vi "btp_work.vi"() -> ()   [LabVIEW 2022 SP3]
uses:
  D:/LabVIEWCodes/USRPPacketTxRx/sub_Chop_Packet.vi
  D:/LabVIEWCodes/USRPPacketTxRx/sub_Ave_Power_And_Thresholding.vi
  D:/LabVIEWCodes/USRPPacketTxRx/sub_Extract_Packet_Boundaries - G.vi
  D:/LabVIEWCodes/USRPPacketTxRx/sub_Extract_Packets.vi
  <vilib>/addons/Modulation/Digital/General/MT Generate PSK System Parameters(M).vi
  <instrlib>/niUSRP/niUSRP Write Tx Data (CDB Cluster).vi
  <instrlib>/niUSRP/niUSRP Fetch Rx Data (CDB Cluster).vi
  D:/LabVIEWCodes/USRPPacketTxRx/subDCOffset.vi
  D:/LabVIEWCodes/USRPPacketTxRx/sub_est_noise_power - G1.vi
  <vilib>/addons/Modulation/niDMT.lvlib
panel:
  out "text 2":string
  out "text":string
  out "standard output 3":string
  out "standard output":string
  out "standard output 2":string
  in  "file (use dialog) 4":path
  in  "file (use dialog) 3":path
  out "standard error 3":string
  in  "file (use dialog) 2":path
  in  "file (use dialog)":path
  out "standard error 2":string
  out "standard error":string
  out "x .or. y?":bool
  in  "synchronization parameters":T1={"expected sync location (symbols)"=-1, "sync sequence"=[], "sync location uncertainty (symbols)"=0, "sync indent (symbols)"=0} {"sync sequence" format="%.2f"}
  in  "Tab Control":T2(tab)=enum."Rx Display"
  in  "Acquisition Duration [sec]":dbl=0.04 format="%#.6p"
  in  "Rx Parameters":T3={"Rx IQ Sampling\nRate [s/sec]"=500000.0, "Rx\nFrequency [Hz]"=915000000.0, "Rx Gain [dB]"=20.0, "Rx Antenna"="RX1"} {"Rx Gain [dB]" format="%#.6p"; "Rx\nFrequency [Hz]" format="%#.6p"; "Rx IQ Sampling\nRate [s/sec]" format="%#.6p"}
  out "Actual Rx Parameters":T3={"Rx IQ Sampling\nRate [s/sec]"=500000.0, "Rx\nFrequency [Hz]"=915000000.0, "Rx Gain [dB]"=20.0, "Rx Antenna"="RX1"} {"Rx Gain [dB]" format="%#.6p"; "Rx\nFrequency [Hz]" format="%#.6p"; "Rx IQ Sampling\nRate [s/sec]" format="%#.6p"}
  out "Symbol Rate\n[symbols/sec]":dbl=62500.0 format="%#.6p"
  in  "Choose a PSK Format":T4(tab)=enum."QPSK" caption="PSK"
  in  "BPSK System Parameters":T5={"Samples per Symbol"=8, "symbol map"=[], "Differential PSK"=enum."disable", "PSK type"=0} {"PSK type" items=["normal", "shifted", "offset"]; "symbol map" format="%.3f"}
  in  "QPSK System Parameters":T5={"Samples per Symbol"=8, "symbol map"=[], "Differential PSK"=enum."disable", "PSK type"=0} {"PSK type" items=["normal", "shifted", "offset"]; "symbol map" format="%.3f"}
  in  "pi/4 DQPSK System Parameters":T5={"Samples per Symbol"=8, "symbol map"=[], "Differential PSK"=enum."enable", "PSK type"=1} {"PSK type" items=["normal", "shifted", "offset"]; "symbol map" format="%.3f"}
  in  "OQPSK System Parameters":T5={"Samples per Symbol"=8, "symbol map"=[], "Differential PSK"=enum."disable", "PSK type"=2} {"PSK type" items=["normal", "shifted", "offset"]; "symbol map" format="%.3f"}
  in  "8-PSK System Parameters":T5={"Samples per Symbol"=8, "symbol map"=[], "Differential PSK"=enum."disable", "PSK type"=0} {"PSK type" items=["normal", "shifted", "offset"]; "symbol map" format="%.3f"}
  in  "16-PSK System Parameters":T5={"Samples per Symbol"=8, "symbol map"=[], "Differential PSK"=enum."disable", "PSK type"=0} {"PSK type" items=["normal", "shifted", "offset"]; "symbol map" format="%.3f"}
  in  "M":i32=4 min=2 step=2
  in  "Custom System Parameters":T5={"Samples per Symbol"=8, "symbol map"=[], "Differential PSK"=enum."disable", "PSK type"=0} {"PSK type" items=["normal", "shifted", "offset"]; "symbol map" format="%.3f"}
  in  "filter parameters":T6={"Alpha"=0.5, "Filter Length"=6, "TX Filter"=enum."Root Raised Cos"} caption="Matching Filter Parameters" {"Alpha" format="%.2f"}
  in  "PN Sequence Order\nfor Sync":i32=31
  in  "Packet Parameters":T7={"Guard Bits "=30, "Sync Bits"=20, "Message Bits"=128, "Number of Packets \nto Expect"=46}
  out "Recovered Message":string="Two roads diverged in a yellow wood,\nAnd sorry I could not travel both\nAnd be one traveler, long I stood\nAnd looked down one as far as I could\nTo where it bent in the undergrowth.\n\nThen took the other, as just as fair,\nAnd having perhaps the better claim,\nBecause it was grassy and wanted wear;\nThough as for that the passing there\nHad worn them really about the same.\n\nAnd both that morning equally lay\nIn leaves no step had trodden black.\nOh, I kept the first for another day!\nYet knowing how way leads on to way,\nI doubted if I should ever come back.\n\nI shall be telling this with a sigh\nSomewhere..."
  out "Received Signal (Raw)":dbl[](graph)
  out "Constellation Graph":T8(graph)=[{"Decimated Array"=[-0.6804993103727607, -0.6771092058245918, -0.6428257187708691, 0.7259219405542873, 0.7311366832454209, -0.6450362325295403, -0.658892442379921, -0.6855840493085356, -0.646998431742077, -0.6568678904388265, 0.7432214399633668, -0.6618522924674632, -0.6753922285302938, 0.6950905811428861, 0.7248141384495557, 0.7218255862492685, 0.704818637196686, 0.7027336696732543, 0.7016253671990413, 0.7082534735709545, 0.7084209330001522, 0.7036372125301554, 0.7010930640613204, 0.7075984577478206, 0.7100058187983528, 0.7171431626733421, 0.7279231861183771, 0.6959557947635676, -0.7024336186443912, -0.7110189818905128, 0.6934234462727887, 0.7327126116070742, 0.7051667045224878, 0.690798979580973, -0.6877839781333666, 0.6889445287579181, 0.716354235720989, -0.706071092371314, 0.72195318833854, -0.7119212984185137, 0.7223509528651848, -0.7244956435522718, -0.6716656585292338, -0.7182056308592257, 0.724421589775866, -0.6763390206227603, 0.7587597202334532, -0.6966306246608392, -0.6999692828092537, -0.7056805503027465, 0.7430994824068496, 0.7108305621069824, 0.7197425435843314, -0.7051937005816177, -0.6734048186040171, -0.6909214820858487, 0.7004218263991402, -0.6889802592692622, 0.7244882842042791, 0.7027757047403482, -0.7012448562483489, -0.6963431828766949, 0.7166197717755273, 0.7431431506248717, 0.7233235134334371, 0.6983161172439467, 0.7059749857271942, -0.6872358926309042, 0.6918268533027474, -0.7138701729016586, -0.6801285945135653, 0.7195044185357663, 0.6810587309328351, -0.6856313040037053, -0.7011043347997452, 0.6920652628903768, -0.7080955978852922, -0.6860253207439192, -0.7101309321759165, 0.7212965033681705, 0.6967245108747491, 0.7128097205123256, 0.6657328144726218, 0.6985573048815797, 0.6967609587320983, 0.720489591403177, -0.6992149062771553, 0.6810319795543738, -0.7124274384065621, -0.6689704942642202, 0.7017697482270308, 0.7036983705130238, -0.69378287602043, -0.6926507402482928, 0.6832891050414109, 0.7219614630178657, 0.7044242088089868, 0.6722056874933439, -0.6818156450864503, 0.6786113633855301, 0.7039257931121476, -0.6836867328922335, 0.6967676536286352, -0.7018627722542645, 0.7033449800412358, -0.7121625353086042], "Decimated Array"=[0.7327573786203745, 0.7417811878517194, -0.6799031648608087, -0.7111421642681004, -0.727382953469249, -0.6704579022356528, -0.6770604606987946, 0.7538529097411865, -0.6722715103438465, -0.6756211416707443, -0.6914774106844375, -0.673529581873597, 0.7393627898718214, 0.7522557788351737, 0.7435736461024193, 0.7257726558576425, 0.7275033865931528, 0.7311828384458046, 0.7293390182016347, 0.7220976758138733, 0.7195981106474233, 0.7211811690986409, 0.7188051788075457, 0.7320183145085448, 0.6962181897094762, 0.7305998791526044, -0.6967382767827438, 0.7159339540668409, -0.7008762468325049, 0.7525668303202456, 0.7058888207208955, 0.7252589385855543, -0.7159704258460882, 0.7370284868429373, 0.7140037167311404, 0.7389767670280546, -0.6960013467696725, 0.7235856630223708, -0.6972846806923089, -0.657884155216942, -0.6949224336608516, 0.7453870445521058, -0.6844918028247094, -0.6835224068604273, -0.7079388773369498, 0.7505384293302241, 0.6958348088594112, 0.7516973279064126, -0.6781015202421304, 0.7276930986154884, 0.7072095654921254, -0.6818066642899347, -0.702124108056222, 0.7365289833752492, 0.7313371097907961, 0.7586596196292686, -0.7079902911617727, 0.713630396728027, -0.7007240447824197, 0.7246614220304907, -0.7064584618733396, 0.7515472341269214, 0.6939391865838809, 0.7190183727683939, -0.6934598211856411, 0.7287398470888085, 0.7237013633767214, 0.7256529739097736, -0.6909901985488635, 0.7147604584382636, 0.6881560723752628, 0.7236976539802175, -0.6922424302133595, 0.7045483839307563, 0.6890103411064745, -0.6887965775506286, -0.7136342940914308, 0.7205719868506776, 0.7023916754066073, 0.7473081616445082, -0.6863264429683489, 0.7186091906642366, -0.7100679145508004, -0.6810878313976068, 0.7293932651728482, 0.722408788035578, 0.7004331018480651, -0.6822150791593455, 0.685337537979504, 0.7132682495621445, -0.6721281174161831, 0.7245443113283739, -0.7431160183824671, 0.7359349670621476, 0.7174344380700259, 0.7431105593701001, -0.6993804544754962, 0.7453566040596344, 0.6929469282521439, 0.7449696798222867, -0.693664788209523, 0.7157173189250563, -0.7183409139718169, -0.6991338441055578, -0.7093747657586275, 0.724868684652829]}, {"Decimated Array"=[-0.6804993103727607, -0.6762349965387238, -0.6685108157798112, -0.6587623289821404, -0.6494739544100483, -0.6438465750011458, -0.645155862498135, -0.6559333949667008, -0.6771092058245918, -0.707329395010057, -0.7427108893571827, -0.7768816274525345, -0.8016064503455926, -0.8078913118575249, -0.7873020181422804, -0.7333876332701184, -0.6428257187708691, -0.5161117575568228, -0.35777203758853365, -0.17570329650700167, 0.01987541369217473, 0.21778298257008183, 0.4072432109758152, 0.5789865397268567, 0.7259219405542873, 0.8433225109633283, 0.9285347773827741, 0.9803625623365572, 0.9983411710644498, 0.9823024312079763, 0.9321501534368272, 0.8480801425231922, 0.7311366832454209, 0.5839247754585907, 0.41126876723240074, 0.2204206478178329, 0.020932943403138903, -0.1761332529377578, -0.3593512576776315, -0.5183227318987554, -0.6450362325295403, -0.7348944300155227, -0.7873580245691122, -0.8057437870339258, -0.7965717988687436, -0.7684407927742708, -0.7306238606226202, -0.6917860656058442, -0.658892442379921, -0.6364690666334113, -0.6263656338128196, -0.6279033391241801, -0.6383295002999582, -0.6535857140497858, -0.6691389263327601, -0.6808303682804338, -0.6855840493085356, -0.6819546232796994, -0.6704727894453094, -0.6535744314745204, -0.6353365462635079, -0.6208696353048802, -0.6154307523642993, -0.6233724286798671, -0.646998431742077, -0.6855864576394015, -0.7347128803667217, -0.7860882541221362, -0.8282453730286534, -0.8479309126781169, -0.8321007406466316, -0.7702787309009056, -0.6568678904388265, -0.4928870454737699, -0.286812316855307, -0.054181947000257816, 0.18398541460571163, 0.403912791430555, 0.5822957160369652, 0.6996654194867074, 0.7432214399633668, 0.7085518372290116, 0.6001271112229511, 0.43028071322686884, 0.21712133759522834, -0.01828477060583316, -0.25486167705907176, -0.474106655260725, -0.6618522924674632, -0.8090041994597156, -0.9113555181844136, -0.9685514235160106, -0.9827395175415803, -0.9572113882143858, -0.8953875269303032, -0.8004356628744611, -0.6753922285302938, -0.5237515103490776, -0.3502005293644506, -0.1611351791820148, 0.03517140208780353, 0.22893110044459927, 0.40972263321669966, 0.5677345648283395, 0.6950905811428861, 0.7869683371034619, 0.8423038906676682, 0.8638849324516561, 0.8577538092414735, 0.8321468933549871, 0.7961070317612736, 0.7580880124868856, 0.7248141384495557, 0.7005277134039959, 0.686923334338586, 0.6833877232132058, 0.6876280888811944, 0.6964899036822818, 0.706747954834772, 0.7157647696850384, 0.7218255862492685, 0.724268969267967, 0.7234261321898535, 0.7202619630220548, 0.7159731242866095, 0.7116890979547664, 0.7082240869885714, 0.70594341514383, 0.704818637196686, 0.7045271958113069, 0.7047088927454438, 0.7050023859293303, 0.7051255773761397, 0.7049541452505861, 0.7044514570052206, 0.7036747950662702, 0.7027336696732543, 0.7017628701423971, 0.7009138948889888, 0.7003118882562483, 0.7000261021126073, 0.7000875017890581, 0.7004449481097869, 0.7009932809698078, 0.7016253671990413, 0.702221540251104, 0.7027618684813808, 0.7032916906181711, 0.7038854962099375, 0.7046487256800136, 0.7056308879137863, 0.7068515417419651, 0.7082534735709545, 0.7096888191782372, 0.7109913402244956, 0.7119894724643936, 0.7124890080936077, 0.7123827414517839, 0.7116323891766451, 0.7102633952930952, 0.7084209330001522, 0.7063057748688335, 0.7042562032788021, 0.7025954190884202, 0.7015546954049546, 0.7012557549487087, 0.7016448259380934, 0.7025398218482226, 0.7036372125301554, 0.7046321819639692, 0.7053295412842902, 0.7055972799037947, 0.705357986716468, 0.7046523984817116, 0.7036068751653552, 0.7023536981462808, 0.7010930640613204, 0.7000326295845363, 0.6993965049981011, 0.6993226127993213, 0.6998881120919372, 0.701113074412268, 0.7029138523453567, 0.7051416575412044, 0.7075984577478206, 0.710078980444559, 0.7123321038850414, 0.7140736603763724, 0.7150314533562983, 0.7150214932752349, 0.7140093308210059, 0.7121877418723002, 0.7100058187983528, 0.70805206355385, 0.7070027727419878, 0.7073212689161522, 0.7091056294101988, 0.7119833987327618, 0.7150644848824459, 0.7171668570713718, 0.7171431626733421, 0.71423133689185, 0.7085192919358748, 0.7011650150275229, 0.6943243914091253, 0.6909299894216554, 0.694045612210552, 0.706066960259486, 0.7279231861183771, 0.7583890909767882, 0.7938021658029275, 0.8279962238841705, 0.8528896550258644, 0.8595701988778817, 0.8395633321459017, 0.7862278633870129, 0.6959557947635676, 0.5689496495122442, 0.4094105630569515, 0.22502717825358973, 0.025894312218078558, -0.17672464042078925, -0.37176542586543576, -0.5495413422869474, -0.7024336186443912, -0.8251771287794907, -0.9146738107129905, -0.9693864660264264, -0.9886486884020281, -0.9721997012143947, -0.920010882437784, -0.8324905468768208, -0.7110189818905128, -0.5586215402038113, -0.38057133580870495, -0.18461757845785642, 0.019294891934465676, 0.2197963582992338, 0.4053691867674974, 0.5657713716359056, 0.6934234462727887, 0.7843501298361789, 0.8386729718179944, 0.8602628823550353, 0.855774513907276, 0.8333154686311419, 0.8010170366525857, 0.7658225991667146, 0.7327126116070742, 0.7045406905991981, 0.6824916000019303, 0.6667964864918056, 0.6575588911889615, 0.6553991485314229, 0.6616300661715835, 0.677865934701111, 0.7051667045224878, 0.7429233296416752, 0.7878677137961015, 0.8333853282559609, 0.8696348770191419, 0.8846190114381185, 0.8659756375138661, 0.8033400824826783, 0.690798979580973, 0.5288571353054295, 0.32551133007737276, 0.09595098720473762, -0.13906888290440567, -0.35588344294942403, -0.5312979803398246, -0.646084108275294, -0.6877839781333666, -0.6524636145322816, -0.5450893812430798, -0.37828756856953233, -0.17009276356333847, 0.0590247558982818, 0.28912715162217667, 0.5032762839933951, 0.6889445287579181, 0.8383428746399739, 0.9477025130341128, 1.015790170453614, 1.0423483901645878, 1.0268512388275022, 0.9680879161655901, 0.8646551393981081, 0.716354235720989, 0.5260764152807655, 0.30160439840294034, 0.05668512406955431, -0.18910351581760784, -0.4118751751084471, -0.5863423085037114, -0.6897554505434935, -0.706071092371314, -0.6295185621493208, -0.4668637151478481, -0.23765972556227086, 0.027714817455610417, 0.29202447870753795, 0.5167154122972588, 0.6679084709283569, 0.72195318833854, 0.6695114009171929, 0.5175155629675429, 0.2883041299697019, 0.01623720013151288, -0.25755900242514196, -0.4917082138253101, -0.6510176327160702, -0.7119212984185137, -0.6659995880876536, -0.5209852917537516, -0.2992839322286186, -0.03416997277404838, 0.2355466281568285, 0.4714352113659737, 0.6410442893752866, 0.7223509528651848, 0.7062991907811851, 0.5973003486423586, 0.4116890808688979, 0.17445466790696096, -0.08489625696410336, -0.3368901331962952, -0.5561324114364461, -0.7244956435522718, -0.832904063982776, -0.8817003370505312, -0.8795283892255058, -0.841156501109088, -0.7846263716950196, -0.7281214416972949, -0.6870445779683771, -0.6716656585292338, -0.6855631019709484, -0.7251869491105687, -0.7803544807713914, -0.8357414937022205, -0.8732615963603204, -0.8749681769421048, -0.8261602248386887, -0.7182056308592257, -0.5506938062457699, -0.3325933377055765, -0.08189760414583691, 0.17618237159000388, 0.4123697444728759, 0.5974694739328056, 0.7068084628379865, 0.724421589775866, 0.6461724854013321, 0.4812775786848407, 0.25159361606242997, -0.011058078343011023, -0.2692923486046545, -0.48569025029571594, -0.6284581525739953, -0.6763390206227603, -0.6219818356022658, -0.47306441806801147, -0.2510857990405568, 0.01202477775150253, 0.27875734553572085, 0.5116930035471384, 0.6789865139576629, 0.7587597202334532, 0.7418192787585248, 0.6323458533022597, 0.446406792743502, 0.20878035238051276, -0.05119783320575381, -0.3042611875270661, -0.5253152667965498, -0.6966306246608392, -0.8095606744479041, -0.8647740627418172, -0.870930075780708, -0.8423384959975685, -0.7960318277718325, -0.7486596019303445, -0.7137982795070836, -0.6999692828092537, -0.7095971091381883, -0.7390816485119921, -0.7796138336185289, -0.818762813999536, -0.8425904879324037, -0.8378822227707572, -0.7942341058424417, -0.7056805503027465, -0.571726769560303, -0.39765177441111643, -0.19391837432237818, 0.025178720377377686, 0.24333379676657457, 0.44433965307888695, 0.6142375047967751, 0.7430994824068496, 0.8263038750024307, 0.8650100488333368, 0.8657148042767202, 0.8390794723757462, 0.7981161813167071, 0.7560954579232749, 0.7244176046468488, 0.7108305621069824, 0.718204650734365, 0.7441150394580835, 0.7812106743682087, 0.8183931962770272, 0.8425254654823089, 0.8406177118076219, 0.8019301699596733, 0.7197425435843314, 0.5926686710089698, 0.4251140503775492, 0.22683136067452989, 0.011660330280988253, -0.20423795622266205, -0.4045792942890271, -0.57504838691632, -0.7051937005816177, -0.7897661684393493, -0.8293068652572223, -0.8299006515155186, -0.8021229049955473, -0.7594233513128958, -0.715953221878639, -0.684307426439313, -0.6734048186040171, -0.6868570522140265, -0.7221874426788824, -0.7708237442647581, -0.8191585903691571, -0.8505818015508355, -0.8481661462885941, -0.7977634650762118, -0.6909214820858487, -0.5271825682100394, -0.31525436879598623, -0.07267661804829456, 0.17610311762416703, 0.4028796348907104, 0.5798206568779839, 0.6838352068807156, 0.7004218263991402, 0.6263585027788804, 0.4707037347107586, 0.2537801245269521, 0.004363575376446024, -0.244425088845282, -0.45988451941533137, -0.6143614233710846, -0.6889802592692622, -0.675810131006379, -0.5782280367437729, -0.40962067096108434, -0.19054676255841746, 0.05481291967260732, 0.3023001215109928, 0.5308329677888366, 0.7244882842042791, 0.8734246012838044, 0.9735701497284382, 1.0253939516322779, 1.0322709072595566, 0.9989018615889086, 0.9300855209250758, 0.8301278260930205, 0.7027757047403482, 0.5516545283139476, 0.38091449347590134, 0.19570631362414656, 0.002354352790910658, -0.19179798997086855, -0.3788570549590451, -0.5510272450358933, -0.7012448562483489, -0.8236915392774603, -0.914039706142418, -0.9694184170252935, -0.9881756409826234, -0.9696303075716558, -0.913918517626886, -0.8220829857364051, -0.6963431828766949, -0.5405016807251724, -0.36031892603430715, -0.16359224329210514, 0.04013418091790215, 0.24018456190270834, 0.425760423266114, 0.5870829268985424, 0.7166197717755273, 0.8099833426954562, 0.8664917523906949, 0.8890606065456064, 0.8835329376488369, 0.8577948250420299, 0.8205354221662687, 0.7800304020582047, 0.7431431506248717, 0.7146443568705966, 0.6969512334183051, 0.6901074157262647, 0.6922880175560046, 0.7003398356906728, 0.7105226229352982, 0.7191652725013788, 0.7233235134334371, 0.7213381284523223, 0.7131072858574705, 0.7002046822080928, 0.6857438943908143, 0.6739876200747604, 0.6696394639541572, 0.6768836675096863, 0.6983161172439467, 0.7338690127516884, 0.7800774899548244, 0.829602819630056, 0.8715371312486556, 0.892620000492053, 0.8790856399483223, 0.8192212166031462, 0.7059749857271942, 0.5391749210900726, 0.3269503040314498, 0.08573815461541592, -0.1612255824786287, -0.386730293143399, -0.5635326559438285, -0.6686383256247854, -0.6872358926309042, -0.6156114857935734, -0.4623211423735695, -0.24733010394610414, 0.0007198102460047476, 0.24863863484628498, 0.4635514254715547, 0.6176104623364325, 0.6918268533027474, 0.6782756201030052, 0.5805134425392992, 0.41210610757403726, 0.19372452237290802, -0.050391409713054024, -0.29611210645789393, -0.5225111093000552, -0.7138701729016586, -0.8605441211993027, -0.9585448112667802, -1.008414026021156, -1.0135648241052666, -0.978745896542667, -0.9087849082692102, -0.8079881948321259, -0.6801285945135653, -0.5287862221062773, -0.35805233939202374, -0.1729861888667504, 0.020116186161511587, 0.21387335563181437, 0.40025748153323093, 0.5712472743319003, 0.7195044185357663, 0.8388895884119506, 0.9249072134737321, 0.9746853929178996, 0.9868923875604191, 0.9616684243967665, 0.9003848901697228, 0.8056175444681817, 0.6810587309328351, 0.5314881726723011, 0.3626554692436761, 0.18103860407685468, -0.006510589607727805, -0.1931114704827839, -0.3722848897831801, -0.5381718770034626, -0.6856313040037053, -0.8101801487665511, -0.9076732803716326, -0.9739618526107378, -1.004716020345832, -0.9956414793795033, -0.9430154749490675, -0.8446500281072215, -0.7011043347997452, -0.516842399364099, -0.3010204717594881, -0.06763754580789842, 0.16514820448340978, 0.37668157665933155, 0.5461920463765456, 0.655552915260347, 0.6920652628903768, 0.6505655304034257, 0.5346883243834851, 0.35661897243093144, 0.13559774776324776, -0.1046718797566402, -0.3394032573081613, -0.5461789593962133, -0.7080955978852922, -0.8157954529602021, -0.8683801331865292, -0.8727983131028657, -0.8421078226859732, -0.7927582081222804, -0.741572331068595, -0.7028423018527019, -0.6860253207439192, -0.6943551977069015, -0.7245345157854167, -0.7675646042411391, -0.8104296201087327, -0.8383601072014226, -0.8373952185694984, -0.7966528302359737, -0.7101309321759165, -0.5776984378988999, -0.40521323182553737, -0.2036592543667804, 0.012419924984258368, 0.22695341747885692, 0.42449093142276867, 0.592188438033417, 0.7212965033681705, 0.8079364234726191, 0.8532668165288172, 0.8627953034872611, 0.8451288060001957, 0.8104079963441455, 0.7687359339278867, 0.7287670505538517, 0.6967245108747491, 0.6759780606536095, 0.667107406232625, 0.6684364317450245, 0.676784919616326, 0.6884291860003884, 0.699890853611944, 0.7085144901744879, 0.7128097205123256, 0.7124229876828518, 0.7080187790236897, 0.7008050101089057, 0.6921805709227881, 0.6834646736814466, 0.6757033963031507, 0.669648508318143, 0.6657328144726218, 0.6642652636337992, 0.6653767657521718, 0.6690028595853793, 0.674775333959487, 0.6819477949985021, 0.6893278789128267, 0.6953927726157616, 0.6985573048815797, 0.697578095425808, 0.6920506573747554, 0.6828307951888688, 0.6722732265164824, 0.6640958466160822, 0.6627912256868634, 0.6726965874495441, 0.6967609587320983, 0.735252994349721, 0.7847852487718341, 0.837860611588047, 0.8832021671865116, 0.9070282265831913, 0.8950883370622812, 0.8352994933427401, 0.720489591403177, 0.5506306635171825, 0.3342725070105252, 0.08840692523651153, -0.16315427404215097, -0.3926718560799536, -0.572539734272038, -0.6796338477180948, -0.6992149062771553, -0.6277630208203462, -0.4741131473050659, -0.2585293695095081, -0.009930257048617025, 0.23830892263310452, 0.45325402085890604, 0.607121618765611, 0.6810319795543738, 0.6672310461853316, 0.5694827757707117, 0.4015147931896041, 0.1841817171712272, -0.05817646638242799, -0.3014136753019013, -0.524665532969832, -0.7124274384065621, -0.855285246094759, -0.9495933688767533, -0.996236130847489, -0.9989838487955423, -0.9628841324499167, -0.8930056180780918, -0.7937877561121499, -0.6689704942642202, -0.5220072798874036, -0.3566099133872175, -0.17731129436958973, 0.010268861422383327, 0.19945198638565087, 0.3827826926443024, 0.5526251582270405, 0.7017697482270308, 0.8239876507426606, 0.9144785689512498, 0.9699591512942685, 0.9886252045487814, 0.9700306803372667, 0.9149020439452162, 0.825116863065968, 0.7036983705130238, 0.554839481392563, 0.3840291620621759, 0.19787647745423148, 0.003860727052948984, -0.18999525295737457, -0.3757044734833313, -0.5458056810042837, -0.69378287602043, -0.814366828718361, -0.9036469275456485, -0.9588849469775574, -0.9783006504455267, -0.960973889608092, -0.9067746467203663, -0.8165903751017708, -0.6926507402482928, -0.5388812935652539, -0.361228905014989, -0.16771060388912773, 0.031903370124330505, 0.22678679843602859, 0.4061707941853134, 0.5606402717569381, 0.6832891050414109, 0.7705901219032752, 0.8228006526178891, 0.8436430103344122, 0.8394755303225311, 0.8180394512925253, 0.7871333265278456, 0.7534665911565442, 0.7219614630178657, 0.695510686451852, 0.6753252498343544, 0.6615878037807406, 0.6542998195364643, 0.6538606147644473, 0.6612723675386262, 0.6778625191525914, 0.7044242088089868, 0.7402649399766673, 0.7822594926239343, 0.8241634231439008, 0.8566831085547093, 0.8684082810681567, 0.8475040183712003, 0.784012885063017, 0.6722056874933439, 0.5125005393952523, 0.31260026449095785, 0.08722135068631567, -0.14339658857823498, -0.35611765704885123, -0.5282733760242059, -0.6409441045045646, -0.6818156450864503, -0.6469272017629891, -0.5410574986904879, -0.37652152921039295, -0.17097947697100876, 0.05541171165914345, 0.2829619347828144, 0.49484727767121917, 0.6786113633855301, 0.8264573551553331, 0.9345361200971587, 1.0015661687984379, 1.0272888190262575, 1.0112965146842847, 0.952583288738177, 0.8500890658990591, 0.7039257931121476, 0.5171900515296706, 0.29764273007471115, 0.05870661463653025, -0.1806017914741214, -0.39721826601913907, -0.5668036345777544, -0.6674573482841338, -0.6836867328922335, -0.6099467963750959, -0.4528161959244535, -0.23123780147788525, 0.0254037230819288, 0.2810884215045038, 0.4984727203603391, 0.6447055580185417, 0.6967676536286352, 0.6455398584402634, 0.4976568874522828, 0.2746594289249686, 0.009825427460916032, -0.25698435822392646, -0.4855514161032739, -0.6415528231225354, -0.7018627722542645, -0.6580125604775775, -0.517265265222927, -0.30121265695938104, -0.04212438479079229, 0.22217065809727116, 0.45405673442103006, 0.6217149465148919, 0.7033449800412358, 0.6897787566619501, 0.5850104229528822, 0.4047415306155254, 0.17323834921239678, -0.08075812096424864, -0.3284327261412435, -0.5448733152596168, -0.7121625353086042, -0.8211818337976253, -0.8719691969355644, -0.8727186157199347, -0.8376486334880819, -0.7842590106698991, -0.7303274268398209, -0.6909814362358659], "Decimated Array"=[0.7327573786203745, 0.8571160437398065, 0.9481227692632541, 1.003980881033979, 1.0238155370523472, 1.0072368286759465, 0.9541994905916551, 0.8651912730450063, 0.7417811878517194, 0.5871636451740783, 0.40676677760888635, 0.20846130324205578, 0.0022318875001048045, -0.2005410967663612, -0.38829860023304064, -0.5506845398656813, -0.6799031648608087, -0.7716987861234258, -0.8258475294329478, -0.8459996756657396, -0.8388616433189412, -0.8130753155007096, -0.7778435482452709, -0.7416372990136377, -0.7111421642681004, -0.6905831950739342, -0.6815454430666558, -0.6831516021872707, -0.6925669267273694, -0.7057731727702966, -0.7184007879882285, -0.7265282476091678, -0.727382953469249, -0.7198001905615271, -0.7045629848520147, -0.6843705475932246, -0.6634185556136458, -0.646887119577886, -0.6400361359583534, -0.6471594714631548, -0.6704579022356528, -0.7090564063186768, -0.7584053880552923, -0.8101244036157627, -0.8526189235085075, -0.872417498261418, -0.8561767863823757, -0.7930533916017833, -0.6770604606987946, -0.5089375701527854, -0.2971550620890392, -0.05761269204799846, 0.18789151496970918, 0.4143336303799478, 0.596919125262307, 0.7147087986695557, 0.7538529097411865, 0.7097353627437273, 0.5877778836770051, 0.40257278286196346, 0.1755748921605498, -0.06817834720063913, -0.30381917292160493, -0.5101473732591594, -0.6722715103438465, -0.782942771822579, -0.8426075541528982, -0.8581499860345086, -0.8406550377330191, -0.8028915815603971, -0.7569445207502417, -0.7124441110679234, -0.6756211416707443, -0.6492985792878058, -0.6336104831921037, -0.6270868628284776, -0.6278993868440812, -0.6347460148648578, -0.6473189374357599, -0.6660652122000107, -0.6914774106844375, -0.7231297220029862, -0.7587664029448702, -0.7936544758660282, -0.8205522923344901, -0.8305429506490288, -0.8142884856193261, -0.7636823212203829, -0.673529581873597, -0.5429181777841331, -0.3758793938755062, -0.18113858110834186, 0.028812354472331908, 0.23939310934756888, 0.4359274511900307, 0.6056519046787863, 0.7393627898718214, 0.8324327306148087, 0.8851319247653551, 0.9020886016493107, 0.8911142062914292, 0.8617307665544903, 0.8235701121823792, 0.7850172209229723, 0.7522557788351737, 0.7288635601528786, 0.7158958847588804, 0.7123277223581522, 0.715761845721655, 0.7231900323302534, 0.7316880970831603, 0.7389528359720056, 0.7435736461024193, 0.7451046063677472, 0.743901281226759, 0.740788821822152, 0.7367782401995692, 0.7328033193551644, 0.7294981194191762, 0.7271513904156902, 0.7257726558576425, 0.725159941446078, 0.725060989178965, 0.7252632377419967, 0.7256163395829798, 0.7260606904500417, 0.7265379023034586, 0.7270291732601397, 0.7275033865931528, 0.7279199682707127, 0.7282769079854728, 0.7285974590770533, 0.7289407767207793, 0.7293428506461535, 0.7298479408102396, 0.7304778513692572, 0.7311828384458046, 0.7318265401385785, 0.7323028750384627, 0.7325567749966301, 0.7325033028493253, 0.7321158823152807, 0.7314068004824351, 0.7304533892028899, 0.7293390182016347, 0.7281572743585262, 0.7270606197087242, 0.7261241067000211, 0.7253508195631971, 0.7246697616263047, 0.723969429286671, 0.723139564739256, 0.7220976758138733, 0.7208555865072881, 0.719568292828321, 0.7184478733558384, 0.7176993275862744, 0.7174622207349447, 0.7177521937986072, 0.718516228428159, 0.7195981106474233, 0.7207879819353863, 0.7218924194293399, 0.7227111613943498, 0.7231168859595661, 0.7230786498664554, 0.7226411424851807, 0.7219463720454906, 0.7211811690986409, 0.7204810710907097, 0.7199538718599565, 0.7196320372423504, 0.7194607411817737, 0.7193099127963588, 0.7190971249818399, 0.7188635612803779, 0.7188051788075457, 0.7192369464355841, 0.7205351477714964, 0.7229401499987833, 0.7263486481418566, 0.7301617369824043, 0.7333271712095472, 0.7344308070476105, 0.7320183145085448, 0.7250816880667706, 0.7135657369657201, 0.6987104127947069, 0.6831567860992641, 0.6708043964638186, 0.6662258399732381, 0.6737496016563864, 0.6962181897094762, 0.7338123953236427, 0.7831464621140352, 0.8367458472751513, 0.8833813981307604, 0.9091987678800104, 0.8998091259693833, 0.8428401153753142, 0.7305998791526044, 0.562507495226734, 0.34659814194077, 0.0995702257773744, -0.15462281131582128, -0.3875977492359962, -0.5706271624637833, -0.6790839949047796, -0.6967382767827438, -0.6189803271815245, -0.4544562375583789, -0.22459908414379984, 0.03903553601854455, 0.29916696405087967, 0.5182679460830586, 0.6643639077354586, 0.7159339540668409, 0.6652943920234429, 0.5198749673865217, 0.300993470244488, 0.04051717061424443, -0.22409581460784916, -0.45544556602126973, -0.6216785191074483, -0.7008762468325049, -0.6837610820977862, -0.5742886326760264, -0.3883111156265534, -0.1505286326662823, 0.10967239939698414, 0.3627475020866999, 0.5831487815378037, 0.7525668303202456, 0.8617987081334637, 0.9111768991603971, 0.9094611758407977, 0.8715862070139058, 0.8157455416667302, 0.760202018310825, 0.7202658930923688, 0.7058888207208955, 0.7201847936946834, 0.759052366114439, 0.811812333812609, 0.8630070563777121, 0.8948697888398245, 0.8903643946442023, 0.8361831300618912, 0.7252589385855543, 0.5584821670091451, 0.345315670477598, 0.10299763765352206, -0.14547539122840722, -0.37428698339337824, -0.5583637418127292, -0.6768312337753024, -0.7159704258460882, -0.6711625159308375, -0.5476542552431498, -0.3597709705436185, -0.1287724532856077, 0.12018518168690656, 0.36151984386717273, 0.572699142103299, 0.7370284868429373, 0.8455964386542135, 0.8979126579643226, 0.9012807607635166, 0.8690744380604796, 0.8181990426007191, 0.7661088030574076, 0.7279245613823432, 0.7140037167311404, 0.7282038712248695, 0.7671972819282604, 0.8208631561250372, 0.8738564756136162, 0.9080475656744531, 0.9055112204914009, 0.8518434216042863, 0.7389767670280546, 0.5673122043840576, 0.346672036977057, 0.09563946895916749, -0.1604955961723308, -0.3929887785452873, -0.573731438794397, -0.6795623772004052, -0.6960013467696725, -0.619916032405668, -0.46047605211853976, -0.238293779549608, 0.017302276506560462, 0.2723050965454336, 0.4928472153853533, 0.6499682346772773, 0.7235856630223708, 0.7050531042870595, 0.5980296925245243, 0.4173625434472803, 0.18635581949974522, -0.06697296685650257, -0.3141616680583659, -0.5303108718258116, -0.6972846806923089, -0.805693295562243, -0.8554610680619644, -0.8548810350527455, -0.8184903429533198, -0.7641725094683359, -0.7100008771843999, -0.671228658984871, -0.657884155216942, -0.6731679025330721, -0.7131015741595147, -0.7671687462263975, -0.8200654189127506, -0.8542004537564716, -0.8526249939936517, -0.8019646550151107, -0.6949224336608516, -0.5320250473508275, -0.32225185034324333, -0.08237582607009868, 0.1650026835738332, 0.39428466394542017, 0.5803342409591474, 0.7020686940954762, 0.7453870445521058, 0.7052505477960299, 0.5864589514160631, 0.40293010537214813, 0.17562748086081167, -0.0704552502607787, -0.309822690701368, -0.5200321703524325, -0.6844918028247094, -0.7944039739927944, -0.849369247148433, -0.856656043797114, -0.8292787623167311, -0.7833804658452638, -0.7353387812407823, -0.6989933350482087, -0.6835224068604273, -0.6921158238785066, -0.7217188264252835, -0.7637517506720419, -0.8057159017858148, -0.8333093620537693, -0.8327870038627241, -0.7931510688939891, -0.7079388773369498, -0.5762895149017982, -0.4032287101039275, -0.19912345762738048, 0.021626092972811716, 0.24243838454530214, 0.4466281803126936, 0.6195670275196116, 0.7505384293302241, 0.8341667424696944, 0.8710515511074273, 0.867618588313726, 0.8350546605288388, 0.7875968290108912, 0.7403153596554869, 0.7065887377614032, 0.6958348088594112, 0.7117510991794384, 0.7514265747295997, 0.8055501080993405, 0.8597172027233948, 0.896672112950365, 0.8992716440220376, 0.8535956532880161, 0.7516973279064126, 0.5935739768219647, 0.3879409425761628, 0.1514795080598367, -0.09323685375808283, -0.32079142716179476, -0.5065138588773618, -0.6300491223171335, -0.6781015202421304, -0.64619431762589, -0.5389832779795898, -0.36913308344851997, -0.15510153259215717, 0.08166236993095077, 0.3196509591252603, 0.5398927777919778, 0.7276930986154884, 0.8734985979773947, 0.9728047077610658, 1.0252642302363124, 1.0333899494712895, 1.0012329554745556, 0.9333027118497857, 0.8339401572384909, 0.7072095654921254, 0.5571462896311223, 0.3881483450425459, 0.20534155782487487, 0.01482887737245796, -0.1764521290488, -0.3611157500299354, -0.5318043493520626, -0.6818066642899347, -0.8054524101831724, -0.8983255342414102, -0.9572814410830893, -0.9802961943453828, -0.9661962276209902, -0.9145882909024544, -0.8259958203690237, -0.702124108056222, -0.5463111553516156, -0.3640099142702318, -0.1630068815984123, 0.04665386649189137, 0.25324056756651203, 0.4443960991039263, 0.6085609531447825, 0.7365289833752492, 0.8228996922007434, 0.8670933837874918, 0.8736111453366721, 0.8515289789816484, 0.8132403002190881, 0.772465080941647, 0.7419679771548864, 0.7313371097907961, 0.7450271466496866, 0.7811915546642222, 0.8315498322037654, 0.8823689588265033, 0.9165305921773814, 0.9163401501954511, 0.866798433796903, 0.7586596196292686, 0.5908492722170399, 0.37178062020046765, 0.11907890680745346, -0.14211821683680798, -0.38238233257874527, -0.5721392733995939, -0.6862057323913836, -0.7079902911617727, -0.6327143381258475, -0.4689575875843263, -0.23816585088733142, 0.02788728184520496, 0.2913733998865506, 0.5138745348418566, 0.6622161891528019, 0.713630396728027, 0.6595409016687056, 0.5072353110800646, 0.2790535214186103, 0.009173689804918802, -0.26151320666451255, -0.49168518087347146, -0.646028784822539, -0.7007240447824197, -0.6471884427151815, -0.493530539618674, -0.2632018631271933, 0.008643095196815533, 0.28067049342689865, 0.5117662020698565, 0.667360375596674, 0.7246614220304907, 0.6758948089830248, 0.5292499968474088, 0.30723953882700833, 0.04292589220225078, -0.22522884697938184, -0.4592044373314265, -0.6269083921942394, -0.7064584618733396, -0.6888404338934664, -0.578411648288706, -0.39139022626549447, -0.15271914914807735, 0.10811456934185323, 0.36154443524920665, 0.5821113615057549, 0.7515472341269214, 0.8606474547165524, 0.9096953707888916, 0.9073268916916939, 0.8684122594374747, 0.8110629523849187, 0.7535131577918508, 0.7111116174600383, 0.6939391865838809, 0.7053500144234236, 0.7415364458091326, 0.7922663020024436, 0.8425535702269459, 0.8751141872059586, 0.8732034679792344, 0.8235993150699542, 0.7190183727683939, 0.5598342988350936, 0.3547305255173707, 0.12000835651727722, -0.12227364288086777, -0.34712620885755746, -0.5299758484536152, -0.6500817333967435, -0.6934598211856411, -0.6548680069310724, -0.538631179832801, -0.35797405653961106, -0.13314154269390344, 0.11150249461783546, 0.3507932103438662, 0.5622006640712187, 0.7287398470888085, 0.8409123226340982, 0.8975410491756267, 0.9052474392037568, 0.8767801125750505, 0.8285828512227308, 0.7778392815717208, 0.7394654445105879, 0.7237013633767214, 0.7343864257619723, 0.7683602106205176, 0.8160146443370595, 0.862832671453382, 0.8918135732392275, 0.8863825849799384, 0.8334021521345413, 0.7256529739097736, 0.5635985512953553, 0.35608386653185525, 0.1195604135723027, -0.12374840459859741, -0.3487502236997944, -0.5308687349642771, -0.6495113130900928, -0.6909901985488635, -0.6504937240912037, -0.5328353201969774, -0.3517349807169625, -0.12783984379196844, 0.11423012543166067, 0.3492730631198282, 0.5549865684462535, 0.7147604584382636, 0.8196924285734603, 0.8692925730239803, 0.8708584840188425, 0.8377913064207088, 0.7870129074549828, 0.7359765930553231, 0.6996793525556969, 0.6881560723752628, 0.7048218776482567, 0.7458257319106636, 0.8006775631265496, 0.853917719961837, 0.8877440401214893, 0.8850693181898429, 0.8326613733709883, 0.7236976539802175, 0.5594490106415803, 0.3497538967519691, 0.11201578047048573, -0.13100695912350224, -0.3542636347146736, -0.5338912711941378, -0.6506028489493497, -0.6922424302133595, -0.6552909494544218, -0.545064832644278, -0.37448254797377645, -0.16191455440330382, 0.07162348789175096, 0.305307696187205, 0.5209397804835978, 0.7045483839307563, 0.8471495500869136, 0.9446334649114675, 0.9967359029755237, 1.0058177131022314, 0.9755714551521117, 0.910087443335543, 0.8133163625595331, 0.6890103411064745, 0.5410140712172831, 0.37367966894661164, 0.19222351735516607, 0.002885008671315868, -0.18723164421141011, -0.3706358231842831, -0.540017664941237, -0.6887965775506286, -0.811456181705438, -0.9037768968384509, -0.9627749707154154, -0.986428591882344, -0.9734798839005043, -0.9233425758887451, -0.8362626385273748, -0.7136342940914308, -0.5585921807071323, -0.37653877807456615, -0.17539608244694269, 0.03449829302119377, 0.24108409799518699, 0.4317114568156308, 0.5946337468390553, 0.7205719868506776, 0.8042233087437884, 0.8452649724027359, 0.8485537347599877, 0.8236121116636361, 0.7832470748996688, 0.7415340851598169, 0.7114139852567443, 0.7023916754066073, 0.7186444625002776, 0.7579146977658392, 0.8114788518364714, 0.865212362785649, 0.9017186145139675, 0.9031789704236397, 0.8546836474975438, 0.7473081616445082, 0.5805118731598218, 0.3633604703375262, 0.11403099657073672, -0.1421571689009856, -0.376100265224383, -0.5591208341865042, -0.66748156416295, -0.6863264429683489, -0.61238919788703, -0.45495950013783854, -0.2348765682622349, 0.018329318180048494, 0.27072256893627067, 0.4888669989484364, 0.6445441082266234, 0.7186091906642366, 0.7032516717681991, 0.602286440359839, 0.4297305321288512, 0.20693427048046936, -0.04118448970582595, -0.2899486028515708, -0.51813884111226, -0.7100679145508004, -0.8564812364022516, -0.954078154354838, -1.004051301932304, -1.0102212014763818, -0.9772535580383042, -0.9093646718646989, -0.8097976595431309, -0.6810878313976068, -0.5258335391357575, -0.34780340225624445, -0.15283789222057037, 0.05073422541995442, 0.25233190333965977, 0.44007238959276546, 0.6022906295601135, 0.7293932651728482, 0.8155001380288734, 0.8596440510683021, 0.8661244160018878, 0.8440053760191001, 0.8057116144877121, 0.7648934322393982, 0.7341019522530025, 0.722408788035578, 0.7335846743805764, 0.76523665163658, 0.8088069415554398, 0.8508057382972929, 0.8750784439185956, 0.8656525197192184, 0.8097364952043214, 0.7004331018480651, 0.5385134797346247, 0.333020638982082, 0.10055243220663874, -0.13684916712333142, -0.3547046170347631, -0.5296187059445376, -0.6427036804094352, -0.6822150791593455, -0.6450059416608724, -0.5366580259087476, -0.37013892662339776, -0.16344566761793425, 0.06325834047144631, 0.29051687792880865, 0.5019090102948002, 0.685337537979504, 0.8332571783100664, 0.9419059935710599, 1.0099338897337269, 1.0368536824281052, 1.0219112826998396, 0.9637216757298569, 0.8608644035958495, 0.7132682495621445, 0.5240958995354725, 0.30150783203128084, 0.05962244367312289, -0.18169903701790627, -0.3985650165893692, -0.5660874768283738, -0.6622779885806316, -0.6721281174161831, -0.5910217986061128, -0.4267122427659796, -0.19931344093386746, 0.06087906417721856, 0.31748163584889194, 0.5333437531858058, 0.6763479522156483, 0.7245443113283739, 0.6697558890344962, 0.5190710655465737, 0.2937181748767438, 0.02576020244976748, -0.24681249668741956, -0.4858948596428177, -0.6588635605451997, -0.7431160183824671, -0.7289134552508003, -0.6200694296515479, -0.4325067812603366, -0.19121024572221312, 0.07400166309693594, 0.3330849816678037, 0.5599873834891823, 0.7359349670621476, 0.8513661111199331, 0.9063246869034065, 0.9094064046484032, 0.8755054075051303, 0.8228032542069148, 0.7695512733800192, 0.7310864566365781, 0.7174344380700259, 0.7318771929311987, 0.770521492507058, 0.8229990169861556, 0.8741669857800006, 0.9065945000702298, 0.9034290410951017, 0.8513488075060012, 0.7431105593701001, 0.5792771762670239, 0.3688585907869233, 0.12855873457058717, -0.11905374155741394, -0.348465451110149, -0.5346000660767498, -0.6563026294503328, -0.6993804544754962, -0.6586232637177873, -0.5386587210945445, -0.35325412329016936, -0.12340944757935825, 0.12562838916868907, 0.3678984527083349, 0.5802535686096911, 0.7453566040596344, 0.8536797217461267, 0.904341743696613, 0.9045288934223483, 0.8678005605218305, 0.8115232656672823, 0.7538338251356304, 0.7106289265654393, 0.6929469282521439, 0.7051665302164144, 0.7441987520198292, 0.7999632255413621, 0.8568697593576841, 0.8963183241181077, 0.8998019936252488, 0.8522424023181564, 0.7449696798222867, 0.5778551163588856, 0.3603125530553699, 0.11070054945898282, -0.14570230635299203, -0.3799809948767624, -0.5637043781173343, -0.6732548027150764, -0.693664788209523, -0.6213306289901542, -0.46505052769065697, -0.24516543111583403, 0.0090596915946915, 0.2635428251223252, 0.48417637041829653, 0.641689526437302, 0.7157173189250563, 0.6973828411174359, 0.5901314098610099, 0.4086428546496129, 0.17619718572689294, -0.07917988137166046, -0.328937783780878, -0.5480728892646238, -0.7183409139718169, -0.830216292312652, -0.8834929518448947, -0.8862829283786646, -0.8529835994516479, -0.8013536812216641, -0.7493136237212195, -0.711957955660661, -0.6991338441055578, -0.7139427031909754, -0.7523268372875261, -0.8037761996631599, -0.8530893578229929, -0.8828792296977179, -0.8764987725251604, -0.8209490836280732, -0.7093747657586275, -0.5427215391631399, -0.33033331822457584, -0.08916763854378294, 0.15803966171501063, 0.3856904000524847, 0.5687642313471672, 0.6864040238926279, 0.724868684652829, 0.6795420414253549, 0.5557211678730963, 0.3677696222282419, 0.13706564016321376, -0.11113892216576668, -0.3513165038596046, -0.5611655218564168]}]
  out "Sync Found":bool=TRUE
  out "Correct Packets Rx":i16=46
  out "Singal & Noise Power":cluster{"signal_power":dbl, "noise_power":dbl}={"signal_power"=0.000719802679436105, "noise_power"=8.71918670194843e-09}
  out "error out":errorcluster
  out "Cumulative Packets Recovered":i16(graph)=46
  out "Signal and Noise Power Tracking":cluster{"total_power":dbl, "noise_power":dbl}(graph)={"total_power"=0.000719802679436105, "noise_power"=8.71918670194843e-09}
  in  "stop":bool
  out "Symbol Rate\n[symbols/sec] 2":dbl=25000.0 format="%#.6p"
  out "Constellation Graph 2":T8(graph) caption="Constellation Graph"
  in  "autoscale":bool
  in  "Tab Control 2":T9(tab)
  in  "Packet Parameters 2":T10={"Guard Bits "=30, "Sync Bits"=20, "Message Bits"=128}
  in  "Packet Pad \n[samples]":i32=200
  in  "Blank Frame \n[samples]":i32=500
  out "Number of Packets in Message":i32=46
  in  "PN sequence order\nfor Sync Bits":i32=31 caption="PN sequence order (9)"
  in  "Packet Repeat":i32=2
  in  "Select PSK Modulation Format":T4(tab)=enum."QPSK" caption="PSK"
  in  "BPSK System Parameters 2":T5={"Samples per Symbol"=8, "symbol map"=[], "Differential PSK"=enum."disable", "PSK type"=0} caption="BPSK System Parameters" {"PSK type" items=["normal", "shifted", "offset"]; "symbol map" format="%.3f"}
  in  "QPSK System Parameters 2":T5={"Samples per Symbol"=8, "symbol map"=[], "Differential PSK"=enum."disable", "PSK type"=0} caption="QPSK System Parameters" {"PSK type" items=["normal", "shifted", "offset"]; "symbol map" format="%.3f"}
  in  "pi/4 DQPSK System Parameters 2":T5={"Samples per Symbol"=8, "symbol map"=[], "Differential PSK"=enum."enable", "PSK type"=1} caption="pi/4 DQPSK System Parameters" {"PSK type" items=["normal", "shifted", "offset"]; "symbol map" format="%.3f"}
  in  "OQPSK System Parameters 2":T5={"Samples per Symbol"=8, "symbol map"=[], "Differential PSK"=enum."disable", "PSK type"=2} caption="OQPSK System Parameters" {"PSK type" items=["normal", "shifted", "offset"]; "symbol map" format="%.3f"}
  in  "8-PSK System Parameters 2":T5={"Samples per Symbol"=8, "symbol map"=[], "Differential PSK"=enum."disable", "PSK type"=0} caption="8-PSK System Parameters" {"PSK type" items=["normal", "shifted", "offset"]; "symbol map" format="%.3f"}
  in  "16-PSK System Parameters 2":T5={"Samples per Symbol"=8, "symbol map"=[], "Differential PSK"=enum."disable", "PSK type"=0} caption="16-PSK System Parameters" {"PSK type" items=["normal", "shifted", "offset"]; "symbol map" format="%.3f"}
  in  "M 2":i32=4 caption="M" min=2 step=2
  in  "Custom System Parameters 2":T5={"Samples per Symbol"=8, "symbol map"=[], "Differential PSK"=enum."disable", "PSK type"=0} caption="Custom System Parameters" {"PSK type" items=["normal", "shifted", "offset"]; "symbol map" format="%.3f"}
  in  "Pulse Shaping Filter Parameters":T6={"Alpha"=0.5, "Filter Length"=6, "TX Filter"=enum."Root Raised Cos"} caption="Pulse Shaping Filter" {"Alpha" format="%.2f"}
  in  "Tx Parameters":T11={"Tx IQ Sampling\nRate [s/sec]"=500000.0, "Tx Frequency [Hz]"=2500000000.0, "Tx Gain [dB]"=0.0, "Tx Antenna"="TX1"} {"Tx Gain [dB]" format="%#.6p"; "Tx Frequency [Hz]" format="%#.6p"; "Tx IQ Sampling\nRate [s/sec]" format="%#.6p"}
  out "Actual Tx Parameters":T11={"Tx IQ Sampling\nRate [s/sec]"=200000.0, "Tx Frequency [Hz]"=2500000000.0, "Tx Gain [dB]"=0.0, "Tx Antenna"="TX1"} {"Tx Gain [dB]" format="%#.6p"; "Tx Frequency [Hz]" format="%#.6p"; "Tx IQ Sampling\nRate [s/sec]" format="%#.6p"}
  out "error out 2":errorcluster
  in  "Queue Length":i32=10
  in  "stop 3":bool caption="stop"
  out "Symbol Rate\n[symbols/sec] 5":dbl=25000.0 format="%#.6p"
  out "Constellation Graph 5":T8(graph) caption="Constellation Graph"
  in  "autoscale 3":bool caption="autoscale"
  in  "Tab Control 5":T9(tab)
  in  "Packet Parameters 5":T10={"Guard Bits "=30, "Sync Bits"=20, "Message Bits"=128}
  in  "Packet Pad \n[samples] 3":i32=200
  in  "Blank Frame \n[samples] 3":i32=500
  out "Number of Packets in Message 3":i32=46
  in  "PN sequence order\nfor Sync Bits 3":i32=31 caption="PN sequence order (9)"
  in  "Packet Repeat 3":i32=2
  in  "Select PSK Modulation Format 3":T4(tab)=enum."QPSK" caption="PSK"
  in  "BPSK System Parameters 5":T5={"Samples per Symbol"=8, "symbol map"=[], "Differential PSK"=enum."disable", "PSK type"=0} caption="BPSK System Parameters" {"PSK type" items=["normal", "shifted", "offset"]; "symbol map" format="%.3f"}
  in  "QPSK System Parameters 5":T5={"Samples per Symbol"=8, "symbol map"=[], "Differential PSK"=enum."disable", "PSK type"=0} caption="QPSK System Parameters" {"PSK type" items=["normal", "shifted", "offset"]; "symbol map" format="%.3f"}
  in  "pi/4 DQPSK System Parameters 5":T5={"Samples per Symbol"=8, "symbol map"=[], "Differential PSK"=enum."enable", "PSK type"=1} caption="pi/4 DQPSK System Parameters" {"PSK type" items=["normal", "shifted", "offset"]; "symbol map" format="%.3f"}
  in  "OQPSK System Parameters 5":T5={"Samples per Symbol"=8, "symbol map"=[], "Differential PSK"=enum."disable", "PSK type"=2} caption="OQPSK System Parameters" {"PSK type" items=["normal", "shifted", "offset"]; "symbol map" format="%.3f"}
  in  "8-PSK System Parameters 5":T5={"Samples per Symbol"=8, "symbol map"=[], "Differential PSK"=enum."disable", "PSK type"=0} caption="8-PSK System Parameters" {"PSK type" items=["normal", "shifted", "offset"]; "symbol map" format="%.3f"}
  in  "16-PSK System Parameters 5":T5={"Samples per Symbol"=8, "symbol map"=[], "Differential PSK"=enum."disable", "PSK type"=0} caption="16-PSK System Parameters" {"PSK type" items=["normal", "shifted", "offset"]; "symbol map" format="%.3f"}
  in  "M 5":i32=4 caption="M" min=2 step=2
  in  "Custom System Parameters 5":T5={"Samples per Symbol"=8, "symbol map"=[], "Differential PSK"=enum."disable", "PSK type"=0} caption="Custom System Parameters" {"PSK type" items=["normal", "shifted", "offset"]; "symbol map" format="%.3f"}
  in  "Pulse Shaping Filter Parameters 3":T6={"Alpha"=0.5, "Filter Length"=6, "TX Filter"=enum."Root Raised Cos"} caption="Pulse Shaping Filter" {"Alpha" format="%.2f"}
  in  "Tx Parameters 3":T11={"Tx IQ Sampling\nRate [s/sec]"=500000.0, "Tx Frequency [Hz]"=2500000000.0, "Tx Gain [dB]"=0.0, "Tx Antenna"="TX1"} {"Tx Gain [dB]" format="%#.6p"; "Tx Frequency [Hz]" format="%#.6p"; "Tx IQ Sampling\nRate [s/sec]" format="%#.6p"}
  out "Actual Tx Parameters 3":T11={"Tx IQ Sampling\nRate [s/sec]"=200000.0, "Tx Frequency [Hz]"=2500000000.0, "Tx Gain [dB]"=0.0, "Tx Antenna"="TX1"} {"Tx Gain [dB]" format="%#.6p"; "Tx Frequency [Hz]" format="%#.6p"; "Tx IQ Sampling\nRate [s/sec]" format="%#.6p"}
  out "error out 5":errorcluster
  in  "Queue Length 3":i32=10
  out "x .or. y? 6":bool
  in  "synchronization parameters 4":T1={"expected sync location (symbols)"=-1, "sync sequence"=[], "sync location uncertainty (symbols)"=0, "sync indent (symbols)"=0} caption="synchronization parameters" {"sync sequence" format="%.2f"}
  in  "Tab Control 7":T2(tab)=enum."Rx Display"
  in  "Acquisition Duration [sec] 4":dbl=0.04 format="%#.6p"
  in  "Rx Parameters 4":T3={"Rx IQ Sampling\nRate [s/sec]"=500000.0, "Rx\nFrequency [Hz]"=915000000.0, "Rx Gain [dB]"=20.0, "Rx Antenna"="RX1"} {"Rx Gain [dB]" format="%#.6p"; "Rx\nFrequency [Hz]" format="%#.6p"; "Rx IQ Sampling\nRate [s/sec]" format="%#.6p"}
  out "Actual Rx Parameters  4":T3={"Rx IQ Sampling\nRate [s/sec]"=500000.0, "Rx\nFrequency [Hz]"=915000000.0, "Rx Gain [dB]"=20.0, "Rx Antenna"="RX1"} {"Rx Gain [dB]" format="%#.6p"; "Rx\nFrequency [Hz]" format="%#.6p"; "Rx IQ Sampling\nRate [s/sec]" format="%#.6p"}
  out "Symbol Rate\n[symbols/sec] 7":dbl=62500.0 format="%#.6p"
  in  "Choose a PSK Format 4":T4(tab)=enum."QPSK" caption="PSK"
  in  "BPSK System Parameters 7":T5={"Samples per Symbol"=8, "symbol map"=[], "Differential PSK"=enum."disable", "PSK type"=0} caption="BPSK System Parameters" {"PSK type" items=["normal", "shifted", "offset"]; "symbol map" format="%.3f"}
  in  "QPSK System Parameters 7":T5={"Samples per Symbol"=8, "symbol map"=[], "Differential PSK"=enum."disable", "PSK type"=0} caption="QPSK System Parameters" {"PSK type" items=["normal", "shifted", "offset"]; "symbol map" format="%.3f"}
  in  "pi/4 DQPSK System Parameters 7":T5={"Samples per Symbol"=8, "symbol map"=[], "Differential PSK"=enum."enable", "PSK type"=1} caption="pi/4 DQPSK System Parameters" {"PSK type" items=["normal", "shifted", "offset"]; "symbol map" format="%.3f"}
  in  "OQPSK System Parameters 7":T5={"Samples per Symbol"=8, "symbol map"=[], "Differential PSK"=enum."disable", "PSK type"=2} caption="OQPSK System Parameters" {"PSK type" items=["normal", "shifted", "offset"]; "symbol map" format="%.3f"}
  in  "8-PSK System Parameters 7":T5={"Samples per Symbol"=8, "symbol map"=[], "Differential PSK"=enum."disable", "PSK type"=0} caption="8-PSK System Parameters" {"PSK type" items=["normal", "shifted", "offset"]; "symbol map" format="%.3f"}
  in  "16-PSK System Parameters 7":T5={"Samples per Symbol"=8, "symbol map"=[], "Differential PSK"=enum."disable", "PSK type"=0} caption="16-PSK System Parameters" {"PSK type" items=["normal", "shifted", "offset"]; "symbol map" format="%.3f"}
  in  "M 7":i32=4 caption="M" min=2 step=2
  in  "Custom System Parameters 7":T5={"Samples per Symbol"=8, "symbol map"=[], "Differential PSK"=enum."disable", "PSK type"=0} caption="Custom System Parameters" {"PSK type" items=["normal", "shifted", "offset"]; "symbol map" format="%.3f"}
  in  "filter parameters 4":T6={"Alpha"=0.5, "Filter Length"=6, "TX Filter"=enum."Root Raised Cos"} caption="Matching Filter Parameters" {"Alpha" format="%.2f"}
  in  "PN Sequence Order\nfor Sync 4":i32=31
  in  "Packet Parameters 7":T7={"Guard Bits "=30, "Sync Bits"=20, "Message Bits"=128, "Number of Packets \nto Expect"=46}
  out "Recovered Message 4":string="Two roads diverged in a yellow wood,\nAnd sorry I could not travel both\nAnd be one traveler, long I stood\nAnd looked down one as far as I could\nTo where it bent in the undergrowth.\n\nThen took the other, as just as fair,\nAnd having perhaps the better claim,\nBecause it was grassy and wanted wear;\nThough as for that the passing there\nHad worn them really about the same.\n\nAnd both that morning equally lay\nIn leaves no step had trodden black.\nOh, I kept the first for another day!\nYet knowing how way leads on to way,\nI doubted if I should ever come back.\n\nI shall be telling this with a sigh\nSomewhere..."
  out "Received Signal (Raw) 4":dbl[](graph)
  out "Constellation Graph 7":T8(graph)=[{"Decimated Array"=[-0.6804993103727607, -0.6771092058245918, -0.6428257187708691, 0.7259219405542873, 0.7311366832454209, -0.6450362325295403, -0.658892442379921, -0.6855840493085356, -0.646998431742077, -0.6568678904388265, 0.7432214399633668, -0.6618522924674632, -0.6753922285302938, 0.6950905811428861, 0.7248141384495557, 0.7218255862492685, 0.704818637196686, 0.7027336696732543, 0.7016253671990413, 0.7082534735709545, 0.7084209330001522, 0.7036372125301554, 0.7010930640613204, 0.7075984577478206, 0.7100058187983528, 0.7171431626733421, 0.7279231861183771, 0.6959557947635676, -0.7024336186443912, -0.7110189818905128, 0.6934234462727887, 0.7327126116070742, 0.7051667045224878, 0.690798979580973, -0.6877839781333666, 0.6889445287579181, 0.716354235720989, -0.706071092371314, 0.72195318833854, -0.7119212984185137, 0.7223509528651848, -0.7244956435522718, -0.6716656585292338, -0.7182056308592257, 0.724421589775866, -0.6763390206227603, 0.7587597202334532, -0.6966306246608392, -0.6999692828092537, -0.7056805503027465, 0.7430994824068496, 0.7108305621069824, 0.7197425435843314, -0.7051937005816177, -0.6734048186040171, -0.6909214820858487, 0.7004218263991402, -0.6889802592692622, 0.7244882842042791, 0.7027757047403482, -0.7012448562483489, -0.6963431828766949, 0.7166197717755273, 0.7431431506248717, 0.7233235134334371, 0.6983161172439467, 0.7059749857271942, -0.6872358926309042, 0.6918268533027474, -0.7138701729016586, -0.6801285945135653, 0.7195044185357663, 0.6810587309328351, -0.6856313040037053, -0.7011043347997452, 0.6920652628903768, -0.7080955978852922, -0.6860253207439192, -0.7101309321759165, 0.7212965033681705, 0.6967245108747491, 0.7128097205123256, 0.6657328144726218, 0.6985573048815797, 0.6967609587320983, 0.720489591403177, -0.6992149062771553, 0.6810319795543738, -0.7124274384065621, -0.6689704942642202, 0.7017697482270308, 0.7036983705130238, -0.69378287602043, -0.6926507402482928, 0.6832891050414109, 0.7219614630178657, 0.7044242088089868, 0.6722056874933439, -0.6818156450864503, 0.6786113633855301, 0.7039257931121476, -0.6836867328922335, 0.6967676536286352, -0.7018627722542645, 0.7033449800412358, -0.7121625353086042], "Decimated Array"=[0.7327573786203745, 0.7417811878517194, -0.6799031648608087, -0.7111421642681004, -0.727382953469249, -0.6704579022356528, -0.6770604606987946, 0.7538529097411865, -0.6722715103438465, -0.6756211416707443, -0.6914774106844375, -0.673529581873597, 0.7393627898718214, 0.7522557788351737, 0.7435736461024193, 0.7257726558576425, 0.7275033865931528, 0.7311828384458046, 0.7293390182016347, 0.7220976758138733, 0.7195981106474233, 0.7211811690986409, 0.7188051788075457, 0.7320183145085448, 0.6962181897094762, 0.7305998791526044, -0.6967382767827438, 0.7159339540668409, -0.7008762468325049, 0.7525668303202456, 0.7058888207208955, 0.7252589385855543, -0.7159704258460882, 0.7370284868429373, 0.7140037167311404, 0.7389767670280546, -0.6960013467696725, 0.7235856630223708, -0.6972846806923089, -0.657884155216942, -0.6949224336608516, 0.7453870445521058, -0.6844918028247094, -0.6835224068604273, -0.7079388773369498, 0.7505384293302241, 0.6958348088594112, 0.7516973279064126, -0.6781015202421304, 0.7276930986154884, 0.7072095654921254, -0.6818066642899347, -0.702124108056222, 0.7365289833752492, 0.7313371097907961, 0.7586596196292686, -0.7079902911617727, 0.713630396728027, -0.7007240447824197, 0.7246614220304907, -0.7064584618733396, 0.7515472341269214, 0.6939391865838809, 0.7190183727683939, -0.6934598211856411, 0.7287398470888085, 0.7237013633767214, 0.7256529739097736, -0.6909901985488635, 0.7147604584382636, 0.6881560723752628, 0.7236976539802175, -0.6922424302133595, 0.7045483839307563, 0.6890103411064745, -0.6887965775506286, -0.7136342940914308, 0.7205719868506776, 0.7023916754066073, 0.7473081616445082, -0.6863264429683489, 0.7186091906642366, -0.7100679145508004, -0.6810878313976068, 0.7293932651728482, 0.722408788035578, 0.7004331018480651, -0.6822150791593455, 0.685337537979504, 0.7132682495621445, -0.6721281174161831, 0.7245443113283739, -0.7431160183824671, 0.7359349670621476, 0.7174344380700259, 0.7431105593701001, -0.6993804544754962, 0.7453566040596344, 0.6929469282521439, 0.7449696798222867, -0.693664788209523, 0.7157173189250563, -0.7183409139718169, -0.6991338441055578, -0.7093747657586275, 0.724868684652829]}, {"Decimated Array"=[-0.6804993103727607, -0.6762349965387238, -0.6685108157798112, -0.6587623289821404, -0.6494739544100483, -0.6438465750011458, -0.645155862498135, -0.6559333949667008, -0.6771092058245918, -0.707329395010057, -0.7427108893571827, -0.7768816274525345, -0.8016064503455926, -0.8078913118575249, -0.7873020181422804, -0.7333876332701184, -0.6428257187708691, -0.5161117575568228, -0.35777203758853365, -0.17570329650700167, 0.01987541369217473, 0.21778298257008183, 0.4072432109758152, 0.5789865397268567, 0.7259219405542873, 0.8433225109633283, 0.9285347773827741, 0.9803625623365572, 0.9983411710644498, 0.9823024312079763, 0.9321501534368272, 0.8480801425231922, 0.7311366832454209, 0.5839247754585907, 0.41126876723240074, 0.2204206478178329, 0.020932943403138903, -0.1761332529377578, -0.3593512576776315, -0.5183227318987554, -0.6450362325295403, -0.7348944300155227, -0.7873580245691122, -0.8057437870339258, -0.7965717988687436, -0.7684407927742708, -0.7306238606226202, -0.6917860656058442, -0.658892442379921, -0.6364690666334113, -0.6263656338128196, -0.6279033391241801, -0.6383295002999582, -0.6535857140497858, -0.6691389263327601, -0.6808303682804338, -0.6855840493085356, -0.6819546232796994, -0.6704727894453094, -0.6535744314745204, -0.6353365462635079, -0.6208696353048802, -0.6154307523642993, -0.6233724286798671, -0.646998431742077, -0.6855864576394015, -0.7347128803667217, -0.7860882541221362, -0.8282453730286534, -0.8479309126781169, -0.8321007406466316, -0.7702787309009056, -0.6568678904388265, -0.4928870454737699, -0.286812316855307, -0.054181947000257816, 0.18398541460571163, 0.403912791430555, 0.5822957160369652, 0.6996654194867074, 0.7432214399633668, 0.7085518372290116, 0.6001271112229511, 0.43028071322686884, 0.21712133759522834, -0.01828477060583316, -0.25486167705907176, -0.474106655260725, -0.6618522924674632, -0.8090041994597156, -0.9113555181844136, -0.9685514235160106, -0.9827395175415803, -0.9572113882143858, -0.8953875269303032, -0.8004356628744611, -0.6753922285302938, -0.5237515103490776, -0.3502005293644506, -0.1611351791820148, 0.03517140208780353, 0.22893110044459927, 0.40972263321669966, 0.5677345648283395, 0.6950905811428861, 0.7869683371034619, 0.8423038906676682, 0.8638849324516561, 0.8577538092414735, 0.8321468933549871, 0.7961070317612736, 0.7580880124868856, 0.7248141384495557, 0.7005277134039959, 0.686923334338586, 0.6833877232132058, 0.6876280888811944, 0.6964899036822818, 0.706747954834772, 0.7157647696850384, 0.7218255862492685, 0.724268969267967, 0.7234261321898535, 0.7202619630220548, 0.7159731242866095, 0.7116890979547664, 0.7082240869885714, 0.70594341514383, 0.704818637196686, 0.7045271958113069, 0.7047088927454438, 0.7050023859293303, 0.7051255773761397, 0.7049541452505861, 0.7044514570052206, 0.7036747950662702, 0.7027336696732543, 0.7017628701423971, 0.7009138948889888, 0.7003118882562483, 0.7000261021126073, 0.7000875017890581, 0.7004449481097869, 0.7009932809698078, 0.7016253671990413, 0.702221540251104, 0.7027618684813808, 0.7032916906181711, 0.7038854962099375, 0.7046487256800136, 0.7056308879137863, 0.7068515417419651, 0.7082534735709545, 0.7096888191782372, 0.7109913402244956, 0.7119894724643936, 0.7124890080936077, 0.7123827414517839, 0.7116323891766451, 0.7102633952930952, 0.7084209330001522, 0.7063057748688335, 0.7042562032788021, 0.7025954190884202, 0.7015546954049546, 0.7012557549487087, 0.7016448259380934, 0.7025398218482226, 0.7036372125301554, 0.7046321819639692, 0.7053295412842902, 0.7055972799037947, 0.705357986716468, 0.7046523984817116, 0.7036068751653552, 0.7023536981462808, 0.7010930640613204, 0.7000326295845363, 0.6993965049981011, 0.6993226127993213, 0.6998881120919372, 0.701113074412268, 0.7029138523453567, 0.7051416575412044, 0.7075984577478206, 0.710078980444559, 0.7123321038850414, 0.7140736603763724, 0.7150314533562983, 0.7150214932752349, 0.7140093308210059, 0.7121877418723002, 0.7100058187983528, 0.70805206355385, 0.7070027727419878, 0.7073212689161522, 0.7091056294101988, 0.7119833987327618, 0.7150644848824459, 0.7171668570713718, 0.7171431626733421, 0.71423133689185, 0.7085192919358748, 0.7011650150275229, 0.6943243914091253, 0.6909299894216554, 0.694045612210552, 0.706066960259486, 0.7279231861183771, 0.7583890909767882, 0.7938021658029275, 0.8279962238841705, 0.8528896550258644, 0.8595701988778817, 0.8395633321459017, 0.7862278633870129, 0.6959557947635676, 0.5689496495122442, 0.4094105630569515, 0.22502717825358973, 0.025894312218078558, -0.17672464042078925, -0.37176542586543576, -0.5495413422869474, -0.7024336186443912, -0.8251771287794907, -0.9146738107129905, -0.9693864660264264, -0.9886486884020281, -0.9721997012143947, -0.920010882437784, -0.8324905468768208, -0.7110189818905128, -0.5586215402038113, -0.38057133580870495, -0.18461757845785642, 0.019294891934465676, 0.2197963582992338, 0.4053691867674974, 0.5657713716359056, 0.6934234462727887, 0.7843501298361789, 0.8386729718179944, 0.8602628823550353, 0.855774513907276, 0.8333154686311419, 0.8010170366525857, 0.7658225991667146, 0.7327126116070742, 0.7045406905991981, 0.6824916000019303, 0.6667964864918056, 0.6575588911889615, 0.6553991485314229, 0.6616300661715835, 0.677865934701111, 0.7051667045224878, 0.7429233296416752, 0.7878677137961015, 0.8333853282559609, 0.8696348770191419, 0.8846190114381185, 0.8659756375138661, 0.8033400824826783, 0.690798979580973, 0.5288571353054295, 0.32551133007737276, 0.09595098720473762, -0.13906888290440567, -0.35588344294942403, -0.5312979803398246, -0.646084108275294, -0.6877839781333666, -0.6524636145322816, -0.5450893812430798, -0.37828756856953233, -0.17009276356333847, 0.0590247558982818, 0.28912715162217667, 0.5032762839933951, 0.6889445287579181, 0.8383428746399739, 0.9477025130341128, 1.015790170453614, 1.0423483901645878, 1.0268512388275022, 0.9680879161655901, 0.8646551393981081, 0.716354235720989, 0.5260764152807655, 0.30160439840294034, 0.05668512406955431, -0.18910351581760784, -0.4118751751084471, -0.5863423085037114, -0.6897554505434935, -0.706071092371314, -0.6295185621493208, -0.4668637151478481, -0.23765972556227086, 0.027714817455610417, 0.29202447870753795, 0.5167154122972588, 0.6679084709283569, 0.72195318833854, 0.6695114009171929, 0.5175155629675429, 0.2883041299697019, 0.01623720013151288, -0.25755900242514196, -0.4917082138253101, -0.6510176327160702, -0.7119212984185137, -0.6659995880876536, -0.5209852917537516, -0.2992839322286186, -0.03416997277404838, 0.2355466281568285, 0.4714352113659737, 0.6410442893752866, 0.7223509528651848, 0.7062991907811851, 0.5973003486423586, 0.4116890808688979, 0.17445466790696096, -0.08489625696410336, -0.3368901331962952, -0.5561324114364461, -0.7244956435522718, -0.832904063982776, -0.8817003370505312, -0.8795283892255058, -0.841156501109088, -0.7846263716950196, -0.7281214416972949, -0.6870445779683771, -0.6716656585292338, -0.6855631019709484, -0.7251869491105687, -0.7803544807713914, -0.8357414937022205, -0.8732615963603204, -0.8749681769421048, -0.8261602248386887, -0.7182056308592257, -0.5506938062457699, -0.3325933377055765, -0.08189760414583691, 0.17618237159000388, 0.4123697444728759, 0.5974694739328056, 0.7068084628379865, 0.724421589775866, 0.6461724854013321, 0.4812775786848407, 0.25159361606242997, -0.011058078343011023, -0.2692923486046545, -0.48569025029571594, -0.6284581525739953, -0.6763390206227603, -0.6219818356022658, -0.47306441806801147, -0.2510857990405568, 0.01202477775150253, 0.27875734553572085, 0.5116930035471384, 0.6789865139576629, 0.7587597202334532, 0.7418192787585248, 0.6323458533022597, 0.446406792743502, 0.20878035238051276, -0.05119783320575381, -0.3042611875270661, -0.5253152667965498, -0.6966306246608392, -0.8095606744479041, -0.8647740627418172, -0.870930075780708, -0.8423384959975685, -0.7960318277718325, -0.7486596019303445, -0.7137982795070836, -0.6999692828092537, -0.7095971091381883, -0.7390816485119921, -0.7796138336185289, -0.818762813999536, -0.8425904879324037, -0.8378822227707572, -0.7942341058424417, -0.7056805503027465, -0.571726769560303, -0.39765177441111643, -0.19391837432237818, 0.025178720377377686, 0.24333379676657457, 0.44433965307888695, 0.6142375047967751, 0.7430994824068496, 0.8263038750024307, 0.8650100488333368, 0.8657148042767202, 0.8390794723757462, 0.7981161813167071, 0.7560954579232749, 0.7244176046468488, 0.7108305621069824, 0.718204650734365, 0.7441150394580835, 0.7812106743682087, 0.8183931962770272, 0.8425254654823089, 0.8406177118076219, 0.8019301699596733, 0.7197425435843314, 0.5926686710089698, 0.4251140503775492, 0.22683136067452989, 0.011660330280988253, -0.20423795622266205, -0.4045792942890271, -0.57504838691632, -0.7051937005816177, -0.7897661684393493, -0.8293068652572223, -0.8299006515155186, -0.8021229049955473, -0.7594233513128958, -0.715953221878639, -0.684307426439313, -0.6734048186040171, -0.6868570522140265, -0.7221874426788824, -0.7708237442647581, -0.8191585903691571, -0.8505818015508355, -0.8481661462885941, -0.7977634650762118, -0.6909214820858487, -0.5271825682100394, -0.31525436879598623, -0.07267661804829456, 0.17610311762416703, 0.4028796348907104, 0.5798206568779839, 0.6838352068807156, 0.7004218263991402, 0.6263585027788804, 0.4707037347107586, 0.2537801245269521, 0.004363575376446024, -0.244425088845282, -0.45988451941533137, -0.6143614233710846, -0.6889802592692622, -0.675810131006379, -0.5782280367437729, -0.40962067096108434, -0.19054676255841746, 0.05481291967260732, 0.3023001215109928, 0.5308329677888366, 0.7244882842042791, 0.8734246012838044, 0.9735701497284382, 1.0253939516322779, 1.0322709072595566, 0.9989018615889086, 0.9300855209250758, 0.8301278260930205, 0.7027757047403482, 0.5516545283139476, 0.38091449347590134, 0.19570631362414656, 0.002354352790910658, -0.19179798997086855, -0.3788570549590451, -0.5510272450358933, -0.7012448562483489, -0.8236915392774603, -0.914039706142418, -0.9694184170252935, -0.9881756409826234, -0.9696303075716558, -0.913918517626886, -0.8220829857364051, -0.6963431828766949, -0.5405016807251724, -0.36031892603430715, -0.16359224329210514, 0.04013418091790215, 0.24018456190270834, 0.425760423266114, 0.5870829268985424, 0.7166197717755273, 0.8099833426954562, 0.8664917523906949, 0.8890606065456064, 0.8835329376488369, 0.8577948250420299, 0.8205354221662687, 0.7800304020582047, 0.7431431506248717, 0.7146443568705966, 0.6969512334183051, 0.6901074157262647, 0.6922880175560046, 0.7003398356906728, 0.7105226229352982, 0.7191652725013788, 0.7233235134334371, 0.7213381284523223, 0.7131072858574705, 0.7002046822080928, 0.6857438943908143, 0.6739876200747604, 0.6696394639541572, 0.6768836675096863, 0.6983161172439467, 0.7338690127516884, 0.7800774899548244, 0.829602819630056, 0.8715371312486556, 0.892620000492053, 0.8790856399483223, 0.8192212166031462, 0.7059749857271942, 0.5391749210900726, 0.3269503040314498, 0.08573815461541592, -0.1612255824786287, -0.386730293143399, -0.5635326559438285, -0.6686383256247854, -0.6872358926309042, -0.6156114857935734, -0.4623211423735695, -0.24733010394610414, 0.0007198102460047476, 0.24863863484628498, 0.4635514254715547, 0.6176104623364325, 0.6918268533027474, 0.6782756201030052, 0.5805134425392992, 0.41210610757403726, 0.19372452237290802, -0.050391409713054024, -0.29611210645789393, -0.5225111093000552, -0.7138701729016586, -0.8605441211993027, -0.9585448112667802, -1.008414026021156, -1.0135648241052666, -0.978745896542667, -0.9087849082692102, -0.8079881948321259, -0.6801285945135653, -0.5287862221062773, -0.35805233939202374, -0.1729861888667504, 0.020116186161511587, 0.21387335563181437, 0.40025748153323093, 0.5712472743319003, 0.7195044185357663, 0.8388895884119506, 0.9249072134737321, 0.9746853929178996, 0.9868923875604191, 0.9616684243967665, 0.9003848901697228, 0.8056175444681817, 0.6810587309328351, 0.5314881726723011, 0.3626554692436761, 0.18103860407685468, -0.006510589607727805, -0.1931114704827839, -0.3722848897831801, -0.5381718770034626, -0.6856313040037053, -0.8101801487665511, -0.9076732803716326, -0.9739618526107378, -1.004716020345832, -0.9956414793795033, -0.9430154749490675, -0.8446500281072215, -0.7011043347997452, -0.516842399364099, -0.3010204717594881, -0.06763754580789842, 0.16514820448340978, 0.37668157665933155, 0.5461920463765456, 0.655552915260347, 0.6920652628903768, 0.6505655304034257, 0.5346883243834851, 0.35661897243093144, 0.13559774776324776, -0.1046718797566402, -0.3394032573081613, -0.5461789593962133, -0.7080955978852922, -0.8157954529602021, -0.8683801331865292, -0.8727983131028657, -0.8421078226859732, -0.7927582081222804, -0.741572331068595, -0.7028423018527019, -0.6860253207439192, -0.6943551977069015, -0.7245345157854167, -0.7675646042411391, -0.8104296201087327, -0.8383601072014226, -0.8373952185694984, -0.7966528302359737, -0.7101309321759165, -0.5776984378988999, -0.40521323182553737, -0.2036592543667804, 0.012419924984258368, 0.22695341747885692, 0.42449093142276867, 0.592188438033417, 0.7212965033681705, 0.8079364234726191, 0.8532668165288172, 0.8627953034872611, 0.8451288060001957, 0.8104079963441455, 0.7687359339278867, 0.7287670505538517, 0.6967245108747491, 0.6759780606536095, 0.667107406232625, 0.6684364317450245, 0.676784919616326, 0.6884291860003884, 0.699890853611944, 0.7085144901744879, 0.7128097205123256, 0.7124229876828518, 0.7080187790236897, 0.7008050101089057, 0.6921805709227881, 0.6834646736814466, 0.6757033963031507, 0.669648508318143, 0.6657328144726218, 0.6642652636337992, 0.6653767657521718, 0.6690028595853793, 0.674775333959487, 0.6819477949985021, 0.6893278789128267, 0.6953927726157616, 0.6985573048815797, 0.697578095425808, 0.6920506573747554, 0.6828307951888688, 0.6722732265164824, 0.6640958466160822, 0.6627912256868634, 0.6726965874495441, 0.6967609587320983, 0.735252994349721, 0.7847852487718341, 0.837860611588047, 0.8832021671865116, 0.9070282265831913, 0.8950883370622812, 0.8352994933427401, 0.720489591403177, 0.5506306635171825, 0.3342725070105252, 0.08840692523651153, -0.16315427404215097, -0.3926718560799536, -0.572539734272038, -0.6796338477180948, -0.6992149062771553, -0.6277630208203462, -0.4741131473050659, -0.2585293695095081, -0.009930257048617025, 0.23830892263310452, 0.45325402085890604, 0.607121618765611, 0.6810319795543738, 0.6672310461853316, 0.5694827757707117, 0.4015147931896041, 0.1841817171712272, -0.05817646638242799, -0.3014136753019013, -0.524665532969832, -0.7124274384065621, -0.855285246094759, -0.9495933688767533, -0.996236130847489, -0.9989838487955423, -0.9628841324499167, -0.8930056180780918, -0.7937877561121499, -0.6689704942642202, -0.5220072798874036, -0.3566099133872175, -0.17731129436958973, 0.010268861422383327, 0.19945198638565087, 0.3827826926443024, 0.5526251582270405, 0.7017697482270308, 0.8239876507426606, 0.9144785689512498, 0.9699591512942685, 0.9886252045487814, 0.9700306803372667, 0.9149020439452162, 0.825116863065968, 0.7036983705130238, 0.554839481392563, 0.3840291620621759, 0.19787647745423148, 0.003860727052948984, -0.18999525295737457, -0.3757044734833313, -0.5458056810042837, -0.69378287602043, -0.814366828718361, -0.9036469275456485, -0.9588849469775574, -0.9783006504455267, -0.960973889608092, -0.9067746467203663, -0.8165903751017708, -0.6926507402482928, -0.5388812935652539, -0.361228905014989, -0.16771060388912773, 0.031903370124330505, 0.22678679843602859, 0.4061707941853134, 0.5606402717569381, 0.6832891050414109, 0.7705901219032752, 0.8228006526178891, 0.8436430103344122, 0.8394755303225311, 0.8180394512925253, 0.7871333265278456, 0.7534665911565442, 0.7219614630178657, 0.695510686451852, 0.6753252498343544, 0.6615878037807406, 0.6542998195364643, 0.6538606147644473, 0.6612723675386262, 0.6778625191525914, 0.7044242088089868, 0.7402649399766673, 0.7822594926239343, 0.8241634231439008, 0.8566831085547093, 0.8684082810681567, 0.8475040183712003, 0.784012885063017, 0.6722056874933439, 0.5125005393952523, 0.31260026449095785, 0.08722135068631567, -0.14339658857823498, -0.35611765704885123, -0.5282733760242059, -0.6409441045045646, -0.6818156450864503, -0.6469272017629891, -0.5410574986904879, -0.37652152921039295, -0.17097947697100876, 0.05541171165914345, 0.2829619347828144, 0.49484727767121917, 0.6786113633855301, 0.8264573551553331, 0.9345361200971587, 1.0015661687984379, 1.0272888190262575, 1.0112965146842847, 0.952583288738177, 0.8500890658990591, 0.7039257931121476, 0.5171900515296706, 0.29764273007471115, 0.05870661463653025, -0.1806017914741214, -0.39721826601913907, -0.5668036345777544, -0.6674573482841338, -0.6836867328922335, -0.6099467963750959, -0.4528161959244535, -0.23123780147788525, 0.0254037230819288, 0.2810884215045038, 0.4984727203603391, 0.6447055580185417, 0.6967676536286352, 0.6455398584402634, 0.4976568874522828, 0.2746594289249686, 0.009825427460916032, -0.25698435822392646, -0.4855514161032739, -0.6415528231225354, -0.7018627722542645, -0.6580125604775775, -0.517265265222927, -0.30121265695938104, -0.04212438479079229, 0.22217065809727116, 0.45405673442103006, 0.6217149465148919, 0.7033449800412358, 0.6897787566619501, 0.5850104229528822, 0.4047415306155254, 0.17323834921239678, -0.08075812096424864, -0.3284327261412435, -0.5448733152596168, -0.7121625353086042, -0.8211818337976253, -0.8719691969355644, -0.8727186157199347, -0.8376486334880819, -0.7842590106698991, -0.7303274268398209, -0.6909814362358659], "Decimated Array"=[0.7327573786203745, 0.8571160437398065, 0.9481227692632541, 1.003980881033979, 1.0238155370523472, 1.0072368286759465, 0.9541994905916551, 0.8651912730450063, 0.7417811878517194, 0.5871636451740783, 0.40676677760888635, 0.20846130324205578, 0.0022318875001048045, -0.2005410967663612, -0.38829860023304064, -0.5506845398656813, -0.6799031648608087, -0.7716987861234258, -0.8258475294329478, -0.8459996756657396, -0.8388616433189412, -0.8130753155007096, -0.7778435482452709, -0.7416372990136377, -0.7111421642681004, -0.6905831950739342, -0.6815454430666558, -0.6831516021872707, -0.6925669267273694, -0.7057731727702966, -0.7184007879882285, -0.7265282476091678, -0.727382953469249, -0.7198001905615271, -0.7045629848520147, -0.6843705475932246, -0.6634185556136458, -0.646887119577886, -0.6400361359583534, -0.6471594714631548, -0.6704579022356528, -0.7090564063186768, -0.7584053880552923, -0.8101244036157627, -0.8526189235085075, -0.872417498261418, -0.8561767863823757, -0.7930533916017833, -0.6770604606987946, -0.5089375701527854, -0.2971550620890392, -0.05761269204799846, 0.18789151496970918, 0.4143336303799478, 0.596919125262307, 0.7147087986695557, 0.7538529097411865, 0.7097353627437273, 0.5877778836770051, 0.40257278286196346, 0.1755748921605498, -0.06817834720063913, -0.30381917292160493, -0.5101473732591594, -0.6722715103438465, -0.782942771822579, -0.8426075541528982, -0.8581499860345086, -0.8406550377330191, -0.8028915815603971, -0.7569445207502417, -0.7124441110679234, -0.6756211416707443, -0.6492985792878058, -0.6336104831921037, -0.6270868628284776, -0.6278993868440812, -0.6347460148648578, -0.6473189374357599, -0.6660652122000107, -0.6914774106844375, -0.7231297220029862, -0.7587664029448702, -0.7936544758660282, -0.8205522923344901, -0.8305429506490288, -0.8142884856193261, -0.7636823212203829, -0.673529581873597, -0.5429181777841331, -0.3758793938755062, -0.18113858110834186, 0.028812354472331908, 0.23939310934756888, 0.4359274511900307, 0.6056519046787863, 0.7393627898718214, 0.8324327306148087, 0.8851319247653551, 0.9020886016493107, 0.8911142062914292, 0.8617307665544903, 0.8235701121823792, 0.7850172209229723, 0.7522557788351737, 0.7288635601528786, 0.7158958847588804, 0.7123277223581522, 0.715761845721655, 0.7231900323302534, 0.7316880970831603, 0.7389528359720056, 0.7435736461024193, 0.7451046063677472, 0.743901281226759, 0.740788821822152, 0.7367782401995692, 0.7328033193551644, 0.7294981194191762, 0.7271513904156902, 0.7257726558576425, 0.725159941446078, 0.725060989178965, 0.7252632377419967, 0.7256163395829798, 0.7260606904500417, 0.7265379023034586, 0.7270291732601397, 0.7275033865931528, 0.7279199682707127, 0.7282769079854728, 0.7285974590770533, 0.7289407767207793, 0.7293428506461535, 0.7298479408102396, 0.7304778513692572, 0.7311828384458046, 0.7318265401385785, 0.7323028750384627, 0.7325567749966301, 0.7325033028493253, 0.7321158823152807, 0.7314068004824351, 0.7304533892028899, 0.7293390182016347, 0.7281572743585262, 0.7270606197087242, 0.7261241067000211, 0.7253508195631971, 0.7246697616263047, 0.723969429286671, 0.723139564739256, 0.7220976758138733, 0.7208555865072881, 0.719568292828321, 0.7184478733558384, 0.7176993275862744, 0.7174622207349447, 0.7177521937986072, 0.718516228428159, 0.7195981106474233, 0.7207879819353863, 0.7218924194293399, 0.7227111613943498, 0.7231168859595661, 0.7230786498664554, 0.7226411424851807, 0.7219463720454906, 0.7211811690986409, 0.7204810710907097, 0.7199538718599565, 0.7196320372423504, 0.7194607411817737, 0.7193099127963588, 0.7190971249818399, 0.7188635612803779, 0.7188051788075457, 0.7192369464355841, 0.7205351477714964, 0.7229401499987833, 0.7263486481418566, 0.7301617369824043, 0.7333271712095472, 0.7344308070476105, 0.7320183145085448, 0.7250816880667706, 0.7135657369657201, 0.6987104127947069, 0.6831567860992641, 0.6708043964638186, 0.6662258399732381, 0.6737496016563864, 0.6962181897094762, 0.7338123953236427, 0.7831464621140352, 0.8367458472751513, 0.8833813981307604, 0.9091987678800104, 0.8998091259693833, 0.8428401153753142, 0.7305998791526044, 0.562507495226734, 0.34659814194077, 0.0995702257773744, -0.15462281131582128, -0.3875977492359962, -0.5706271624637833, -0.6790839949047796, -0.6967382767827438, -0.6189803271815245, -0.4544562375583789, -0.22459908414379984, 0.03903553601854455, 0.29916696405087967, 0.5182679460830586, 0.6643639077354586, 0.7159339540668409, 0.6652943920234429, 0.5198749673865217, 0.300993470244488, 0.04051717061424443, -0.22409581460784916, -0.45544556602126973, -0.6216785191074483, -0.7008762468325049, -0.6837610820977862, -0.5742886326760264, -0.3883111156265534, -0.1505286326662823, 0.10967239939698414, 0.3627475020866999, 0.5831487815378037, 0.7525668303202456, 0.8617987081334637, 0.9111768991603971, 0.9094611758407977, 0.8715862070139058, 0.8157455416667302, 0.760202018310825, 0.7202658930923688, 0.7058888207208955, 0.7201847936946834, 0.759052366114439, 0.811812333812609, 0.8630070563777121, 0.8948697888398245, 0.8903643946442023, 0.8361831300618912, 0.7252589385855543, 0.5584821670091451, 0.345315670477598, 0.10299763765352206, -0.14547539122840722, -0.37428698339337824, -0.5583637418127292, -0.6768312337753024, -0.7159704258460882, -0.6711625159308375, -0.5476542552431498, -0.3597709705436185, -0.1287724532856077, 0.12018518168690656, 0.36151984386717273, 0.572699142103299, 0.7370284868429373, 0.8455964386542135, 0.8979126579643226, 0.9012807607635166, 0.8690744380604796, 0.8181990426007191, 0.7661088030574076, 0.7279245613823432, 0.7140037167311404, 0.7282038712248695, 0.7671972819282604, 0.8208631561250372, 0.8738564756136162, 0.9080475656744531, 0.9055112204914009, 0.8518434216042863, 0.7389767670280546, 0.5673122043840576, 0.346672036977057, 0.09563946895916749, -0.1604955961723308, -0.3929887785452873, -0.573731438794397, -0.6795623772004052, -0.6960013467696725, -0.619916032405668, -0.46047605211853976, -0.238293779549608, 0.017302276506560462, 0.2723050965454336, 0.4928472153853533, 0.6499682346772773, 0.7235856630223708, 0.7050531042870595, 0.5980296925245243, 0.4173625434472803, 0.18635581949974522, -0.06697296685650257, -0.3141616680583659, -0.5303108718258116, -0.6972846806923089, -0.805693295562243, -0.8554610680619644, -0.8548810350527455, -0.8184903429533198, -0.7641725094683359, -0.7100008771843999, -0.671228658984871, -0.657884155216942, -0.6731679025330721, -0.7131015741595147, -0.7671687462263975, -0.8200654189127506, -0.8542004537564716, -0.8526249939936517, -0.8019646550151107, -0.6949224336608516, -0.5320250473508275, -0.32225185034324333, -0.08237582607009868, 0.1650026835738332, 0.39428466394542017, 0.5803342409591474, 0.7020686940954762, 0.7453870445521058, 0.7052505477960299, 0.5864589514160631, 0.40293010537214813, 0.17562748086081167, -0.0704552502607787, -0.309822690701368, -0.5200321703524325, -0.6844918028247094, -0.7944039739927944, -0.849369247148433, -0.856656043797114, -0.8292787623167311, -0.7833804658452638, -0.7353387812407823, -0.6989933350482087, -0.6835224068604273, -0.6921158238785066, -0.7217188264252835, -0.7637517506720419, -0.8057159017858148, -0.8333093620537693, -0.8327870038627241, -0.7931510688939891, -0.7079388773369498, -0.5762895149017982, -0.4032287101039275, -0.19912345762738048, 0.021626092972811716, 0.24243838454530214, 0.4466281803126936, 0.6195670275196116, 0.7505384293302241, 0.8341667424696944, 0.8710515511074273, 0.867618588313726, 0.8350546605288388, 0.7875968290108912, 0.7403153596554869, 0.7065887377614032, 0.6958348088594112, 0.7117510991794384, 0.7514265747295997, 0.8055501080993405, 0.8597172027233948, 0.896672112950365, 0.8992716440220376, 0.8535956532880161, 0.7516973279064126, 0.5935739768219647, 0.3879409425761628, 0.1514795080598367, -0.09323685375808283, -0.32079142716179476, -0.5065138588773618, -0.6300491223171335, -0.6781015202421304, -0.64619431762589, -0.5389832779795898, -0.36913308344851997, -0.15510153259215717, 0.08166236993095077, 0.3196509591252603, 0.5398927777919778, 0.7276930986154884, 0.8734985979773947, 0.9728047077610658, 1.0252642302363124, 1.0333899494712895, 1.0012329554745556, 0.9333027118497857, 0.8339401572384909, 0.7072095654921254, 0.5571462896311223, 0.3881483450425459, 0.20534155782487487, 0.01482887737245796, -0.1764521290488, -0.3611157500299354, -0.5318043493520626, -0.6818066642899347, -0.8054524101831724, -0.8983255342414102, -0.9572814410830893, -0.9802961943453828, -0.9661962276209902, -0.9145882909024544, -0.8259958203690237, -0.702124108056222, -0.5463111553516156, -0.3640099142702318, -0.1630068815984123, 0.04665386649189137, 0.25324056756651203, 0.4443960991039263, 0.6085609531447825, 0.7365289833752492, 0.8228996922007434, 0.8670933837874918, 0.8736111453366721, 0.8515289789816484, 0.8132403002190881, 0.772465080941647, 0.7419679771548864, 0.7313371097907961, 0.7450271466496866, 0.7811915546642222, 0.8315498322037654, 0.8823689588265033, 0.9165305921773814, 0.9163401501954511, 0.866798433796903, 0.7586596196292686, 0.5908492722170399, 0.37178062020046765, 0.11907890680745346, -0.14211821683680798, -0.38238233257874527, -0.5721392733995939, -0.6862057323913836, -0.7079902911617727, -0.6327143381258475, -0.4689575875843263, -0.23816585088733142, 0.02788728184520496, 0.2913733998865506, 0.5138745348418566, 0.6622161891528019, 0.713630396728027, 0.6595409016687056, 0.5072353110800646, 0.2790535214186103, 0.009173689804918802, -0.26151320666451255, -0.49168518087347146, -0.646028784822539, -0.7007240447824197, -0.6471884427151815, -0.493530539618674, -0.2632018631271933, 0.008643095196815533, 0.28067049342689865, 0.5117662020698565, 0.667360375596674, 0.7246614220304907, 0.6758948089830248, 0.5292499968474088, 0.30723953882700833, 0.04292589220225078, -0.22522884697938184, -0.4592044373314265, -0.6269083921942394, -0.7064584618733396, -0.6888404338934664, -0.578411648288706, -0.39139022626549447, -0.15271914914807735, 0.10811456934185323, 0.36154443524920665, 0.5821113615057549, 0.7515472341269214, 0.8606474547165524, 0.9096953707888916, 0.9073268916916939, 0.8684122594374747, 0.8110629523849187, 0.7535131577918508, 0.7111116174600383, 0.6939391865838809, 0.7053500144234236, 0.7415364458091326, 0.7922663020024436, 0.8425535702269459, 0.8751141872059586, 0.8732034679792344, 0.8235993150699542, 0.7190183727683939, 0.5598342988350936, 0.3547305255173707, 0.12000835651727722, -0.12227364288086777, -0.34712620885755746, -0.5299758484536152, -0.6500817333967435, -0.6934598211856411, -0.6548680069310724, -0.538631179832801, -0.35797405653961106, -0.13314154269390344, 0.11150249461783546, 0.3507932103438662, 0.5622006640712187, 0.7287398470888085, 0.8409123226340982, 0.8975410491756267, 0.9052474392037568, 0.8767801125750505, 0.8285828512227308, 0.7778392815717208, 0.7394654445105879, 0.7237013633767214, 0.7343864257619723, 0.7683602106205176, 0.8160146443370595, 0.862832671453382, 0.8918135732392275, 0.8863825849799384, 0.8334021521345413, 0.7256529739097736, 0.5635985512953553, 0.35608386653185525, 0.1195604135723027, -0.12374840459859741, -0.3487502236997944, -0.5308687349642771, -0.6495113130900928, -0.6909901985488635, -0.6504937240912037, -0.5328353201969774, -0.3517349807169625, -0.12783984379196844, 0.11423012543166067, 0.3492730631198282, 0.5549865684462535, 0.7147604584382636, 0.8196924285734603, 0.8692925730239803, 0.8708584840188425, 0.8377913064207088, 0.7870129074549828, 0.7359765930553231, 0.6996793525556969, 0.6881560723752628, 0.7048218776482567, 0.7458257319106636, 0.8006775631265496, 0.853917719961837, 0.8877440401214893, 0.8850693181898429, 0.8326613733709883, 0.7236976539802175, 0.5594490106415803, 0.3497538967519691, 0.11201578047048573, -0.13100695912350224, -0.3542636347146736, -0.5338912711941378, -0.6506028489493497, -0.6922424302133595, -0.6552909494544218, -0.545064832644278, -0.37448254797377645, -0.16191455440330382, 0.07162348789175096, 0.305307696187205, 0.5209397804835978, 0.7045483839307563, 0.8471495500869136, 0.9446334649114675, 0.9967359029755237, 1.0058177131022314, 0.9755714551521117, 0.910087443335543, 0.8133163625595331, 0.6890103411064745, 0.5410140712172831, 0.37367966894661164, 0.19222351735516607, 0.002885008671315868, -0.18723164421141011, -0.3706358231842831, -0.540017664941237, -0.6887965775506286, -0.811456181705438, -0.9037768968384509, -0.9627749707154154, -0.986428591882344, -0.9734798839005043, -0.9233425758887451, -0.8362626385273748, -0.7136342940914308, -0.5585921807071323, -0.37653877807456615, -0.17539608244694269, 0.03449829302119377, 0.24108409799518699, 0.4317114568156308, 0.5946337468390553, 0.7205719868506776, 0.8042233087437884, 0.8452649724027359, 0.8485537347599877, 0.8236121116636361, 0.7832470748996688, 0.7415340851598169, 0.7114139852567443, 0.7023916754066073, 0.7186444625002776, 0.7579146977658392, 0.8114788518364714, 0.865212362785649, 0.9017186145139675, 0.9031789704236397, 0.8546836474975438, 0.7473081616445082, 0.5805118731598218, 0.3633604703375262, 0.11403099657073672, -0.1421571689009856, -0.376100265224383, -0.5591208341865042, -0.66748156416295, -0.6863264429683489, -0.61238919788703, -0.45495950013783854, -0.2348765682622349, 0.018329318180048494, 0.27072256893627067, 0.4888669989484364, 0.6445441082266234, 0.7186091906642366, 0.7032516717681991, 0.602286440359839, 0.4297305321288512, 0.20693427048046936, -0.04118448970582595, -0.2899486028515708, -0.51813884111226, -0.7100679145508004, -0.8564812364022516, -0.954078154354838, -1.004051301932304, -1.0102212014763818, -0.9772535580383042, -0.9093646718646989, -0.8097976595431309, -0.6810878313976068, -0.5258335391357575, -0.34780340225624445, -0.15283789222057037, 0.05073422541995442, 0.25233190333965977, 0.44007238959276546, 0.6022906295601135, 0.7293932651728482, 0.8155001380288734, 0.8596440510683021, 0.8661244160018878, 0.8440053760191001, 0.8057116144877121, 0.7648934322393982, 0.7341019522530025, 0.722408788035578, 0.7335846743805764, 0.76523665163658, 0.8088069415554398, 0.8508057382972929, 0.8750784439185956, 0.8656525197192184, 0.8097364952043214, 0.7004331018480651, 0.5385134797346247, 0.333020638982082, 0.10055243220663874, -0.13684916712333142, -0.3547046170347631, -0.5296187059445376, -0.6427036804094352, -0.6822150791593455, -0.6450059416608724, -0.5366580259087476, -0.37013892662339776, -0.16344566761793425, 0.06325834047144631, 0.29051687792880865, 0.5019090102948002, 0.685337537979504, 0.8332571783100664, 0.9419059935710599, 1.0099338897337269, 1.0368536824281052, 1.0219112826998396, 0.9637216757298569, 0.8608644035958495, 0.7132682495621445, 0.5240958995354725, 0.30150783203128084, 0.05962244367312289, -0.18169903701790627, -0.3985650165893692, -0.5660874768283738, -0.6622779885806316, -0.6721281174161831, -0.5910217986061128, -0.4267122427659796, -0.19931344093386746, 0.06087906417721856, 0.31748163584889194, 0.5333437531858058, 0.6763479522156483, 0.7245443113283739, 0.6697558890344962, 0.5190710655465737, 0.2937181748767438, 0.02576020244976748, -0.24681249668741956, -0.4858948596428177, -0.6588635605451997, -0.7431160183824671, -0.7289134552508003, -0.6200694296515479, -0.4325067812603366, -0.19121024572221312, 0.07400166309693594, 0.3330849816678037, 0.5599873834891823, 0.7359349670621476, 0.8513661111199331, 0.9063246869034065, 0.9094064046484032, 0.8755054075051303, 0.8228032542069148, 0.7695512733800192, 0.7310864566365781, 0.7174344380700259, 0.7318771929311987, 0.770521492507058, 0.8229990169861556, 0.8741669857800006, 0.9065945000702298, 0.9034290410951017, 0.8513488075060012, 0.7431105593701001, 0.5792771762670239, 0.3688585907869233, 0.12855873457058717, -0.11905374155741394, -0.348465451110149, -0.5346000660767498, -0.6563026294503328, -0.6993804544754962, -0.6586232637177873, -0.5386587210945445, -0.35325412329016936, -0.12340944757935825, 0.12562838916868907, 0.3678984527083349, 0.5802535686096911, 0.7453566040596344, 0.8536797217461267, 0.904341743696613, 0.9045288934223483, 0.8678005605218305, 0.8115232656672823, 0.7538338251356304, 0.7106289265654393, 0.6929469282521439, 0.7051665302164144, 0.7441987520198292, 0.7999632255413621, 0.8568697593576841, 0.8963183241181077, 0.8998019936252488, 0.8522424023181564, 0.7449696798222867, 0.5778551163588856, 0.3603125530553699, 0.11070054945898282, -0.14570230635299203, -0.3799809948767624, -0.5637043781173343, -0.6732548027150764, -0.693664788209523, -0.6213306289901542, -0.46505052769065697, -0.24516543111583403, 0.0090596915946915, 0.2635428251223252, 0.48417637041829653, 0.641689526437302, 0.7157173189250563, 0.6973828411174359, 0.5901314098610099, 0.4086428546496129, 0.17619718572689294, -0.07917988137166046, -0.328937783780878, -0.5480728892646238, -0.7183409139718169, -0.830216292312652, -0.8834929518448947, -0.8862829283786646, -0.8529835994516479, -0.8013536812216641, -0.7493136237212195, -0.711957955660661, -0.6991338441055578, -0.7139427031909754, -0.7523268372875261, -0.8037761996631599, -0.8530893578229929, -0.8828792296977179, -0.8764987725251604, -0.8209490836280732, -0.7093747657586275, -0.5427215391631399, -0.33033331822457584, -0.08916763854378294, 0.15803966171501063, 0.3856904000524847, 0.5687642313471672, 0.6864040238926279, 0.724868684652829, 0.6795420414253549, 0.5557211678730963, 0.3677696222282419, 0.13706564016321376, -0.11113892216576668, -0.3513165038596046, -0.5611655218564168]}] caption="Constellation Graph"
  out "Sync Found 4":bool=TRUE
  out "Correct Packets Rx 4":i16=46
  out "Singal & Noise Power 4":cluster{"signal_power":dbl, "noise_power":dbl}={"signal_power"=0.000719802679436105, "noise_power"=8.71918670194843e-09}
  out "error out 7":errorcluster
  out "Cumulative Packets Recovered 4":i16(graph)=46
  out "Signal and Noise Power Tracking 4":cluster{"total_power":dbl, "noise_power":dbl}(graph)={"total_power"=0.000719802679436105, "noise_power"=8.71918670194843e-09}
  in  "stop 2":bool caption="stop"
  out "Symbol Rate\n[symbols/sec] 4":dbl=25000.0 format="%#.6p"
  out "Constellation Graph 4":T8(graph) caption="Constellation Graph"
  in  "autoscale 2":bool caption="autoscale"
  in  "Tab Control 4":T9(tab)
  in  "Packet Parameters 4":T10={"Guard Bits "=30, "Sync Bits"=20, "Message Bits"=128}
  in  "Packet Pad \n[samples] 2":i32=200
  in  "Blank Frame \n[samples] 2":i32=500
  out "Number of Packets in Message 2":i32=46
  in  "PN sequence order\nfor Sync Bits 2":i32=31 caption="PN sequence order (9)"
  in  "Packet Repeat 2":i32=2
  in  "Select PSK Modulation Format 2":T4(tab)=enum."QPSK" caption="PSK"
  in  "BPSK System Parameters 4":T5={"Samples per Symbol"=8, "symbol map"=[], "Differential PSK"=enum."disable", "PSK type"=0} caption="BPSK System Parameters" {"PSK type" items=["normal", "shifted", "offset"]; "symbol map" format="%.3f"}
  in  "QPSK System Parameters 4":T5={"Samples per Symbol"=8, "symbol map"=[], "Differential PSK"=enum."disable", "PSK type"=0} caption="QPSK System Parameters" {"PSK type" items=["normal", "shifted", "offset"]; "symbol map" format="%.3f"}
  in  "pi/4 DQPSK System Parameters 4":T5={"Samples per Symbol"=8, "symbol map"=[], "Differential PSK"=enum."enable", "PSK type"=1} caption="pi/4 DQPSK System Parameters" {"PSK type" items=["normal", "shifted", "offset"]; "symbol map" format="%.3f"}
  in  "OQPSK System Parameters 4":T5={"Samples per Symbol"=8, "symbol map"=[], "Differential PSK"=enum."disable", "PSK type"=2} caption="OQPSK System Parameters" {"PSK type" items=["normal", "shifted", "offset"]; "symbol map" format="%.3f"}
  in  "8-PSK System Parameters 4":T5={"Samples per Symbol"=8, "symbol map"=[], "Differential PSK"=enum."disable", "PSK type"=0} caption="8-PSK System Parameters" {"PSK type" items=["normal", "shifted", "offset"]; "symbol map" format="%.3f"}
  in  "16-PSK System Parameters 4":T5={"Samples per Symbol"=8, "symbol map"=[], "Differential PSK"=enum."disable", "PSK type"=0} caption="16-PSK System Parameters" {"PSK type" items=["normal", "shifted", "offset"]; "symbol map" format="%.3f"}
  in  "M 4":i32=4 caption="M" min=2 step=2
  in  "Custom System Parameters 4":T5={"Samples per Symbol"=8, "symbol map"=[], "Differential PSK"=enum."disable", "PSK type"=0} caption="Custom System Parameters" {"PSK type" items=["normal", "shifted", "offset"]; "symbol map" format="%.3f"}
  in  "Pulse Shaping Filter Parameters 2":T6={"Alpha"=0.5, "Filter Length"=6, "TX Filter"=enum."Root Raised Cos"} caption="Pulse Shaping Filter" {"Alpha" format="%.2f"}
  in  "Tx Parameters 2":T11={"Tx IQ Sampling\nRate [s/sec]"=500000.0, "Tx Frequency [Hz]"=2500000000.0, "Tx Gain [dB]"=0.0, "Tx Antenna"="TX1"} {"Tx Gain [dB]" format="%#.6p"; "Tx Frequency [Hz]" format="%#.6p"; "Tx IQ Sampling\nRate [s/sec]" format="%#.6p"}
  out "Actual Tx Parameters 2":T11={"Tx IQ Sampling\nRate [s/sec]"=200000.0, "Tx Frequency [Hz]"=2500000000.0, "Tx Gain [dB]"=0.0, "Tx Antenna"="TX1"} {"Tx Gain [dB]" format="%#.6p"; "Tx Frequency [Hz]" format="%#.6p"; "Tx IQ Sampling\nRate [s/sec]" format="%#.6p"}
  out "error out 4":errorcluster
  in  "Queue Length 2":i32=10
  out "x .or. y? 2":bool
  in  "synchronization parameters 2":T1={"expected sync location (symbols)"=-1, "sync sequence"=[], "sync location uncertainty (symbols)"=0, "sync indent (symbols)"=0} caption="synchronization parameters" {"sync sequence" format="%.2f"}
  in  "Tab Control 3":T2(tab)=enum."Rx Display"
  in  "Acquisition Duration [sec] 2":dbl=0.04 format="%#.6p"
  in  "Rx Parameters 2":T3={"Rx IQ Sampling\nRate [s/sec]"=500000.0, "Rx\nFrequency [Hz]"=915000000.0, "Rx Gain [dB]"=20.0, "Rx Antenna"="RX1"} {"Rx Gain [dB]" format="%#.6p"; "Rx\nFrequency [Hz]" format="%#.6p"; "Rx IQ Sampling\nRate [s/sec]" format="%#.6p"}
  out "Actual Rx Parameters  2":T3={"Rx IQ Sampling\nRate [s/sec]"=500000.0, "Rx\nFrequency [Hz]"=915000000.0, "Rx Gain [dB]"=20.0, "Rx Antenna"="RX1"} {"Rx Gain [dB]" format="%#.6p"; "Rx\nFrequency [Hz]" format="%#.6p"; "Rx IQ Sampling\nRate [s/sec]" format="%#.6p"}
  out "Symbol Rate\n[symbols/sec] 3":dbl=62500.0 format="%#.6p"
  in  "Choose a PSK Format 2":T4(tab)=enum."QPSK" caption="PSK"
  in  "BPSK System Parameters 3":T5={"Samples per Symbol"=8, "symbol map"=[], "Differential PSK"=enum."disable", "PSK type"=0} caption="BPSK System Parameters" {"PSK type" items=["normal", "shifted", "offset"]; "symbol map" format="%.3f"}
  in  "QPSK System Parameters 3":T5={"Samples per Symbol"=8, "symbol map"=[], "Differential PSK"=enum."disable", "PSK type"=0} caption="QPSK System Parameters" {"PSK type" items=["normal", "shifted", "offset"]; "symbol map" format="%.3f"}
  in  "pi/4 DQPSK System Parameters 3":T5={"Samples per Symbol"=8, "symbol map"=[], "Differential PSK"=enum."enable", "PSK type"=1} caption="pi/4 DQPSK System Parameters" {"PSK type" items=["normal", "shifted", "offset"]; "symbol map" format="%.3f"}
  in  "OQPSK System Parameters 3":T5={"Samples per Symbol"=8, "symbol map"=[], "Differential PSK"=enum."disable", "PSK type"=2} caption="OQPSK System Parameters" {"PSK type" items=["normal", "shifted", "offset"]; "symbol map" format="%.3f"}
  in  "8-PSK System Parameters 3":T5={"Samples per Symbol"=8, "symbol map"=[], "Differential PSK"=enum."disable", "PSK type"=0} caption="8-PSK System Parameters" {"PSK type" items=["normal", "shifted", "offset"]; "symbol map" format="%.3f"}
  in  "16-PSK System Parameters 3":T5={"Samples per Symbol"=8, "symbol map"=[], "Differential PSK"=enum."disable", "PSK type"=0} caption="16-PSK System Parameters" {"PSK type" items=["normal", "shifted", "offset"]; "symbol map" format="%.3f"}
  in  "M 3":i32=4 caption="M" min=2 step=2
  in  "Custom System Parameters 3":T5={"Samples per Symbol"=8, "symbol map"=[], "Differential PSK"=enum."disable", "PSK type"=0} caption="Custom System Parameters" {"PSK type" items=["normal", "shifted", "offset"]; "symbol map" format="%.3f"}
  in  "filter parameters 2":T6={"Alpha"=0.5, "Filter Length"=6, "TX Filter"=enum."Root Raised Cos"} caption="Matching Filter Parameters" {"Alpha" format="%.2f"}
  in  "PN Sequence Order\nfor Sync 2":i32=31
  in  "Packet Parameters 3":T7={"Guard Bits "=30, "Sync Bits"=20, "Message Bits"=128, "Number of Packets \nto Expect"=46}
  out "Recovered Message 2":string="Two roads diverged in a yellow wood,\nAnd sorry I could not travel both\nAnd be one traveler, long I stood\nAnd looked down one as far as I could\nTo where it bent in the undergrowth.\n\nThen took the other, as just as fair,\nAnd having perhaps the better claim,\nBecause it was grassy and wanted wear;\nThough as for that the passing there\nHad worn them really about the same.\n\nAnd both that morning equally lay\nIn leaves no step had trodden black.\nOh, I kept the first for another day!\nYet knowing how way leads on to way,\nI doubted if I should ever come back.\n\nI shall be telling this with a sigh\nSomewhere..."
  out "Received Signal (Raw) 2":dbl[](graph)
  out "Constellation Graph 3":T8(graph)=[{"Decimated Array"=[-0.6804993103727607, -0.6771092058245918, -0.6428257187708691, 0.7259219405542873, 0.7311366832454209, -0.6450362325295403, -0.658892442379921, -0.6855840493085356, -0.646998431742077, -0.6568678904388265, 0.7432214399633668, -0.6618522924674632, -0.6753922285302938, 0.6950905811428861, 0.7248141384495557, 0.7218255862492685, 0.704818637196686, 0.7027336696732543, 0.7016253671990413, 0.7082534735709545, 0.7084209330001522, 0.7036372125301554, 0.7010930640613204, 0.7075984577478206, 0.7100058187983528, 0.7171431626733421, 0.7279231861183771, 0.6959557947635676, -0.7024336186443912, -0.7110189818905128, 0.6934234462727887, 0.7327126116070742, 0.7051667045224878, 0.690798979580973, -0.6877839781333666, 0.6889445287579181, 0.716354235720989, -0.706071092371314, 0.72195318833854, -0.7119212984185137, 0.7223509528651848, -0.7244956435522718, -0.6716656585292338, -0.7182056308592257, 0.724421589775866, -0.6763390206227603, 0.7587597202334532, -0.6966306246608392, -0.6999692828092537, -0.7056805503027465, 0.7430994824068496, 0.7108305621069824, 0.7197425435843314, -0.7051937005816177, -0.6734048186040171, -0.6909214820858487, 0.7004218263991402, -0.6889802592692622, 0.7244882842042791, 0.7027757047403482, -0.7012448562483489, -0.6963431828766949, 0.7166197717755273, 0.7431431506248717, 0.7233235134334371, 0.6983161172439467, 0.7059749857271942, -0.6872358926309042, 0.6918268533027474, -0.7138701729016586, -0.6801285945135653, 0.7195044185357663, 0.6810587309328351, -0.6856313040037053, -0.7011043347997452, 0.6920652628903768, -0.7080955978852922, -0.6860253207439192, -0.7101309321759165, 0.7212965033681705, 0.6967245108747491, 0.7128097205123256, 0.6657328144726218, 0.6985573048815797, 0.6967609587320983, 0.720489591403177, -0.6992149062771553, 0.6810319795543738, -0.7124274384065621, -0.6689704942642202, 0.7017697482270308, 0.7036983705130238, -0.69378287602043, -0.6926507402482928, 0.6832891050414109, 0.7219614630178657, 0.7044242088089868, 0.6722056874933439, -0.6818156450864503, 0.6786113633855301, 0.7039257931121476, -0.6836867328922335, 0.6967676536286352, -0.7018627722542645, 0.7033449800412358, -0.7121625353086042], "Decimated Array"=[0.7327573786203745, 0.7417811878517194, -0.6799031648608087, -0.7111421642681004, -0.727382953469249, -0.6704579022356528, -0.6770604606987946, 0.7538529097411865, -0.6722715103438465, -0.6756211416707443, -0.6914774106844375, -0.673529581873597, 0.7393627898718214, 0.7522557788351737, 0.7435736461024193, 0.7257726558576425, 0.7275033865931528, 0.7311828384458046, 0.7293390182016347, 0.7220976758138733, 0.7195981106474233, 0.7211811690986409, 0.7188051788075457, 0.7320183145085448, 0.6962181897094762, 0.7305998791526044, -0.6967382767827438, 0.7159339540668409, -0.7008762468325049, 0.7525668303202456, 0.7058888207208955, 0.7252589385855543, -0.7159704258460882, 0.7370284868429373, 0.7140037167311404, 0.7389767670280546, -0.6960013467696725, 0.7235856630223708, -0.6972846806923089, -0.657884155216942, -0.6949224336608516, 0.7453870445521058, -0.6844918028247094, -0.6835224068604273, -0.7079388773369498, 0.7505384293302241, 0.6958348088594112, 0.7516973279064126, -0.6781015202421304, 0.7276930986154884, 0.7072095654921254, -0.6818066642899347, -0.702124108056222, 0.7365289833752492, 0.7313371097907961, 0.7586596196292686, -0.7079902911617727, 0.713630396728027, -0.7007240447824197, 0.7246614220304907, -0.7064584618733396, 0.7515472341269214, 0.6939391865838809, 0.7190183727683939, -0.6934598211856411, 0.7287398470888085, 0.7237013633767214, 0.7256529739097736, -0.6909901985488635, 0.7147604584382636, 0.6881560723752628, 0.7236976539802175, -0.6922424302133595, 0.7045483839307563, 0.6890103411064745, -0.6887965775506286, -0.7136342940914308, 0.7205719868506776, 0.7023916754066073, 0.7473081616445082, -0.6863264429683489, 0.7186091906642366, -0.7100679145508004, -0.6810878313976068, 0.7293932651728482, 0.722408788035578, 0.7004331018480651, -0.6822150791593455, 0.685337537979504, 0.7132682495621445, -0.6721281174161831, 0.7245443113283739, -0.7431160183824671, 0.7359349670621476, 0.7174344380700259, 0.7431105593701001, -0.6993804544754962, 0.7453566040596344, 0.6929469282521439, 0.7449696798222867, -0.693664788209523, 0.7157173189250563, -0.7183409139718169, -0.6991338441055578, -0.7093747657586275, 0.724868684652829]}, {"Decimated Array"=[-0.6804993103727607, -0.6762349965387238, -0.6685108157798112, -0.6587623289821404, -0.6494739544100483, -0.6438465750011458, -0.645155862498135, -0.6559333949667008, -0.6771092058245918, -0.707329395010057, -0.7427108893571827, -0.7768816274525345, -0.8016064503455926, -0.8078913118575249, -0.7873020181422804, -0.7333876332701184, -0.6428257187708691, -0.5161117575568228, -0.35777203758853365, -0.17570329650700167, 0.01987541369217473, 0.21778298257008183, 0.4072432109758152, 0.5789865397268567, 0.7259219405542873, 0.8433225109633283, 0.9285347773827741, 0.9803625623365572, 0.9983411710644498, 0.9823024312079763, 0.9321501534368272, 0.8480801425231922, 0.7311366832454209, 0.5839247754585907, 0.41126876723240074, 0.2204206478178329, 0.020932943403138903, -0.1761332529377578, -0.3593512576776315, -0.5183227318987554, -0.6450362325295403, -0.7348944300155227, -0.7873580245691122, -0.8057437870339258, -0.7965717988687436, -0.7684407927742708, -0.7306238606226202, -0.6917860656058442, -0.658892442379921, -0.6364690666334113, -0.6263656338128196, -0.6279033391241801, -0.6383295002999582, -0.6535857140497858, -0.6691389263327601, -0.6808303682804338, -0.6855840493085356, -0.6819546232796994, -0.6704727894453094, -0.6535744314745204, -0.6353365462635079, -0.6208696353048802, -0.6154307523642993, -0.6233724286798671, -0.646998431742077, -0.6855864576394015, -0.7347128803667217, -0.7860882541221362, -0.8282453730286534, -0.8479309126781169, -0.8321007406466316, -0.7702787309009056, -0.6568678904388265, -0.4928870454737699, -0.286812316855307, -0.054181947000257816, 0.18398541460571163, 0.403912791430555, 0.5822957160369652, 0.6996654194867074, 0.7432214399633668, 0.7085518372290116, 0.6001271112229511, 0.43028071322686884, 0.21712133759522834, -0.01828477060583316, -0.25486167705907176, -0.474106655260725, -0.6618522924674632, -0.8090041994597156, -0.9113555181844136, -0.9685514235160106, -0.9827395175415803, -0.9572113882143858, -0.8953875269303032, -0.8004356628744611, -0.6753922285302938, -0.5237515103490776, -0.3502005293644506, -0.1611351791820148, 0.03517140208780353, 0.22893110044459927, 0.40972263321669966, 0.5677345648283395, 0.6950905811428861, 0.7869683371034619, 0.8423038906676682, 0.8638849324516561, 0.8577538092414735, 0.8321468933549871, 0.7961070317612736, 0.7580880124868856, 0.7248141384495557, 0.7005277134039959, 0.686923334338586, 0.6833877232132058, 0.6876280888811944, 0.6964899036822818, 0.706747954834772, 0.7157647696850384, 0.7218255862492685, 0.724268969267967, 0.7234261321898535, 0.7202619630220548, 0.7159731242866095, 0.7116890979547664, 0.7082240869885714, 0.70594341514383, 0.704818637196686, 0.7045271958113069, 0.7047088927454438, 0.7050023859293303, 0.7051255773761397, 0.7049541452505861, 0.7044514570052206, 0.7036747950662702, 0.7027336696732543, 0.7017628701423971, 0.7009138948889888, 0.7003118882562483, 0.7000261021126073, 0.7000875017890581, 0.7004449481097869, 0.7009932809698078, 0.7016253671990413, 0.702221540251104, 0.7027618684813808, 0.7032916906181711, 0.7038854962099375, 0.7046487256800136, 0.7056308879137863, 0.7068515417419651, 0.7082534735709545, 0.7096888191782372, 0.7109913402244956, 0.7119894724643936, 0.7124890080936077, 0.7123827414517839, 0.7116323891766451, 0.7102633952930952, 0.7084209330001522, 0.7063057748688335, 0.7042562032788021, 0.7025954190884202, 0.7015546954049546, 0.7012557549487087, 0.7016448259380934, 0.7025398218482226, 0.7036372125301554, 0.7046321819639692, 0.7053295412842902, 0.7055972799037947, 0.705357986716468, 0.7046523984817116, 0.7036068751653552, 0.7023536981462808, 0.7010930640613204, 0.7000326295845363, 0.6993965049981011, 0.6993226127993213, 0.6998881120919372, 0.701113074412268, 0.7029138523453567, 0.7051416575412044, 0.7075984577478206, 0.710078980444559, 0.7123321038850414, 0.7140736603763724, 0.7150314533562983, 0.7150214932752349, 0.7140093308210059, 0.7121877418723002, 0.7100058187983528, 0.70805206355385, 0.7070027727419878, 0.7073212689161522, 0.7091056294101988, 0.7119833987327618, 0.7150644848824459, 0.7171668570713718, 0.7171431626733421, 0.71423133689185, 0.7085192919358748, 0.7011650150275229, 0.6943243914091253, 0.6909299894216554, 0.694045612210552, 0.706066960259486, 0.7279231861183771, 0.7583890909767882, 0.7938021658029275, 0.8279962238841705, 0.8528896550258644, 0.8595701988778817, 0.8395633321459017, 0.7862278633870129, 0.6959557947635676, 0.5689496495122442, 0.4094105630569515, 0.22502717825358973, 0.025894312218078558, -0.17672464042078925, -0.37176542586543576, -0.5495413422869474, -0.7024336186443912, -0.8251771287794907, -0.9146738107129905, -0.9693864660264264, -0.9886486884020281, -0.9721997012143947, -0.920010882437784, -0.8324905468768208, -0.7110189818905128, -0.5586215402038113, -0.38057133580870495, -0.18461757845785642, 0.019294891934465676, 0.2197963582992338, 0.4053691867674974, 0.5657713716359056, 0.6934234462727887, 0.7843501298361789, 0.8386729718179944, 0.8602628823550353, 0.855774513907276, 0.8333154686311419, 0.8010170366525857, 0.7658225991667146, 0.7327126116070742, 0.7045406905991981, 0.6824916000019303, 0.6667964864918056, 0.6575588911889615, 0.6553991485314229, 0.6616300661715835, 0.677865934701111, 0.7051667045224878, 0.7429233296416752, 0.7878677137961015, 0.8333853282559609, 0.8696348770191419, 0.8846190114381185, 0.8659756375138661, 0.8033400824826783, 0.690798979580973, 0.5288571353054295, 0.32551133007737276, 0.09595098720473762, -0.13906888290440567, -0.35588344294942403, -0.5312979803398246, -0.646084108275294, -0.6877839781333666, -0.6524636145322816, -0.5450893812430798, -0.37828756856953233, -0.17009276356333847, 0.0590247558982818, 0.28912715162217667, 0.5032762839933951, 0.6889445287579181, 0.8383428746399739, 0.9477025130341128, 1.015790170453614, 1.0423483901645878, 1.0268512388275022, 0.9680879161655901, 0.8646551393981081, 0.716354235720989, 0.5260764152807655, 0.30160439840294034, 0.05668512406955431, -0.18910351581760784, -0.4118751751084471, -0.5863423085037114, -0.6897554505434935, -0.706071092371314, -0.6295185621493208, -0.4668637151478481, -0.23765972556227086, 0.027714817455610417, 0.29202447870753795, 0.5167154122972588, 0.6679084709283569, 0.72195318833854, 0.6695114009171929, 0.5175155629675429, 0.2883041299697019, 0.01623720013151288, -0.25755900242514196, -0.4917082138253101, -0.6510176327160702, -0.7119212984185137, -0.6659995880876536, -0.5209852917537516, -0.2992839322286186, -0.03416997277404838, 0.2355466281568285, 0.4714352113659737, 0.6410442893752866, 0.7223509528651848, 0.7062991907811851, 0.5973003486423586, 0.4116890808688979, 0.17445466790696096, -0.08489625696410336, -0.3368901331962952, -0.5561324114364461, -0.7244956435522718, -0.832904063982776, -0.8817003370505312, -0.8795283892255058, -0.841156501109088, -0.7846263716950196, -0.7281214416972949, -0.6870445779683771, -0.6716656585292338, -0.6855631019709484, -0.7251869491105687, -0.7803544807713914, -0.8357414937022205, -0.8732615963603204, -0.8749681769421048, -0.8261602248386887, -0.7182056308592257, -0.5506938062457699, -0.3325933377055765, -0.08189760414583691, 0.17618237159000388, 0.4123697444728759, 0.5974694739328056, 0.7068084628379865, 0.724421589775866, 0.6461724854013321, 0.4812775786848407, 0.25159361606242997, -0.011058078343011023, -0.2692923486046545, -0.48569025029571594, -0.6284581525739953, -0.6763390206227603, -0.6219818356022658, -0.47306441806801147, -0.2510857990405568, 0.01202477775150253, 0.27875734553572085, 0.5116930035471384, 0.6789865139576629, 0.7587597202334532, 0.7418192787585248, 0.6323458533022597, 0.446406792743502, 0.20878035238051276, -0.05119783320575381, -0.3042611875270661, -0.5253152667965498, -0.6966306246608392, -0.8095606744479041, -0.8647740627418172, -0.870930075780708, -0.8423384959975685, -0.7960318277718325, -0.7486596019303445, -0.7137982795070836, -0.6999692828092537, -0.7095971091381883, -0.7390816485119921, -0.7796138336185289, -0.818762813999536, -0.8425904879324037, -0.8378822227707572, -0.7942341058424417, -0.7056805503027465, -0.571726769560303, -0.39765177441111643, -0.19391837432237818, 0.025178720377377686, 0.24333379676657457, 0.44433965307888695, 0.6142375047967751, 0.7430994824068496, 0.8263038750024307, 0.8650100488333368, 0.8657148042767202, 0.8390794723757462, 0.7981161813167071, 0.7560954579232749, 0.7244176046468488, 0.7108305621069824, 0.718204650734365, 0.7441150394580835, 0.7812106743682087, 0.8183931962770272, 0.8425254654823089, 0.8406177118076219, 0.8019301699596733, 0.7197425435843314, 0.5926686710089698, 0.4251140503775492, 0.22683136067452989, 0.011660330280988253, -0.20423795622266205, -0.4045792942890271, -0.57504838691632, -0.7051937005816177, -0.7897661684393493, -0.8293068652572223, -0.8299006515155186, -0.8021229049955473, -0.7594233513128958, -0.715953221878639, -0.684307426439313, -0.6734048186040171, -0.6868570522140265, -0.7221874426788824, -0.7708237442647581, -0.8191585903691571, -0.8505818015508355, -0.8481661462885941, -0.7977634650762118, -0.6909214820858487, -0.5271825682100394, -0.31525436879598623, -0.07267661804829456, 0.17610311762416703, 0.4028796348907104, 0.5798206568779839, 0.6838352068807156, 0.7004218263991402, 0.6263585027788804, 0.4707037347107586, 0.2537801245269521, 0.004363575376446024, -0.244425088845282, -0.45988451941533137, -0.6143614233710846, -0.6889802592692622, -0.675810131006379, -0.5782280367437729, -0.40962067096108434, -0.19054676255841746, 0.05481291967260732, 0.3023001215109928, 0.5308329677888366, 0.7244882842042791, 0.8734246012838044, 0.9735701497284382, 1.0253939516322779, 1.0322709072595566, 0.9989018615889086, 0.9300855209250758, 0.8301278260930205, 0.7027757047403482, 0.5516545283139476, 0.38091449347590134, 0.19570631362414656, 0.002354352790910658, -0.19179798997086855, -0.3788570549590451, -0.5510272450358933, -0.7012448562483489, -0.8236915392774603, -0.914039706142418, -0.9694184170252935, -0.9881756409826234, -0.9696303075716558, -0.913918517626886, -0.8220829857364051, -0.6963431828766949, -0.5405016807251724, -0.36031892603430715, -0.16359224329210514, 0.04013418091790215, 0.24018456190270834, 0.425760423266114, 0.5870829268985424, 0.7166197717755273, 0.8099833426954562, 0.8664917523906949, 0.8890606065456064, 0.8835329376488369, 0.8577948250420299, 0.8205354221662687, 0.7800304020582047, 0.7431431506248717, 0.7146443568705966, 0.6969512334183051, 0.6901074157262647, 0.6922880175560046, 0.7003398356906728, 0.7105226229352982, 0.7191652725013788, 0.7233235134334371, 0.7213381284523223, 0.7131072858574705, 0.7002046822080928, 0.6857438943908143, 0.6739876200747604, 0.6696394639541572, 0.6768836675096863, 0.6983161172439467, 0.7338690127516884, 0.7800774899548244, 0.829602819630056, 0.8715371312486556, 0.892620000492053, 0.8790856399483223, 0.8192212166031462, 0.7059749857271942, 0.5391749210900726, 0.3269503040314498, 0.08573815461541592, -0.1612255824786287, -0.386730293143399, -0.5635326559438285, -0.6686383256247854, -0.6872358926309042, -0.6156114857935734, -0.4623211423735695, -0.24733010394610414, 0.0007198102460047476, 0.24863863484628498, 0.4635514254715547, 0.6176104623364325, 0.6918268533027474, 0.6782756201030052, 0.5805134425392992, 0.41210610757403726, 0.19372452237290802, -0.050391409713054024, -0.29611210645789393, -0.5225111093000552, -0.7138701729016586, -0.8605441211993027, -0.9585448112667802, -1.008414026021156, -1.0135648241052666, -0.978745896542667, -0.9087849082692102, -0.8079881948321259, -0.6801285945135653, -0.5287862221062773, -0.35805233939202374, -0.1729861888667504, 0.020116186161511587, 0.21387335563181437, 0.40025748153323093, 0.5712472743319003, 0.7195044185357663, 0.8388895884119506, 0.9249072134737321, 0.9746853929178996, 0.9868923875604191, 0.9616684243967665, 0.9003848901697228, 0.8056175444681817, 0.6810587309328351, 0.5314881726723011, 0.3626554692436761, 0.18103860407685468, -0.006510589607727805, -0.1931114704827839, -0.3722848897831801, -0.5381718770034626, -0.6856313040037053, -0.8101801487665511, -0.9076732803716326, -0.9739618526107378, -1.004716020345832, -0.9956414793795033, -0.9430154749490675, -0.8446500281072215, -0.7011043347997452, -0.516842399364099, -0.3010204717594881, -0.06763754580789842, 0.16514820448340978, 0.37668157665933155, 0.5461920463765456, 0.655552915260347, 0.6920652628903768, 0.6505655304034257, 0.5346883243834851, 0.35661897243093144, 0.13559774776324776, -0.1046718797566402, -0.3394032573081613, -0.5461789593962133, -0.7080955978852922, -0.8157954529602021, -0.8683801331865292, -0.8727983131028657, -0.8421078226859732, -0.7927582081222804, -0.741572331068595, -0.7028423018527019, -0.6860253207439192, -0.6943551977069015, -0.7245345157854167, -0.7675646042411391, -0.8104296201087327, -0.8383601072014226, -0.8373952185694984, -0.7966528302359737, -0.7101309321759165, -0.5776984378988999, -0.40521323182553737, -0.2036592543667804, 0.012419924984258368, 0.22695341747885692, 0.42449093142276867, 0.592188438033417, 0.7212965033681705, 0.8079364234726191, 0.8532668165288172, 0.8627953034872611, 0.8451288060001957, 0.8104079963441455, 0.7687359339278867, 0.7287670505538517, 0.6967245108747491, 0.6759780606536095, 0.667107406232625, 0.6684364317450245, 0.676784919616326, 0.6884291860003884, 0.699890853611944, 0.7085144901744879, 0.7128097205123256, 0.7124229876828518, 0.7080187790236897, 0.7008050101089057, 0.6921805709227881, 0.6834646736814466, 0.6757033963031507, 0.669648508318143, 0.6657328144726218, 0.6642652636337992, 0.6653767657521718, 0.6690028595853793, 0.674775333959487, 0.6819477949985021, 0.6893278789128267, 0.6953927726157616, 0.6985573048815797, 0.697578095425808, 0.6920506573747554, 0.6828307951888688, 0.6722732265164824, 0.6640958466160822, 0.6627912256868634, 0.6726965874495441, 0.6967609587320983, 0.735252994349721, 0.7847852487718341, 0.837860611588047, 0.8832021671865116, 0.9070282265831913, 0.8950883370622812, 0.8352994933427401, 0.720489591403177, 0.5506306635171825, 0.3342725070105252, 0.08840692523651153, -0.16315427404215097, -0.3926718560799536, -0.572539734272038, -0.6796338477180948, -0.6992149062771553, -0.6277630208203462, -0.4741131473050659, -0.2585293695095081, -0.009930257048617025, 0.23830892263310452, 0.45325402085890604, 0.607121618765611, 0.6810319795543738, 0.6672310461853316, 0.5694827757707117, 0.4015147931896041, 0.1841817171712272, -0.05817646638242799, -0.3014136753019013, -0.524665532969832, -0.7124274384065621, -0.855285246094759, -0.9495933688767533, -0.996236130847489, -0.9989838487955423, -0.9628841324499167, -0.8930056180780918, -0.7937877561121499, -0.6689704942642202, -0.5220072798874036, -0.3566099133872175, -0.17731129436958973, 0.010268861422383327, 0.19945198638565087, 0.3827826926443024, 0.5526251582270405, 0.7017697482270308, 0.8239876507426606, 0.9144785689512498, 0.9699591512942685, 0.9886252045487814, 0.9700306803372667, 0.9149020439452162, 0.825116863065968, 0.7036983705130238, 0.554839481392563, 0.3840291620621759, 0.19787647745423148, 0.003860727052948984, -0.18999525295737457, -0.3757044734833313, -0.5458056810042837, -0.69378287602043, -0.814366828718361, -0.9036469275456485, -0.9588849469775574, -0.9783006504455267, -0.960973889608092, -0.9067746467203663, -0.8165903751017708, -0.6926507402482928, -0.5388812935652539, -0.361228905014989, -0.16771060388912773, 0.031903370124330505, 0.22678679843602859, 0.4061707941853134, 0.5606402717569381, 0.6832891050414109, 0.7705901219032752, 0.8228006526178891, 0.8436430103344122, 0.8394755303225311, 0.8180394512925253, 0.7871333265278456, 0.7534665911565442, 0.7219614630178657, 0.695510686451852, 0.6753252498343544, 0.6615878037807406, 0.6542998195364643, 0.6538606147644473, 0.6612723675386262, 0.6778625191525914, 0.7044242088089868, 0.7402649399766673, 0.7822594926239343, 0.8241634231439008, 0.8566831085547093, 0.8684082810681567, 0.8475040183712003, 0.784012885063017, 0.6722056874933439, 0.5125005393952523, 0.31260026449095785, 0.08722135068631567, -0.14339658857823498, -0.35611765704885123, -0.5282733760242059, -0.6409441045045646, -0.6818156450864503, -0.6469272017629891, -0.5410574986904879, -0.37652152921039295, -0.17097947697100876, 0.05541171165914345, 0.2829619347828144, 0.49484727767121917, 0.6786113633855301, 0.8264573551553331, 0.9345361200971587, 1.0015661687984379, 1.0272888190262575, 1.0112965146842847, 0.952583288738177, 0.8500890658990591, 0.7039257931121476, 0.5171900515296706, 0.29764273007471115, 0.05870661463653025, -0.1806017914741214, -0.39721826601913907, -0.5668036345777544, -0.6674573482841338, -0.6836867328922335, -0.6099467963750959, -0.4528161959244535, -0.23123780147788525, 0.0254037230819288, 0.2810884215045038, 0.4984727203603391, 0.6447055580185417, 0.6967676536286352, 0.6455398584402634, 0.4976568874522828, 0.2746594289249686, 0.009825427460916032, -0.25698435822392646, -0.4855514161032739, -0.6415528231225354, -0.7018627722542645, -0.6580125604775775, -0.517265265222927, -0.30121265695938104, -0.04212438479079229, 0.22217065809727116, 0.45405673442103006, 0.6217149465148919, 0.7033449800412358, 0.6897787566619501, 0.5850104229528822, 0.4047415306155254, 0.17323834921239678, -0.08075812096424864, -0.3284327261412435, -0.5448733152596168, -0.7121625353086042, -0.8211818337976253, -0.8719691969355644, -0.8727186157199347, -0.8376486334880819, -0.7842590106698991, -0.7303274268398209, -0.6909814362358659], "Decimated Array"=[0.7327573786203745, 0.8571160437398065, 0.9481227692632541, 1.003980881033979, 1.0238155370523472, 1.0072368286759465, 0.9541994905916551, 0.8651912730450063, 0.7417811878517194, 0.5871636451740783, 0.40676677760888635, 0.20846130324205578, 0.0022318875001048045, -0.2005410967663612, -0.38829860023304064, -0.5506845398656813, -0.6799031648608087, -0.7716987861234258, -0.8258475294329478, -0.8459996756657396, -0.8388616433189412, -0.8130753155007096, -0.7778435482452709, -0.7416372990136377, -0.7111421642681004, -0.6905831950739342, -0.6815454430666558, -0.6831516021872707, -0.6925669267273694, -0.7057731727702966, -0.7184007879882285, -0.7265282476091678, -0.727382953469249, -0.7198001905615271, -0.7045629848520147, -0.6843705475932246, -0.6634185556136458, -0.646887119577886, -0.6400361359583534, -0.6471594714631548, -0.6704579022356528, -0.7090564063186768, -0.7584053880552923, -0.8101244036157627, -0.8526189235085075, -0.872417498261418, -0.8561767863823757, -0.7930533916017833, -0.6770604606987946, -0.5089375701527854, -0.2971550620890392, -0.05761269204799846, 0.18789151496970918, 0.4143336303799478, 0.596919125262307, 0.7147087986695557, 0.7538529097411865, 0.7097353627437273, 0.5877778836770051, 0.40257278286196346, 0.1755748921605498, -0.06817834720063913, -0.30381917292160493, -0.5101473732591594, -0.6722715103438465, -0.782942771822579, -0.8426075541528982, -0.8581499860345086, -0.8406550377330191, -0.8028915815603971, -0.7569445207502417, -0.7124441110679234, -0.6756211416707443, -0.6492985792878058, -0.6336104831921037, -0.6270868628284776, -0.6278993868440812, -0.6347460148648578, -0.6473189374357599, -0.6660652122000107, -0.6914774106844375, -0.7231297220029862, -0.7587664029448702, -0.7936544758660282, -0.8205522923344901, -0.8305429506490288, -0.8142884856193261, -0.7636823212203829, -0.673529581873597, -0.5429181777841331, -0.3758793938755062, -0.18113858110834186, 0.028812354472331908, 0.23939310934756888, 0.4359274511900307, 0.6056519046787863, 0.7393627898718214, 0.8324327306148087, 0.8851319247653551, 0.9020886016493107, 0.8911142062914292, 0.8617307665544903, 0.8235701121823792, 0.7850172209229723, 0.7522557788351737, 0.7288635601528786, 0.7158958847588804, 0.7123277223581522, 0.715761845721655, 0.7231900323302534, 0.7316880970831603, 0.7389528359720056, 0.7435736461024193, 0.7451046063677472, 0.743901281226759, 0.740788821822152, 0.7367782401995692, 0.7328033193551644, 0.7294981194191762, 0.7271513904156902, 0.7257726558576425, 0.725159941446078, 0.725060989178965, 0.7252632377419967, 0.7256163395829798, 0.7260606904500417, 0.7265379023034586, 0.7270291732601397, 0.7275033865931528, 0.7279199682707127, 0.7282769079854728, 0.7285974590770533, 0.7289407767207793, 0.7293428506461535, 0.7298479408102396, 0.7304778513692572, 0.7311828384458046, 0.7318265401385785, 0.7323028750384627, 0.7325567749966301, 0.7325033028493253, 0.7321158823152807, 0.7314068004824351, 0.7304533892028899, 0.7293390182016347, 0.7281572743585262, 0.7270606197087242, 0.7261241067000211, 0.7253508195631971, 0.7246697616263047, 0.723969429286671, 0.723139564739256, 0.7220976758138733, 0.7208555865072881, 0.719568292828321, 0.7184478733558384, 0.7176993275862744, 0.7174622207349447, 0.7177521937986072, 0.718516228428159, 0.7195981106474233, 0.7207879819353863, 0.7218924194293399, 0.7227111613943498, 0.7231168859595661, 0.7230786498664554, 0.7226411424851807, 0.7219463720454906, 0.7211811690986409, 0.7204810710907097, 0.7199538718599565, 0.7196320372423504, 0.7194607411817737, 0.7193099127963588, 0.7190971249818399, 0.7188635612803779, 0.7188051788075457, 0.7192369464355841, 0.7205351477714964, 0.7229401499987833, 0.7263486481418566, 0.7301617369824043, 0.7333271712095472, 0.7344308070476105, 0.7320183145085448, 0.7250816880667706, 0.7135657369657201, 0.6987104127947069, 0.6831567860992641, 0.6708043964638186, 0.6662258399732381, 0.6737496016563864, 0.6962181897094762, 0.7338123953236427, 0.7831464621140352, 0.8367458472751513, 0.8833813981307604, 0.9091987678800104, 0.8998091259693833, 0.8428401153753142, 0.7305998791526044, 0.562507495226734, 0.34659814194077, 0.0995702257773744, -0.15462281131582128, -0.3875977492359962, -0.5706271624637833, -0.6790839949047796, -0.6967382767827438, -0.6189803271815245, -0.4544562375583789, -0.22459908414379984, 0.03903553601854455, 0.29916696405087967, 0.5182679460830586, 0.6643639077354586, 0.7159339540668409, 0.6652943920234429, 0.5198749673865217, 0.300993470244488, 0.04051717061424443, -0.22409581460784916, -0.45544556602126973, -0.6216785191074483, -0.7008762468325049, -0.6837610820977862, -0.5742886326760264, -0.3883111156265534, -0.1505286326662823, 0.10967239939698414, 0.3627475020866999, 0.5831487815378037, 0.7525668303202456, 0.8617987081334637, 0.9111768991603971, 0.9094611758407977, 0.8715862070139058, 0.8157455416667302, 0.760202018310825, 0.7202658930923688, 0.7058888207208955, 0.7201847936946834, 0.759052366114439, 0.811812333812609, 0.8630070563777121, 0.8948697888398245, 0.8903643946442023, 0.8361831300618912, 0.7252589385855543, 0.5584821670091451, 0.345315670477598, 0.10299763765352206, -0.14547539122840722, -0.37428698339337824, -0.5583637418127292, -0.6768312337753024, -0.7159704258460882, -0.6711625159308375, -0.5476542552431498, -0.3597709705436185, -0.1287724532856077, 0.12018518168690656, 0.36151984386717273, 0.572699142103299, 0.7370284868429373, 0.8455964386542135, 0.8979126579643226, 0.9012807607635166, 0.8690744380604796, 0.8181990426007191, 0.7661088030574076, 0.7279245613823432, 0.7140037167311404, 0.7282038712248695, 0.7671972819282604, 0.8208631561250372, 0.8738564756136162, 0.9080475656744531, 0.9055112204914009, 0.8518434216042863, 0.7389767670280546, 0.5673122043840576, 0.346672036977057, 0.09563946895916749, -0.1604955961723308, -0.3929887785452873, -0.573731438794397, -0.6795623772004052, -0.6960013467696725, -0.619916032405668, -0.46047605211853976, -0.238293779549608, 0.017302276506560462, 0.2723050965454336, 0.4928472153853533, 0.6499682346772773, 0.7235856630223708, 0.7050531042870595, 0.5980296925245243, 0.4173625434472803, 0.18635581949974522, -0.06697296685650257, -0.3141616680583659, -0.5303108718258116, -0.6972846806923089, -0.805693295562243, -0.8554610680619644, -0.8548810350527455, -0.8184903429533198, -0.7641725094683359, -0.7100008771843999, -0.671228658984871, -0.657884155216942, -0.6731679025330721, -0.7131015741595147, -0.7671687462263975, -0.8200654189127506, -0.8542004537564716, -0.8526249939936517, -0.8019646550151107, -0.6949224336608516, -0.5320250473508275, -0.32225185034324333, -0.08237582607009868, 0.1650026835738332, 0.39428466394542017, 0.5803342409591474, 0.7020686940954762, 0.7453870445521058, 0.7052505477960299, 0.5864589514160631, 0.40293010537214813, 0.17562748086081167, -0.0704552502607787, -0.309822690701368, -0.5200321703524325, -0.6844918028247094, -0.7944039739927944, -0.849369247148433, -0.856656043797114, -0.8292787623167311, -0.7833804658452638, -0.7353387812407823, -0.6989933350482087, -0.6835224068604273, -0.6921158238785066, -0.7217188264252835, -0.7637517506720419, -0.8057159017858148, -0.8333093620537693, -0.8327870038627241, -0.7931510688939891, -0.7079388773369498, -0.5762895149017982, -0.4032287101039275, -0.19912345762738048, 0.021626092972811716, 0.24243838454530214, 0.4466281803126936, 0.6195670275196116, 0.7505384293302241, 0.8341667424696944, 0.8710515511074273, 0.867618588313726, 0.8350546605288388, 0.7875968290108912, 0.7403153596554869, 0.7065887377614032, 0.6958348088594112, 0.7117510991794384, 0.7514265747295997, 0.8055501080993405, 0.8597172027233948, 0.896672112950365, 0.8992716440220376, 0.8535956532880161, 0.7516973279064126, 0.5935739768219647, 0.3879409425761628, 0.1514795080598367, -0.09323685375808283, -0.32079142716179476, -0.5065138588773618, -0.6300491223171335, -0.6781015202421304, -0.64619431762589, -0.5389832779795898, -0.36913308344851997, -0.15510153259215717, 0.08166236993095077, 0.3196509591252603, 0.5398927777919778, 0.7276930986154884, 0.8734985979773947, 0.9728047077610658, 1.0252642302363124, 1.0333899494712895, 1.0012329554745556, 0.9333027118497857, 0.8339401572384909, 0.7072095654921254, 0.5571462896311223, 0.3881483450425459, 0.20534155782487487, 0.01482887737245796, -0.1764521290488, -0.3611157500299354, -0.5318043493520626, -0.6818066642899347, -0.8054524101831724, -0.8983255342414102, -0.9572814410830893, -0.9802961943453828, -0.9661962276209902, -0.9145882909024544, -0.8259958203690237, -0.702124108056222, -0.5463111553516156, -0.3640099142702318, -0.1630068815984123, 0.04665386649189137, 0.25324056756651203, 0.4443960991039263, 0.6085609531447825, 0.7365289833752492, 0.8228996922007434, 0.8670933837874918, 0.8736111453366721, 0.8515289789816484, 0.8132403002190881, 0.772465080941647, 0.7419679771548864, 0.7313371097907961, 0.7450271466496866, 0.7811915546642222, 0.8315498322037654, 0.8823689588265033, 0.9165305921773814, 0.9163401501954511, 0.866798433796903, 0.7586596196292686, 0.5908492722170399, 0.37178062020046765, 0.11907890680745346, -0.14211821683680798, -0.38238233257874527, -0.5721392733995939, -0.6862057323913836, -0.7079902911617727, -0.6327143381258475, -0.4689575875843263, -0.23816585088733142, 0.02788728184520496, 0.2913733998865506, 0.5138745348418566, 0.6622161891528019, 0.713630396728027, 0.6595409016687056, 0.5072353110800646, 0.2790535214186103, 0.009173689804918802, -0.26151320666451255, -0.49168518087347146, -0.646028784822539, -0.7007240447824197, -0.6471884427151815, -0.493530539618674, -0.2632018631271933, 0.008643095196815533, 0.28067049342689865, 0.5117662020698565, 0.667360375596674, 0.7246614220304907, 0.6758948089830248, 0.5292499968474088, 0.30723953882700833, 0.04292589220225078, -0.22522884697938184, -0.4592044373314265, -0.6269083921942394, -0.7064584618733396, -0.6888404338934664, -0.578411648288706, -0.39139022626549447, -0.15271914914807735, 0.10811456934185323, 0.36154443524920665, 0.5821113615057549, 0.7515472341269214, 0.8606474547165524, 0.9096953707888916, 0.9073268916916939, 0.8684122594374747, 0.8110629523849187, 0.7535131577918508, 0.7111116174600383, 0.6939391865838809, 0.7053500144234236, 0.7415364458091326, 0.7922663020024436, 0.8425535702269459, 0.8751141872059586, 0.8732034679792344, 0.8235993150699542, 0.7190183727683939, 0.5598342988350936, 0.3547305255173707, 0.12000835651727722, -0.12227364288086777, -0.34712620885755746, -0.5299758484536152, -0.6500817333967435, -0.6934598211856411, -0.6548680069310724, -0.538631179832801, -0.35797405653961106, -0.13314154269390344, 0.11150249461783546, 0.3507932103438662, 0.5622006640712187, 0.7287398470888085, 0.8409123226340982, 0.8975410491756267, 0.9052474392037568, 0.8767801125750505, 0.8285828512227308, 0.7778392815717208, 0.7394654445105879, 0.7237013633767214, 0.7343864257619723, 0.7683602106205176, 0.8160146443370595, 0.862832671453382, 0.8918135732392275, 0.8863825849799384, 0.8334021521345413, 0.7256529739097736, 0.5635985512953553, 0.35608386653185525, 0.1195604135723027, -0.12374840459859741, -0.3487502236997944, -0.5308687349642771, -0.6495113130900928, -0.6909901985488635, -0.6504937240912037, -0.5328353201969774, -0.3517349807169625, -0.12783984379196844, 0.11423012543166067, 0.3492730631198282, 0.5549865684462535, 0.7147604584382636, 0.8196924285734603, 0.8692925730239803, 0.8708584840188425, 0.8377913064207088, 0.7870129074549828, 0.7359765930553231, 0.6996793525556969, 0.6881560723752628, 0.7048218776482567, 0.7458257319106636, 0.8006775631265496, 0.853917719961837, 0.8877440401214893, 0.8850693181898429, 0.8326613733709883, 0.7236976539802175, 0.5594490106415803, 0.3497538967519691, 0.11201578047048573, -0.13100695912350224, -0.3542636347146736, -0.5338912711941378, -0.6506028489493497, -0.6922424302133595, -0.6552909494544218, -0.545064832644278, -0.37448254797377645, -0.16191455440330382, 0.07162348789175096, 0.305307696187205, 0.5209397804835978, 0.7045483839307563, 0.8471495500869136, 0.9446334649114675, 0.9967359029755237, 1.0058177131022314, 0.9755714551521117, 0.910087443335543, 0.8133163625595331, 0.6890103411064745, 0.5410140712172831, 0.37367966894661164, 0.19222351735516607, 0.002885008671315868, -0.18723164421141011, -0.3706358231842831, -0.540017664941237, -0.6887965775506286, -0.811456181705438, -0.9037768968384509, -0.9627749707154154, -0.986428591882344, -0.9734798839005043, -0.9233425758887451, -0.8362626385273748, -0.7136342940914308, -0.5585921807071323, -0.37653877807456615, -0.17539608244694269, 0.03449829302119377, 0.24108409799518699, 0.4317114568156308, 0.5946337468390553, 0.7205719868506776, 0.8042233087437884, 0.8452649724027359, 0.8485537347599877, 0.8236121116636361, 0.7832470748996688, 0.7415340851598169, 0.7114139852567443, 0.7023916754066073, 0.7186444625002776, 0.7579146977658392, 0.8114788518364714, 0.865212362785649, 0.9017186145139675, 0.9031789704236397, 0.8546836474975438, 0.7473081616445082, 0.5805118731598218, 0.3633604703375262, 0.11403099657073672, -0.1421571689009856, -0.376100265224383, -0.5591208341865042, -0.66748156416295, -0.6863264429683489, -0.61238919788703, -0.45495950013783854, -0.2348765682622349, 0.018329318180048494, 0.27072256893627067, 0.4888669989484364, 0.6445441082266234, 0.7186091906642366, 0.7032516717681991, 0.602286440359839, 0.4297305321288512, 0.20693427048046936, -0.04118448970582595, -0.2899486028515708, -0.51813884111226, -0.7100679145508004, -0.8564812364022516, -0.954078154354838, -1.004051301932304, -1.0102212014763818, -0.9772535580383042, -0.9093646718646989, -0.8097976595431309, -0.6810878313976068, -0.5258335391357575, -0.34780340225624445, -0.15283789222057037, 0.05073422541995442, 0.25233190333965977, 0.44007238959276546, 0.6022906295601135, 0.7293932651728482, 0.8155001380288734, 0.8596440510683021, 0.8661244160018878, 0.8440053760191001, 0.8057116144877121, 0.7648934322393982, 0.7341019522530025, 0.722408788035578, 0.7335846743805764, 0.76523665163658, 0.8088069415554398, 0.8508057382972929, 0.8750784439185956, 0.8656525197192184, 0.8097364952043214, 0.7004331018480651, 0.5385134797346247, 0.333020638982082, 0.10055243220663874, -0.13684916712333142, -0.3547046170347631, -0.5296187059445376, -0.6427036804094352, -0.6822150791593455, -0.6450059416608724, -0.5366580259087476, -0.37013892662339776, -0.16344566761793425, 0.06325834047144631, 0.29051687792880865, 0.5019090102948002, 0.685337537979504, 0.8332571783100664, 0.9419059935710599, 1.0099338897337269, 1.0368536824281052, 1.0219112826998396, 0.9637216757298569, 0.8608644035958495, 0.7132682495621445, 0.5240958995354725, 0.30150783203128084, 0.05962244367312289, -0.18169903701790627, -0.3985650165893692, -0.5660874768283738, -0.6622779885806316, -0.6721281174161831, -0.5910217986061128, -0.4267122427659796, -0.19931344093386746, 0.06087906417721856, 0.31748163584889194, 0.5333437531858058, 0.6763479522156483, 0.7245443113283739, 0.6697558890344962, 0.5190710655465737, 0.2937181748767438, 0.02576020244976748, -0.24681249668741956, -0.4858948596428177, -0.6588635605451997, -0.7431160183824671, -0.7289134552508003, -0.6200694296515479, -0.4325067812603366, -0.19121024572221312, 0.07400166309693594, 0.3330849816678037, 0.5599873834891823, 0.7359349670621476, 0.8513661111199331, 0.9063246869034065, 0.9094064046484032, 0.8755054075051303, 0.8228032542069148, 0.7695512733800192, 0.7310864566365781, 0.7174344380700259, 0.7318771929311987, 0.770521492507058, 0.8229990169861556, 0.8741669857800006, 0.9065945000702298, 0.9034290410951017, 0.8513488075060012, 0.7431105593701001, 0.5792771762670239, 0.3688585907869233, 0.12855873457058717, -0.11905374155741394, -0.348465451110149, -0.5346000660767498, -0.6563026294503328, -0.6993804544754962, -0.6586232637177873, -0.5386587210945445, -0.35325412329016936, -0.12340944757935825, 0.12562838916868907, 0.3678984527083349, 0.5802535686096911, 0.7453566040596344, 0.8536797217461267, 0.904341743696613, 0.9045288934223483, 0.8678005605218305, 0.8115232656672823, 0.7538338251356304, 0.7106289265654393, 0.6929469282521439, 0.7051665302164144, 0.7441987520198292, 0.7999632255413621, 0.8568697593576841, 0.8963183241181077, 0.8998019936252488, 0.8522424023181564, 0.7449696798222867, 0.5778551163588856, 0.3603125530553699, 0.11070054945898282, -0.14570230635299203, -0.3799809948767624, -0.5637043781173343, -0.6732548027150764, -0.693664788209523, -0.6213306289901542, -0.46505052769065697, -0.24516543111583403, 0.0090596915946915, 0.2635428251223252, 0.48417637041829653, 0.641689526437302, 0.7157173189250563, 0.6973828411174359, 0.5901314098610099, 0.4086428546496129, 0.17619718572689294, -0.07917988137166046, -0.328937783780878, -0.5480728892646238, -0.7183409139718169, -0.830216292312652, -0.8834929518448947, -0.8862829283786646, -0.8529835994516479, -0.8013536812216641, -0.7493136237212195, -0.711957955660661, -0.6991338441055578, -0.7139427031909754, -0.7523268372875261, -0.8037761996631599, -0.8530893578229929, -0.8828792296977179, -0.8764987725251604, -0.8209490836280732, -0.7093747657586275, -0.5427215391631399, -0.33033331822457584, -0.08916763854378294, 0.15803966171501063, 0.3856904000524847, 0.5687642313471672, 0.6864040238926279, 0.724868684652829, 0.6795420414253549, 0.5557211678730963, 0.3677696222282419, 0.13706564016321376, -0.11113892216576668, -0.3513165038596046, -0.5611655218564168]}] caption="Constellation Graph"
  out "Sync Found 2":bool=TRUE
  out "Correct Packets Rx 2":i16=46
  out "Singal & Noise Power 2":cluster{"signal_power":dbl, "noise_power":dbl}={"signal_power"=0.000719802679436105, "noise_power"=8.71918670194843e-09}
  out "error out 3":errorcluster
  out "Cumulative Packets Recovered 2":i16(graph)=46
  out "Signal and Noise Power Tracking 2":cluster{"total_power":dbl, "noise_power":dbl}(graph)={"total_power"=0.000719802679436105, "noise_power"=8.71918670194843e-09}
  out "x .or. y? 4":bool
  in  "synchronization parameters 3":T1={"expected sync location (symbols)"=-1, "sync sequence"=[], "sync location uncertainty (symbols)"=0, "sync indent (symbols)"=0} caption="synchronization parameters" {"sync sequence" format="%.2f"}
  in  "Tab Control 6":T2(tab)=enum."Rx Display"
  in  "Acquisition Duration [sec] 3":dbl=0.04 format="%#.6p"
  in  "Rx Parameters 3":T3={"Rx IQ Sampling\nRate [s/sec]"=500000.0, "Rx\nFrequency [Hz]"=915000000.0, "Rx Gain [dB]"=20.0, "Rx Antenna"="RX1"} {"Rx Gain [dB]" format="%#.6p"; "Rx\nFrequency [Hz]" format="%#.6p"; "Rx IQ Sampling\nRate [s/sec]" format="%#.6p"}
  out "Actual Rx Parameters  3":T3={"Rx IQ Sampling\nRate [s/sec]"=500000.0, "Rx\nFrequency [Hz]"=915000000.0, "Rx Gain [dB]"=20.0, "Rx Antenna"="RX1"} {"Rx Gain [dB]" format="%#.6p"; "Rx\nFrequency [Hz]" format="%#.6p"; "Rx IQ Sampling\nRate [s/sec]" format="%#.6p"}
  out "Symbol Rate\n[symbols/sec] 6":dbl=62500.0 format="%#.6p"
  in  "Choose a PSK Format 3":T4(tab)=enum."QPSK" caption="PSK"
  in  "BPSK System Parameters 6":T5={"Samples per Symbol"=8, "symbol map"=[], "Differential PSK"=enum."disable", "PSK type"=0} caption="BPSK System Parameters" {"PSK type" items=["normal", "shifted", "offset"]; "symbol map" format="%.3f"}
  in  "QPSK System Parameters 6":T5={"Samples per Symbol"=8, "symbol map"=[], "Differential PSK"=enum."disable", "PSK type"=0} caption="QPSK System Parameters" {"PSK type" items=["normal", "shifted", "offset"]; "symbol map" format="%.3f"}
  in  "pi/4 DQPSK System Parameters 6":T5={"Samples per Symbol"=8, "symbol map"=[], "Differential PSK"=enum."enable", "PSK type"=1} caption="pi/4 DQPSK System Parameters" {"PSK type" items=["normal", "shifted", "offset"]; "symbol map" format="%.3f"}
  in  "OQPSK System Parameters 6":T5={"Samples per Symbol"=8, "symbol map"=[], "Differential PSK"=enum."disable", "PSK type"=2} caption="OQPSK System Parameters" {"PSK type" items=["normal", "shifted", "offset"]; "symbol map" format="%.3f"}
  in  "8-PSK System Parameters 6":T5={"Samples per Symbol"=8, "symbol map"=[], "Differential PSK"=enum."disable", "PSK type"=0} caption="8-PSK System Parameters" {"PSK type" items=["normal", "shifted", "offset"]; "symbol map" format="%.3f"}
  in  "16-PSK System Parameters 6":T5={"Samples per Symbol"=8, "symbol map"=[], "Differential PSK"=enum."disable", "PSK type"=0} caption="16-PSK System Parameters" {"PSK type" items=["normal", "shifted", "offset"]; "symbol map" format="%.3f"}
  in  "M 6":i32=4 caption="M" min=2 step=2
  in  "Custom System Parameters 6":T5={"Samples per Symbol"=8, "symbol map"=[], "Differential PSK"=enum."disable", "PSK type"=0} caption="Custom System Parameters" {"PSK type" items=["normal", "shifted", "offset"]; "symbol map" format="%.3f"}
  in  "filter parameters 3":T6={"Alpha"=0.5, "Filter Length"=6, "TX Filter"=enum."Root Raised Cos"} caption="Matching Filter Parameters" {"Alpha" format="%.2f"}
  in  "PN Sequence Order\nfor Sync 3":i32=31
  in  "Packet Parameters 6":T7={"Guard Bits "=30, "Sync Bits"=20, "Message Bits"=128, "Number of Packets \nto Expect"=46}
  out "Recovered Message 3":string="Two roads diverged in a yellow wood,\nAnd sorry I could not travel both\nAnd be one traveler, long I stood\nAnd looked down one as far as I could\nTo where it bent in the undergrowth.\n\nThen took the other, as just as fair,\nAnd having perhaps the better claim,\nBecause it was grassy and wanted wear;\nThough as for that the passing there\nHad worn them really about the same.\n\nAnd both that morning equally lay\nIn leaves no step had trodden black.\nOh, I kept the first for another day!\nYet knowing how way leads on to way,\nI doubted if I should ever come back.\n\nI shall be telling this with a sigh\nSomewhere..."
  out "Received Signal (Raw) 3":dbl[](graph)
  out "Constellation Graph 6":T8(graph)=[{"Decimated Array"=[-0.6804993103727607, -0.6771092058245918, -0.6428257187708691, 0.7259219405542873, 0.7311366832454209, -0.6450362325295403, -0.658892442379921, -0.6855840493085356, -0.646998431742077, -0.6568678904388265, 0.7432214399633668, -0.6618522924674632, -0.6753922285302938, 0.6950905811428861, 0.7248141384495557, 0.7218255862492685, 0.704818637196686, 0.7027336696732543, 0.7016253671990413, 0.7082534735709545, 0.7084209330001522, 0.7036372125301554, 0.7010930640613204, 0.7075984577478206, 0.7100058187983528, 0.7171431626733421, 0.7279231861183771, 0.6959557947635676, -0.7024336186443912, -0.7110189818905128, 0.6934234462727887, 0.7327126116070742, 0.7051667045224878, 0.690798979580973, -0.6877839781333666, 0.6889445287579181, 0.716354235720989, -0.706071092371314, 0.72195318833854, -0.7119212984185137, 0.7223509528651848, -0.7244956435522718, -0.6716656585292338, -0.7182056308592257, 0.724421589775866, -0.6763390206227603, 0.7587597202334532, -0.6966306246608392, -0.6999692828092537, -0.7056805503027465, 0.7430994824068496, 0.7108305621069824, 0.7197425435843314, -0.7051937005816177, -0.6734048186040171, -0.6909214820858487, 0.7004218263991402, -0.6889802592692622, 0.7244882842042791, 0.7027757047403482, -0.7012448562483489, -0.6963431828766949, 0.7166197717755273, 0.7431431506248717, 0.7233235134334371, 0.6983161172439467, 0.7059749857271942, -0.6872358926309042, 0.6918268533027474, -0.7138701729016586, -0.6801285945135653, 0.7195044185357663, 0.6810587309328351, -0.6856313040037053, -0.7011043347997452, 0.6920652628903768, -0.7080955978852922, -0.6860253207439192, -0.7101309321759165, 0.7212965033681705, 0.6967245108747491, 0.7128097205123256, 0.6657328144726218, 0.6985573048815797, 0.6967609587320983, 0.720489591403177, -0.6992149062771553, 0.6810319795543738, -0.7124274384065621, -0.6689704942642202, 0.7017697482270308, 0.7036983705130238, -0.69378287602043, -0.6926507402482928, 0.6832891050414109, 0.7219614630178657, 0.7044242088089868, 0.6722056874933439, -0.6818156450864503, 0.6786113633855301, 0.7039257931121476, -0.6836867328922335, 0.6967676536286352, -0.7018627722542645, 0.7033449800412358, -0.7121625353086042], "Decimated Array"=[0.7327573786203745, 0.7417811878517194, -0.6799031648608087, -0.7111421642681004, -0.727382953469249, -0.6704579022356528, -0.6770604606987946, 0.7538529097411865, -0.6722715103438465, -0.6756211416707443, -0.6914774106844375, -0.673529581873597, 0.7393627898718214, 0.7522557788351737, 0.7435736461024193, 0.7257726558576425, 0.7275033865931528, 0.7311828384458046, 0.7293390182016347, 0.7220976758138733, 0.7195981106474233, 0.7211811690986409, 0.7188051788075457, 0.7320183145085448, 0.6962181897094762, 0.7305998791526044, -0.6967382767827438, 0.7159339540668409, -0.7008762468325049, 0.7525668303202456, 0.7058888207208955, 0.7252589385855543, -0.7159704258460882, 0.7370284868429373, 0.7140037167311404, 0.7389767670280546, -0.6960013467696725, 0.7235856630223708, -0.6972846806923089, -0.657884155216942, -0.6949224336608516, 0.7453870445521058, -0.6844918028247094, -0.6835224068604273, -0.7079388773369498, 0.7505384293302241, 0.6958348088594112, 0.7516973279064126, -0.6781015202421304, 0.7276930986154884, 0.7072095654921254, -0.6818066642899347, -0.702124108056222, 0.7365289833752492, 0.7313371097907961, 0.7586596196292686, -0.7079902911617727, 0.713630396728027, -0.7007240447824197, 0.7246614220304907, -0.7064584618733396, 0.7515472341269214, 0.6939391865838809, 0.7190183727683939, -0.6934598211856411, 0.7287398470888085, 0.7237013633767214, 0.7256529739097736, -0.6909901985488635, 0.7147604584382636, 0.6881560723752628, 0.7236976539802175, -0.6922424302133595, 0.7045483839307563, 0.6890103411064745, -0.6887965775506286, -0.7136342940914308, 0.7205719868506776, 0.7023916754066073, 0.7473081616445082, -0.6863264429683489, 0.7186091906642366, -0.7100679145508004, -0.6810878313976068, 0.7293932651728482, 0.722408788035578, 0.7004331018480651, -0.6822150791593455, 0.685337537979504, 0.7132682495621445, -0.6721281174161831, 0.7245443113283739, -0.7431160183824671, 0.7359349670621476, 0.7174344380700259, 0.7431105593701001, -0.6993804544754962, 0.7453566040596344, 0.6929469282521439, 0.7449696798222867, -0.693664788209523, 0.7157173189250563, -0.7183409139718169, -0.6991338441055578, -0.7093747657586275, 0.724868684652829]}, {"Decimated Array"=[-0.6804993103727607, -0.6762349965387238, -0.6685108157798112, -0.6587623289821404, -0.6494739544100483, -0.6438465750011458, -0.645155862498135, -0.6559333949667008, -0.6771092058245918, -0.707329395010057, -0.7427108893571827, -0.7768816274525345, -0.8016064503455926, -0.8078913118575249, -0.7873020181422804, -0.7333876332701184, -0.6428257187708691, -0.5161117575568228, -0.35777203758853365, -0.17570329650700167, 0.01987541369217473, 0.21778298257008183, 0.4072432109758152, 0.5789865397268567, 0.7259219405542873, 0.8433225109633283, 0.9285347773827741, 0.9803625623365572, 0.9983411710644498, 0.9823024312079763, 0.9321501534368272, 0.8480801425231922, 0.7311366832454209, 0.5839247754585907, 0.41126876723240074, 0.2204206478178329, 0.020932943403138903, -0.1761332529377578, -0.3593512576776315, -0.5183227318987554, -0.6450362325295403, -0.7348944300155227, -0.7873580245691122, -0.8057437870339258, -0.7965717988687436, -0.7684407927742708, -0.7306238606226202, -0.6917860656058442, -0.658892442379921, -0.6364690666334113, -0.6263656338128196, -0.6279033391241801, -0.6383295002999582, -0.6535857140497858, -0.6691389263327601, -0.6808303682804338, -0.6855840493085356, -0.6819546232796994, -0.6704727894453094, -0.6535744314745204, -0.6353365462635079, -0.6208696353048802, -0.6154307523642993, -0.6233724286798671, -0.646998431742077, -0.6855864576394015, -0.7347128803667217, -0.7860882541221362, -0.8282453730286534, -0.8479309126781169, -0.8321007406466316, -0.7702787309009056, -0.6568678904388265, -0.4928870454737699, -0.286812316855307, -0.054181947000257816, 0.18398541460571163, 0.403912791430555, 0.5822957160369652, 0.6996654194867074, 0.7432214399633668, 0.7085518372290116, 0.6001271112229511, 0.43028071322686884, 0.21712133759522834, -0.01828477060583316, -0.25486167705907176, -0.474106655260725, -0.6618522924674632, -0.8090041994597156, -0.9113555181844136, -0.9685514235160106, -0.9827395175415803, -0.9572113882143858, -0.8953875269303032, -0.8004356628744611, -0.6753922285302938, -0.5237515103490776, -0.3502005293644506, -0.1611351791820148, 0.03517140208780353, 0.22893110044459927, 0.40972263321669966, 0.5677345648283395, 0.6950905811428861, 0.7869683371034619, 0.8423038906676682, 0.8638849324516561, 0.8577538092414735, 0.8321468933549871, 0.7961070317612736, 0.7580880124868856, 0.7248141384495557, 0.7005277134039959, 0.686923334338586, 0.6833877232132058, 0.6876280888811944, 0.6964899036822818, 0.706747954834772, 0.7157647696850384, 0.7218255862492685, 0.724268969267967, 0.7234261321898535, 0.7202619630220548, 0.7159731242866095, 0.7116890979547664, 0.7082240869885714, 0.70594341514383, 0.704818637196686, 0.7045271958113069, 0.7047088927454438, 0.7050023859293303, 0.7051255773761397, 0.7049541452505861, 0.7044514570052206, 0.7036747950662702, 0.7027336696732543, 0.7017628701423971, 0.7009138948889888, 0.7003118882562483, 0.7000261021126073, 0.7000875017890581, 0.7004449481097869, 0.7009932809698078, 0.7016253671990413, 0.702221540251104, 0.7027618684813808, 0.7032916906181711, 0.7038854962099375, 0.7046487256800136, 0.7056308879137863, 0.7068515417419651, 0.7082534735709545, 0.7096888191782372, 0.7109913402244956, 0.7119894724643936, 0.7124890080936077, 0.7123827414517839, 0.7116323891766451, 0.7102633952930952, 0.7084209330001522, 0.7063057748688335, 0.7042562032788021, 0.7025954190884202, 0.7015546954049546, 0.7012557549487087, 0.7016448259380934, 0.7025398218482226, 0.7036372125301554, 0.7046321819639692, 0.7053295412842902, 0.7055972799037947, 0.705357986716468, 0.7046523984817116, 0.7036068751653552, 0.7023536981462808, 0.7010930640613204, 0.7000326295845363, 0.6993965049981011, 0.6993226127993213, 0.6998881120919372, 0.701113074412268, 0.7029138523453567, 0.7051416575412044, 0.7075984577478206, 0.710078980444559, 0.7123321038850414, 0.7140736603763724, 0.7150314533562983, 0.7150214932752349, 0.7140093308210059, 0.7121877418723002, 0.7100058187983528, 0.70805206355385, 0.7070027727419878, 0.7073212689161522, 0.7091056294101988, 0.7119833987327618, 0.7150644848824459, 0.7171668570713718, 0.7171431626733421, 0.71423133689185, 0.7085192919358748, 0.7011650150275229, 0.6943243914091253, 0.6909299894216554, 0.694045612210552, 0.706066960259486, 0.7279231861183771, 0.7583890909767882, 0.7938021658029275, 0.8279962238841705, 0.8528896550258644, 0.8595701988778817, 0.8395633321459017, 0.7862278633870129, 0.6959557947635676, 0.5689496495122442, 0.4094105630569515, 0.22502717825358973, 0.025894312218078558, -0.17672464042078925, -0.37176542586543576, -0.5495413422869474, -0.7024336186443912, -0.8251771287794907, -0.9146738107129905, -0.9693864660264264, -0.9886486884020281, -0.9721997012143947, -0.920010882437784, -0.8324905468768208, -0.7110189818905128, -0.5586215402038113, -0.38057133580870495, -0.18461757845785642, 0.019294891934465676, 0.2197963582992338, 0.4053691867674974, 0.5657713716359056, 0.6934234462727887, 0.7843501298361789, 0.8386729718179944, 0.8602628823550353, 0.855774513907276, 0.8333154686311419, 0.8010170366525857, 0.7658225991667146, 0.7327126116070742, 0.7045406905991981, 0.6824916000019303, 0.6667964864918056, 0.6575588911889615, 0.6553991485314229, 0.6616300661715835, 0.677865934701111, 0.7051667045224878, 0.7429233296416752, 0.7878677137961015, 0.8333853282559609, 0.8696348770191419, 0.8846190114381185, 0.8659756375138661, 0.8033400824826783, 0.690798979580973, 0.5288571353054295, 0.32551133007737276, 0.09595098720473762, -0.13906888290440567, -0.35588344294942403, -0.5312979803398246, -0.646084108275294, -0.6877839781333666, -0.6524636145322816, -0.5450893812430798, -0.37828756856953233, -0.17009276356333847, 0.0590247558982818, 0.28912715162217667, 0.5032762839933951, 0.6889445287579181, 0.8383428746399739, 0.9477025130341128, 1.015790170453614, 1.0423483901645878, 1.0268512388275022, 0.9680879161655901, 0.8646551393981081, 0.716354235720989, 0.5260764152807655, 0.30160439840294034, 0.05668512406955431, -0.18910351581760784, -0.4118751751084471, -0.5863423085037114, -0.6897554505434935, -0.706071092371314, -0.6295185621493208, -0.4668637151478481, -0.23765972556227086, 0.027714817455610417, 0.29202447870753795, 0.5167154122972588, 0.6679084709283569, 0.72195318833854, 0.6695114009171929, 0.5175155629675429, 0.2883041299697019, 0.01623720013151288, -0.25755900242514196, -0.4917082138253101, -0.6510176327160702, -0.7119212984185137, -0.6659995880876536, -0.5209852917537516, -0.2992839322286186, -0.03416997277404838, 0.2355466281568285, 0.4714352113659737, 0.6410442893752866, 0.7223509528651848, 0.7062991907811851, 0.5973003486423586, 0.4116890808688979, 0.17445466790696096, -0.08489625696410336, -0.3368901331962952, -0.5561324114364461, -0.7244956435522718, -0.832904063982776, -0.8817003370505312, -0.8795283892255058, -0.841156501109088, -0.7846263716950196, -0.7281214416972949, -0.6870445779683771, -0.6716656585292338, -0.6855631019709484, -0.7251869491105687, -0.7803544807713914, -0.8357414937022205, -0.8732615963603204, -0.8749681769421048, -0.8261602248386887, -0.7182056308592257, -0.5506938062457699, -0.3325933377055765, -0.08189760414583691, 0.17618237159000388, 0.4123697444728759, 0.5974694739328056, 0.7068084628379865, 0.724421589775866, 0.6461724854013321, 0.4812775786848407, 0.25159361606242997, -0.011058078343011023, -0.2692923486046545, -0.48569025029571594, -0.6284581525739953, -0.6763390206227603, -0.6219818356022658, -0.47306441806801147, -0.2510857990405568, 0.01202477775150253, 0.27875734553572085, 0.5116930035471384, 0.6789865139576629, 0.7587597202334532, 0.7418192787585248, 0.6323458533022597, 0.446406792743502, 0.20878035238051276, -0.05119783320575381, -0.3042611875270661, -0.5253152667965498, -0.6966306246608392, -0.8095606744479041, -0.8647740627418172, -0.870930075780708, -0.8423384959975685, -0.7960318277718325, -0.7486596019303445, -0.7137982795070836, -0.6999692828092537, -0.7095971091381883, -0.7390816485119921, -0.7796138336185289, -0.818762813999536, -0.8425904879324037, -0.8378822227707572, -0.7942341058424417, -0.7056805503027465, -0.571726769560303, -0.39765177441111643, -0.19391837432237818, 0.025178720377377686, 0.24333379676657457, 0.44433965307888695, 0.6142375047967751, 0.7430994824068496, 0.8263038750024307, 0.8650100488333368, 0.8657148042767202, 0.8390794723757462, 0.7981161813167071, 0.7560954579232749, 0.7244176046468488, 0.7108305621069824, 0.718204650734365, 0.7441150394580835, 0.7812106743682087, 0.8183931962770272, 0.8425254654823089, 0.8406177118076219, 0.8019301699596733, 0.7197425435843314, 0.5926686710089698, 0.4251140503775492, 0.22683136067452989, 0.011660330280988253, -0.20423795622266205, -0.4045792942890271, -0.57504838691632, -0.7051937005816177, -0.7897661684393493, -0.8293068652572223, -0.8299006515155186, -0.8021229049955473, -0.7594233513128958, -0.715953221878639, -0.684307426439313, -0.6734048186040171, -0.6868570522140265, -0.7221874426788824, -0.7708237442647581, -0.8191585903691571, -0.8505818015508355, -0.8481661462885941, -0.7977634650762118, -0.6909214820858487, -0.5271825682100394, -0.31525436879598623, -0.07267661804829456, 0.17610311762416703, 0.4028796348907104, 0.5798206568779839, 0.6838352068807156, 0.7004218263991402, 0.6263585027788804, 0.4707037347107586, 0.2537801245269521, 0.004363575376446024, -0.244425088845282, -0.45988451941533137, -0.6143614233710846, -0.6889802592692622, -0.675810131006379, -0.5782280367437729, -0.40962067096108434, -0.19054676255841746, 0.05481291967260732, 0.3023001215109928, 0.5308329677888366, 0.7244882842042791, 0.8734246012838044, 0.9735701497284382, 1.0253939516322779, 1.0322709072595566, 0.9989018615889086, 0.9300855209250758, 0.8301278260930205, 0.7027757047403482, 0.5516545283139476, 0.38091449347590134, 0.19570631362414656, 0.002354352790910658, -0.19179798997086855, -0.3788570549590451, -0.5510272450358933, -0.7012448562483489, -0.8236915392774603, -0.914039706142418, -0.9694184170252935, -0.9881756409826234, -0.9696303075716558, -0.913918517626886, -0.8220829857364051, -0.6963431828766949, -0.5405016807251724, -0.36031892603430715, -0.16359224329210514, 0.04013418091790215, 0.24018456190270834, 0.425760423266114, 0.5870829268985424, 0.7166197717755273, 0.8099833426954562, 0.8664917523906949, 0.8890606065456064, 0.8835329376488369, 0.8577948250420299, 0.8205354221662687, 0.7800304020582047, 0.7431431506248717, 0.7146443568705966, 0.6969512334183051, 0.6901074157262647, 0.6922880175560046, 0.7003398356906728, 0.7105226229352982, 0.7191652725013788, 0.7233235134334371, 0.7213381284523223, 0.7131072858574705, 0.7002046822080928, 0.6857438943908143, 0.6739876200747604, 0.6696394639541572, 0.6768836675096863, 0.6983161172439467, 0.7338690127516884, 0.7800774899548244, 0.829602819630056, 0.8715371312486556, 0.892620000492053, 0.8790856399483223, 0.8192212166031462, 0.7059749857271942, 0.5391749210900726, 0.3269503040314498, 0.08573815461541592, -0.1612255824786287, -0.386730293143399, -0.5635326559438285, -0.6686383256247854, -0.6872358926309042, -0.6156114857935734, -0.4623211423735695, -0.24733010394610414, 0.0007198102460047476, 0.24863863484628498, 0.4635514254715547, 0.6176104623364325, 0.6918268533027474, 0.6782756201030052, 0.5805134425392992, 0.41210610757403726, 0.19372452237290802, -0.050391409713054024, -0.29611210645789393, -0.5225111093000552, -0.7138701729016586, -0.8605441211993027, -0.9585448112667802, -1.008414026021156, -1.0135648241052666, -0.978745896542667, -0.9087849082692102, -0.8079881948321259, -0.6801285945135653, -0.5287862221062773, -0.35805233939202374, -0.1729861888667504, 0.020116186161511587, 0.21387335563181437, 0.40025748153323093, 0.5712472743319003, 0.7195044185357663, 0.8388895884119506, 0.9249072134737321, 0.9746853929178996, 0.9868923875604191, 0.9616684243967665, 0.9003848901697228, 0.8056175444681817, 0.6810587309328351, 0.5314881726723011, 0.3626554692436761, 0.18103860407685468, -0.006510589607727805, -0.1931114704827839, -0.3722848897831801, -0.5381718770034626, -0.6856313040037053, -0.8101801487665511, -0.9076732803716326, -0.9739618526107378, -1.004716020345832, -0.9956414793795033, -0.9430154749490675, -0.8446500281072215, -0.7011043347997452, -0.516842399364099, -0.3010204717594881, -0.06763754580789842, 0.16514820448340978, 0.37668157665933155, 0.5461920463765456, 0.655552915260347, 0.6920652628903768, 0.6505655304034257, 0.5346883243834851, 0.35661897243093144, 0.13559774776324776, -0.1046718797566402, -0.3394032573081613, -0.5461789593962133, -0.7080955978852922, -0.8157954529602021, -0.8683801331865292, -0.8727983131028657, -0.8421078226859732, -0.7927582081222804, -0.741572331068595, -0.7028423018527019, -0.6860253207439192, -0.6943551977069015, -0.7245345157854167, -0.7675646042411391, -0.8104296201087327, -0.8383601072014226, -0.8373952185694984, -0.7966528302359737, -0.7101309321759165, -0.5776984378988999, -0.40521323182553737, -0.2036592543667804, 0.012419924984258368, 0.22695341747885692, 0.42449093142276867, 0.592188438033417, 0.7212965033681705, 0.8079364234726191, 0.8532668165288172, 0.8627953034872611, 0.8451288060001957, 0.8104079963441455, 0.7687359339278867, 0.7287670505538517, 0.6967245108747491, 0.6759780606536095, 0.667107406232625, 0.6684364317450245, 0.676784919616326, 0.6884291860003884, 0.699890853611944, 0.7085144901744879, 0.7128097205123256, 0.7124229876828518, 0.7080187790236897, 0.7008050101089057, 0.6921805709227881, 0.6834646736814466, 0.6757033963031507, 0.669648508318143, 0.6657328144726218, 0.6642652636337992, 0.6653767657521718, 0.6690028595853793, 0.674775333959487, 0.6819477949985021, 0.6893278789128267, 0.6953927726157616, 0.6985573048815797, 0.697578095425808, 0.6920506573747554, 0.6828307951888688, 0.6722732265164824, 0.6640958466160822, 0.6627912256868634, 0.6726965874495441, 0.6967609587320983, 0.735252994349721, 0.7847852487718341, 0.837860611588047, 0.8832021671865116, 0.9070282265831913, 0.8950883370622812, 0.8352994933427401, 0.720489591403177, 0.5506306635171825, 0.3342725070105252, 0.08840692523651153, -0.16315427404215097, -0.3926718560799536, -0.572539734272038, -0.6796338477180948, -0.6992149062771553, -0.6277630208203462, -0.4741131473050659, -0.2585293695095081, -0.009930257048617025, 0.23830892263310452, 0.45325402085890604, 0.607121618765611, 0.6810319795543738, 0.6672310461853316, 0.5694827757707117, 0.4015147931896041, 0.1841817171712272, -0.05817646638242799, -0.3014136753019013, -0.524665532969832, -0.7124274384065621, -0.855285246094759, -0.9495933688767533, -0.996236130847489, -0.9989838487955423, -0.9628841324499167, -0.8930056180780918, -0.7937877561121499, -0.6689704942642202, -0.5220072798874036, -0.3566099133872175, -0.17731129436958973, 0.010268861422383327, 0.19945198638565087, 0.3827826926443024, 0.5526251582270405, 0.7017697482270308, 0.8239876507426606, 0.9144785689512498, 0.9699591512942685, 0.9886252045487814, 0.9700306803372667, 0.9149020439452162, 0.825116863065968, 0.7036983705130238, 0.554839481392563, 0.3840291620621759, 0.19787647745423148, 0.003860727052948984, -0.18999525295737457, -0.3757044734833313, -0.5458056810042837, -0.69378287602043, -0.814366828718361, -0.9036469275456485, -0.9588849469775574, -0.9783006504455267, -0.960973889608092, -0.9067746467203663, -0.8165903751017708, -0.6926507402482928, -0.5388812935652539, -0.361228905014989, -0.16771060388912773, 0.031903370124330505, 0.22678679843602859, 0.4061707941853134, 0.5606402717569381, 0.6832891050414109, 0.7705901219032752, 0.8228006526178891, 0.8436430103344122, 0.8394755303225311, 0.8180394512925253, 0.7871333265278456, 0.7534665911565442, 0.7219614630178657, 0.695510686451852, 0.6753252498343544, 0.6615878037807406, 0.6542998195364643, 0.6538606147644473, 0.6612723675386262, 0.6778625191525914, 0.7044242088089868, 0.7402649399766673, 0.7822594926239343, 0.8241634231439008, 0.8566831085547093, 0.8684082810681567, 0.8475040183712003, 0.784012885063017, 0.6722056874933439, 0.5125005393952523, 0.31260026449095785, 0.08722135068631567, -0.14339658857823498, -0.35611765704885123, -0.5282733760242059, -0.6409441045045646, -0.6818156450864503, -0.6469272017629891, -0.5410574986904879, -0.37652152921039295, -0.17097947697100876, 0.05541171165914345, 0.2829619347828144, 0.49484727767121917, 0.6786113633855301, 0.8264573551553331, 0.9345361200971587, 1.0015661687984379, 1.0272888190262575, 1.0112965146842847, 0.952583288738177, 0.8500890658990591, 0.7039257931121476, 0.5171900515296706, 0.29764273007471115, 0.05870661463653025, -0.1806017914741214, -0.39721826601913907, -0.5668036345777544, -0.6674573482841338, -0.6836867328922335, -0.6099467963750959, -0.4528161959244535, -0.23123780147788525, 0.0254037230819288, 0.2810884215045038, 0.4984727203603391, 0.6447055580185417, 0.6967676536286352, 0.6455398584402634, 0.4976568874522828, 0.2746594289249686, 0.009825427460916032, -0.25698435822392646, -0.4855514161032739, -0.6415528231225354, -0.7018627722542645, -0.6580125604775775, -0.517265265222927, -0.30121265695938104, -0.04212438479079229, 0.22217065809727116, 0.45405673442103006, 0.6217149465148919, 0.7033449800412358, 0.6897787566619501, 0.5850104229528822, 0.4047415306155254, 0.17323834921239678, -0.08075812096424864, -0.3284327261412435, -0.5448733152596168, -0.7121625353086042, -0.8211818337976253, -0.8719691969355644, -0.8727186157199347, -0.8376486334880819, -0.7842590106698991, -0.7303274268398209, -0.6909814362358659], "Decimated Array"=[0.7327573786203745, 0.8571160437398065, 0.9481227692632541, 1.003980881033979, 1.0238155370523472, 1.0072368286759465, 0.9541994905916551, 0.8651912730450063, 0.7417811878517194, 0.5871636451740783, 0.40676677760888635, 0.20846130324205578, 0.0022318875001048045, -0.2005410967663612, -0.38829860023304064, -0.5506845398656813, -0.6799031648608087, -0.7716987861234258, -0.8258475294329478, -0.8459996756657396, -0.8388616433189412, -0.8130753155007096, -0.7778435482452709, -0.7416372990136377, -0.7111421642681004, -0.6905831950739342, -0.6815454430666558, -0.6831516021872707, -0.6925669267273694, -0.7057731727702966, -0.7184007879882285, -0.7265282476091678, -0.727382953469249, -0.7198001905615271, -0.7045629848520147, -0.6843705475932246, -0.6634185556136458, -0.646887119577886, -0.6400361359583534, -0.6471594714631548, -0.6704579022356528, -0.7090564063186768, -0.7584053880552923, -0.8101244036157627, -0.8526189235085075, -0.872417498261418, -0.8561767863823757, -0.7930533916017833, -0.6770604606987946, -0.5089375701527854, -0.2971550620890392, -0.05761269204799846, 0.18789151496970918, 0.4143336303799478, 0.596919125262307, 0.7147087986695557, 0.7538529097411865, 0.7097353627437273, 0.5877778836770051, 0.40257278286196346, 0.1755748921605498, -0.06817834720063913, -0.30381917292160493, -0.5101473732591594, -0.6722715103438465, -0.782942771822579, -0.8426075541528982, -0.8581499860345086, -0.8406550377330191, -0.8028915815603971, -0.7569445207502417, -0.7124441110679234, -0.6756211416707443, -0.6492985792878058, -0.6336104831921037, -0.6270868628284776, -0.6278993868440812, -0.6347460148648578, -0.6473189374357599, -0.6660652122000107, -0.6914774106844375, -0.7231297220029862, -0.7587664029448702, -0.7936544758660282, -0.8205522923344901, -0.8305429506490288, -0.8142884856193261, -0.7636823212203829, -0.673529581873597, -0.5429181777841331, -0.3758793938755062, -0.18113858110834186, 0.028812354472331908, 0.23939310934756888, 0.4359274511900307, 0.6056519046787863, 0.7393627898718214, 0.8324327306148087, 0.8851319247653551, 0.9020886016493107, 0.8911142062914292, 0.8617307665544903, 0.8235701121823792, 0.7850172209229723, 0.7522557788351737, 0.7288635601528786, 0.7158958847588804, 0.7123277223581522, 0.715761845721655, 0.7231900323302534, 0.7316880970831603, 0.7389528359720056, 0.7435736461024193, 0.7451046063677472, 0.743901281226759, 0.740788821822152, 0.7367782401995692, 0.7328033193551644, 0.7294981194191762, 0.7271513904156902, 0.7257726558576425, 0.725159941446078, 0.725060989178965, 0.7252632377419967, 0.7256163395829798, 0.7260606904500417, 0.7265379023034586, 0.7270291732601397, 0.7275033865931528, 0.7279199682707127, 0.7282769079854728, 0.7285974590770533, 0.7289407767207793, 0.7293428506461535, 0.7298479408102396, 0.7304778513692572, 0.7311828384458046, 0.7318265401385785, 0.7323028750384627, 0.7325567749966301, 0.7325033028493253, 0.7321158823152807, 0.7314068004824351, 0.7304533892028899, 0.7293390182016347, 0.7281572743585262, 0.7270606197087242, 0.7261241067000211, 0.7253508195631971, 0.7246697616263047, 0.723969429286671, 0.723139564739256, 0.7220976758138733, 0.7208555865072881, 0.719568292828321, 0.7184478733558384, 0.7176993275862744, 0.7174622207349447, 0.7177521937986072, 0.718516228428159, 0.7195981106474233, 0.7207879819353863, 0.7218924194293399, 0.7227111613943498, 0.7231168859595661, 0.7230786498664554, 0.7226411424851807, 0.7219463720454906, 0.7211811690986409, 0.7204810710907097, 0.7199538718599565, 0.7196320372423504, 0.7194607411817737, 0.7193099127963588, 0.7190971249818399, 0.7188635612803779, 0.7188051788075457, 0.7192369464355841, 0.7205351477714964, 0.7229401499987833, 0.7263486481418566, 0.7301617369824043, 0.7333271712095472, 0.7344308070476105, 0.7320183145085448, 0.7250816880667706, 0.7135657369657201, 0.6987104127947069, 0.6831567860992641, 0.6708043964638186, 0.6662258399732381, 0.6737496016563864, 0.6962181897094762, 0.7338123953236427, 0.7831464621140352, 0.8367458472751513, 0.8833813981307604, 0.9091987678800104, 0.8998091259693833, 0.8428401153753142, 0.7305998791526044, 0.562507495226734, 0.34659814194077, 0.0995702257773744, -0.15462281131582128, -0.3875977492359962, -0.5706271624637833, -0.6790839949047796, -0.6967382767827438, -0.6189803271815245, -0.4544562375583789, -0.22459908414379984, 0.03903553601854455, 0.29916696405087967, 0.5182679460830586, 0.6643639077354586, 0.7159339540668409, 0.6652943920234429, 0.5198749673865217, 0.300993470244488, 0.04051717061424443, -0.22409581460784916, -0.45544556602126973, -0.6216785191074483, -0.7008762468325049, -0.6837610820977862, -0.5742886326760264, -0.3883111156265534, -0.1505286326662823, 0.10967239939698414, 0.3627475020866999, 0.5831487815378037, 0.7525668303202456, 0.8617987081334637, 0.9111768991603971, 0.9094611758407977, 0.8715862070139058, 0.8157455416667302, 0.760202018310825, 0.7202658930923688, 0.7058888207208955, 0.7201847936946834, 0.759052366114439, 0.811812333812609, 0.8630070563777121, 0.8948697888398245, 0.8903643946442023, 0.8361831300618912, 0.7252589385855543, 0.5584821670091451, 0.345315670477598, 0.10299763765352206, -0.14547539122840722, -0.37428698339337824, -0.5583637418127292, -0.6768312337753024, -0.7159704258460882, -0.6711625159308375, -0.5476542552431498, -0.3597709705436185, -0.1287724532856077, 0.12018518168690656, 0.36151984386717273, 0.572699142103299, 0.7370284868429373, 0.8455964386542135, 0.8979126579643226, 0.9012807607635166, 0.8690744380604796, 0.8181990426007191, 0.7661088030574076, 0.7279245613823432, 0.7140037167311404, 0.7282038712248695, 0.7671972819282604, 0.8208631561250372, 0.8738564756136162, 0.9080475656744531, 0.9055112204914009, 0.8518434216042863, 0.7389767670280546, 0.5673122043840576, 0.346672036977057, 0.09563946895916749, -0.1604955961723308, -0.3929887785452873, -0.573731438794397, -0.6795623772004052, -0.6960013467696725, -0.619916032405668, -0.46047605211853976, -0.238293779549608, 0.017302276506560462, 0.2723050965454336, 0.4928472153853533, 0.6499682346772773, 0.7235856630223708, 0.7050531042870595, 0.5980296925245243, 0.4173625434472803, 0.18635581949974522, -0.06697296685650257, -0.3141616680583659, -0.5303108718258116, -0.6972846806923089, -0.805693295562243, -0.8554610680619644, -0.8548810350527455, -0.8184903429533198, -0.7641725094683359, -0.7100008771843999, -0.671228658984871, -0.657884155216942, -0.6731679025330721, -0.7131015741595147, -0.7671687462263975, -0.8200654189127506, -0.8542004537564716, -0.8526249939936517, -0.8019646550151107, -0.6949224336608516, -0.5320250473508275, -0.32225185034324333, -0.08237582607009868, 0.1650026835738332, 0.39428466394542017, 0.5803342409591474, 0.7020686940954762, 0.7453870445521058, 0.7052505477960299, 0.5864589514160631, 0.40293010537214813, 0.17562748086081167, -0.0704552502607787, -0.309822690701368, -0.5200321703524325, -0.6844918028247094, -0.7944039739927944, -0.849369247148433, -0.856656043797114, -0.8292787623167311, -0.7833804658452638, -0.7353387812407823, -0.6989933350482087, -0.6835224068604273, -0.6921158238785066, -0.7217188264252835, -0.7637517506720419, -0.8057159017858148, -0.8333093620537693, -0.8327870038627241, -0.7931510688939891, -0.7079388773369498, -0.5762895149017982, -0.4032287101039275, -0.19912345762738048, 0.021626092972811716, 0.24243838454530214, 0.4466281803126936, 0.6195670275196116, 0.7505384293302241, 0.8341667424696944, 0.8710515511074273, 0.867618588313726, 0.8350546605288388, 0.7875968290108912, 0.7403153596554869, 0.7065887377614032, 0.6958348088594112, 0.7117510991794384, 0.7514265747295997, 0.8055501080993405, 0.8597172027233948, 0.896672112950365, 0.8992716440220376, 0.8535956532880161, 0.7516973279064126, 0.5935739768219647, 0.3879409425761628, 0.1514795080598367, -0.09323685375808283, -0.32079142716179476, -0.5065138588773618, -0.6300491223171335, -0.6781015202421304, -0.64619431762589, -0.5389832779795898, -0.36913308344851997, -0.15510153259215717, 0.08166236993095077, 0.3196509591252603, 0.5398927777919778, 0.7276930986154884, 0.8734985979773947, 0.9728047077610658, 1.0252642302363124, 1.0333899494712895, 1.0012329554745556, 0.9333027118497857, 0.8339401572384909, 0.7072095654921254, 0.5571462896311223, 0.3881483450425459, 0.20534155782487487, 0.01482887737245796, -0.1764521290488, -0.3611157500299354, -0.5318043493520626, -0.6818066642899347, -0.8054524101831724, -0.8983255342414102, -0.9572814410830893, -0.9802961943453828, -0.9661962276209902, -0.9145882909024544, -0.8259958203690237, -0.702124108056222, -0.5463111553516156, -0.3640099142702318, -0.1630068815984123, 0.04665386649189137, 0.25324056756651203, 0.4443960991039263, 0.6085609531447825, 0.7365289833752492, 0.8228996922007434, 0.8670933837874918, 0.8736111453366721, 0.8515289789816484, 0.8132403002190881, 0.772465080941647, 0.7419679771548864, 0.7313371097907961, 0.7450271466496866, 0.7811915546642222, 0.8315498322037654, 0.8823689588265033, 0.9165305921773814, 0.9163401501954511, 0.866798433796903, 0.7586596196292686, 0.5908492722170399, 0.37178062020046765, 0.11907890680745346, -0.14211821683680798, -0.38238233257874527, -0.5721392733995939, -0.6862057323913836, -0.7079902911617727, -0.6327143381258475, -0.4689575875843263, -0.23816585088733142, 0.02788728184520496, 0.2913733998865506, 0.5138745348418566, 0.6622161891528019, 0.713630396728027, 0.6595409016687056, 0.5072353110800646, 0.2790535214186103, 0.009173689804918802, -0.26151320666451255, -0.49168518087347146, -0.646028784822539, -0.7007240447824197, -0.6471884427151815, -0.493530539618674, -0.2632018631271933, 0.008643095196815533, 0.28067049342689865, 0.5117662020698565, 0.667360375596674, 0.7246614220304907, 0.6758948089830248, 0.5292499968474088, 0.30723953882700833, 0.04292589220225078, -0.22522884697938184, -0.4592044373314265, -0.6269083921942394, -0.7064584618733396, -0.6888404338934664, -0.578411648288706, -0.39139022626549447, -0.15271914914807735, 0.10811456934185323, 0.36154443524920665, 0.5821113615057549, 0.7515472341269214, 0.8606474547165524, 0.9096953707888916, 0.9073268916916939, 0.8684122594374747, 0.8110629523849187, 0.7535131577918508, 0.7111116174600383, 0.6939391865838809, 0.7053500144234236, 0.7415364458091326, 0.7922663020024436, 0.8425535702269459, 0.8751141872059586, 0.8732034679792344, 0.8235993150699542, 0.7190183727683939, 0.5598342988350936, 0.3547305255173707, 0.12000835651727722, -0.12227364288086777, -0.34712620885755746, -0.5299758484536152, -0.6500817333967435, -0.6934598211856411, -0.6548680069310724, -0.538631179832801, -0.35797405653961106, -0.13314154269390344, 0.11150249461783546, 0.3507932103438662, 0.5622006640712187, 0.7287398470888085, 0.8409123226340982, 0.8975410491756267, 0.9052474392037568, 0.8767801125750505, 0.8285828512227308, 0.7778392815717208, 0.7394654445105879, 0.7237013633767214, 0.7343864257619723, 0.7683602106205176, 0.8160146443370595, 0.862832671453382, 0.8918135732392275, 0.8863825849799384, 0.8334021521345413, 0.7256529739097736, 0.5635985512953553, 0.35608386653185525, 0.1195604135723027, -0.12374840459859741, -0.3487502236997944, -0.5308687349642771, -0.6495113130900928, -0.6909901985488635, -0.6504937240912037, -0.5328353201969774, -0.3517349807169625, -0.12783984379196844, 0.11423012543166067, 0.3492730631198282, 0.5549865684462535, 0.7147604584382636, 0.8196924285734603, 0.8692925730239803, 0.8708584840188425, 0.8377913064207088, 0.7870129074549828, 0.7359765930553231, 0.6996793525556969, 0.6881560723752628, 0.7048218776482567, 0.7458257319106636, 0.8006775631265496, 0.853917719961837, 0.8877440401214893, 0.8850693181898429, 0.8326613733709883, 0.7236976539802175, 0.5594490106415803, 0.3497538967519691, 0.11201578047048573, -0.13100695912350224, -0.3542636347146736, -0.5338912711941378, -0.6506028489493497, -0.6922424302133595, -0.6552909494544218, -0.545064832644278, -0.37448254797377645, -0.16191455440330382, 0.07162348789175096, 0.305307696187205, 0.5209397804835978, 0.7045483839307563, 0.8471495500869136, 0.9446334649114675, 0.9967359029755237, 1.0058177131022314, 0.9755714551521117, 0.910087443335543, 0.8133163625595331, 0.6890103411064745, 0.5410140712172831, 0.37367966894661164, 0.19222351735516607, 0.002885008671315868, -0.18723164421141011, -0.3706358231842831, -0.540017664941237, -0.6887965775506286, -0.811456181705438, -0.9037768968384509, -0.9627749707154154, -0.986428591882344, -0.9734798839005043, -0.9233425758887451, -0.8362626385273748, -0.7136342940914308, -0.5585921807071323, -0.37653877807456615, -0.17539608244694269, 0.03449829302119377, 0.24108409799518699, 0.4317114568156308, 0.5946337468390553, 0.7205719868506776, 0.8042233087437884, 0.8452649724027359, 0.8485537347599877, 0.8236121116636361, 0.7832470748996688, 0.7415340851598169, 0.7114139852567443, 0.7023916754066073, 0.7186444625002776, 0.7579146977658392, 0.8114788518364714, 0.865212362785649, 0.9017186145139675, 0.9031789704236397, 0.8546836474975438, 0.7473081616445082, 0.5805118731598218, 0.3633604703375262, 0.11403099657073672, -0.1421571689009856, -0.376100265224383, -0.5591208341865042, -0.66748156416295, -0.6863264429683489, -0.61238919788703, -0.45495950013783854, -0.2348765682622349, 0.018329318180048494, 0.27072256893627067, 0.4888669989484364, 0.6445441082266234, 0.7186091906642366, 0.7032516717681991, 0.602286440359839, 0.4297305321288512, 0.20693427048046936, -0.04118448970582595, -0.2899486028515708, -0.51813884111226, -0.7100679145508004, -0.8564812364022516, -0.954078154354838, -1.004051301932304, -1.0102212014763818, -0.9772535580383042, -0.9093646718646989, -0.8097976595431309, -0.6810878313976068, -0.5258335391357575, -0.34780340225624445, -0.15283789222057037, 0.05073422541995442, 0.25233190333965977, 0.44007238959276546, 0.6022906295601135, 0.7293932651728482, 0.8155001380288734, 0.8596440510683021, 0.8661244160018878, 0.8440053760191001, 0.8057116144877121, 0.7648934322393982, 0.7341019522530025, 0.722408788035578, 0.7335846743805764, 0.76523665163658, 0.8088069415554398, 0.8508057382972929, 0.8750784439185956, 0.8656525197192184, 0.8097364952043214, 0.7004331018480651, 0.5385134797346247, 0.333020638982082, 0.10055243220663874, -0.13684916712333142, -0.3547046170347631, -0.5296187059445376, -0.6427036804094352, -0.6822150791593455, -0.6450059416608724, -0.5366580259087476, -0.37013892662339776, -0.16344566761793425, 0.06325834047144631, 0.29051687792880865, 0.5019090102948002, 0.685337537979504, 0.8332571783100664, 0.9419059935710599, 1.0099338897337269, 1.0368536824281052, 1.0219112826998396, 0.9637216757298569, 0.8608644035958495, 0.7132682495621445, 0.5240958995354725, 0.30150783203128084, 0.05962244367312289, -0.18169903701790627, -0.3985650165893692, -0.5660874768283738, -0.6622779885806316, -0.6721281174161831, -0.5910217986061128, -0.4267122427659796, -0.19931344093386746, 0.06087906417721856, 0.31748163584889194, 0.5333437531858058, 0.6763479522156483, 0.7245443113283739, 0.6697558890344962, 0.5190710655465737, 0.2937181748767438, 0.02576020244976748, -0.24681249668741956, -0.4858948596428177, -0.6588635605451997, -0.7431160183824671, -0.7289134552508003, -0.6200694296515479, -0.4325067812603366, -0.19121024572221312, 0.07400166309693594, 0.3330849816678037, 0.5599873834891823, 0.7359349670621476, 0.8513661111199331, 0.9063246869034065, 0.9094064046484032, 0.8755054075051303, 0.8228032542069148, 0.7695512733800192, 0.7310864566365781, 0.7174344380700259, 0.7318771929311987, 0.770521492507058, 0.8229990169861556, 0.8741669857800006, 0.9065945000702298, 0.9034290410951017, 0.8513488075060012, 0.7431105593701001, 0.5792771762670239, 0.3688585907869233, 0.12855873457058717, -0.11905374155741394, -0.348465451110149, -0.5346000660767498, -0.6563026294503328, -0.6993804544754962, -0.6586232637177873, -0.5386587210945445, -0.35325412329016936, -0.12340944757935825, 0.12562838916868907, 0.3678984527083349, 0.5802535686096911, 0.7453566040596344, 0.8536797217461267, 0.904341743696613, 0.9045288934223483, 0.8678005605218305, 0.8115232656672823, 0.7538338251356304, 0.7106289265654393, 0.6929469282521439, 0.7051665302164144, 0.7441987520198292, 0.7999632255413621, 0.8568697593576841, 0.8963183241181077, 0.8998019936252488, 0.8522424023181564, 0.7449696798222867, 0.5778551163588856, 0.3603125530553699, 0.11070054945898282, -0.14570230635299203, -0.3799809948767624, -0.5637043781173343, -0.6732548027150764, -0.693664788209523, -0.6213306289901542, -0.46505052769065697, -0.24516543111583403, 0.0090596915946915, 0.2635428251223252, 0.48417637041829653, 0.641689526437302, 0.7157173189250563, 0.6973828411174359, 0.5901314098610099, 0.4086428546496129, 0.17619718572689294, -0.07917988137166046, -0.328937783780878, -0.5480728892646238, -0.7183409139718169, -0.830216292312652, -0.8834929518448947, -0.8862829283786646, -0.8529835994516479, -0.8013536812216641, -0.7493136237212195, -0.711957955660661, -0.6991338441055578, -0.7139427031909754, -0.7523268372875261, -0.8037761996631599, -0.8530893578229929, -0.8828792296977179, -0.8764987725251604, -0.8209490836280732, -0.7093747657586275, -0.5427215391631399, -0.33033331822457584, -0.08916763854378294, 0.15803966171501063, 0.3856904000524847, 0.5687642313471672, 0.6864040238926279, 0.724868684652829, 0.6795420414253549, 0.5557211678730963, 0.3677696222282419, 0.13706564016321376, -0.11113892216576668, -0.3513165038596046, -0.5611655218564168]}] caption="Constellation Graph"
  out "Sync Found 3":bool=TRUE
  out "Correct Packets Rx 3":i16=46
  out "Singal & Noise Power 3":cluster{"signal_power":dbl, "noise_power":dbl}={"signal_power"=0.000719802679436105, "noise_power"=8.71918670194843e-09}
  out "error out 6":errorcluster
  out "Cumulative Packets Recovered 3":i16(graph)=46
  out "Signal and Noise Power Tracking 3":cluster{"total_power":dbl, "noise_power":dbl}(graph)={"total_power"=0.000719802679436105, "noise_power"=8.71918670194843e-09}
  # "Guard\nBand"
  # "Sync\nSeq"
  # "Packet\nNumber"
  # "Pad\nData"
  # "Blank\nFrame"
  # "Data"
  # "Guard\nBand"
  # "Sync\nSeq"
  # "Packet\nNumber"
  # "Pad\nData"
  # "Blank\nFrame"
  # "Data"
  # "Guard\nBand"
  # "Sync\nSeq"
  # "Packet\nNumber"
  # "Pad\nData"
  # "Blank\nFrame"
  # "Data"
  # "Guard\nBand"
  # "Sync\nSeq"
  # "Packet\nNumber"
  # "Pad\nData"
  # "Blank\nFrame"
  # "Data"
  # "Guard\nBand"
  # "Sync\nSeq"
  # "Packet\nNumber"
  # "Pad\nData"
  # "Blank\nFrame"
  # "Data"
  # "Guard\nBand"
  # "Sync\nSeq"
  # "Packet\nNumber"
  # "Pad\nData"
  # "Blank\nFrame"
  # "Data"
  # "Guard\nBand"
  # "Sync\nSeq"
  # "Packet\nNumber"
  # "Pad\nData"
  # "Blank\nFrame"
  # "Data"
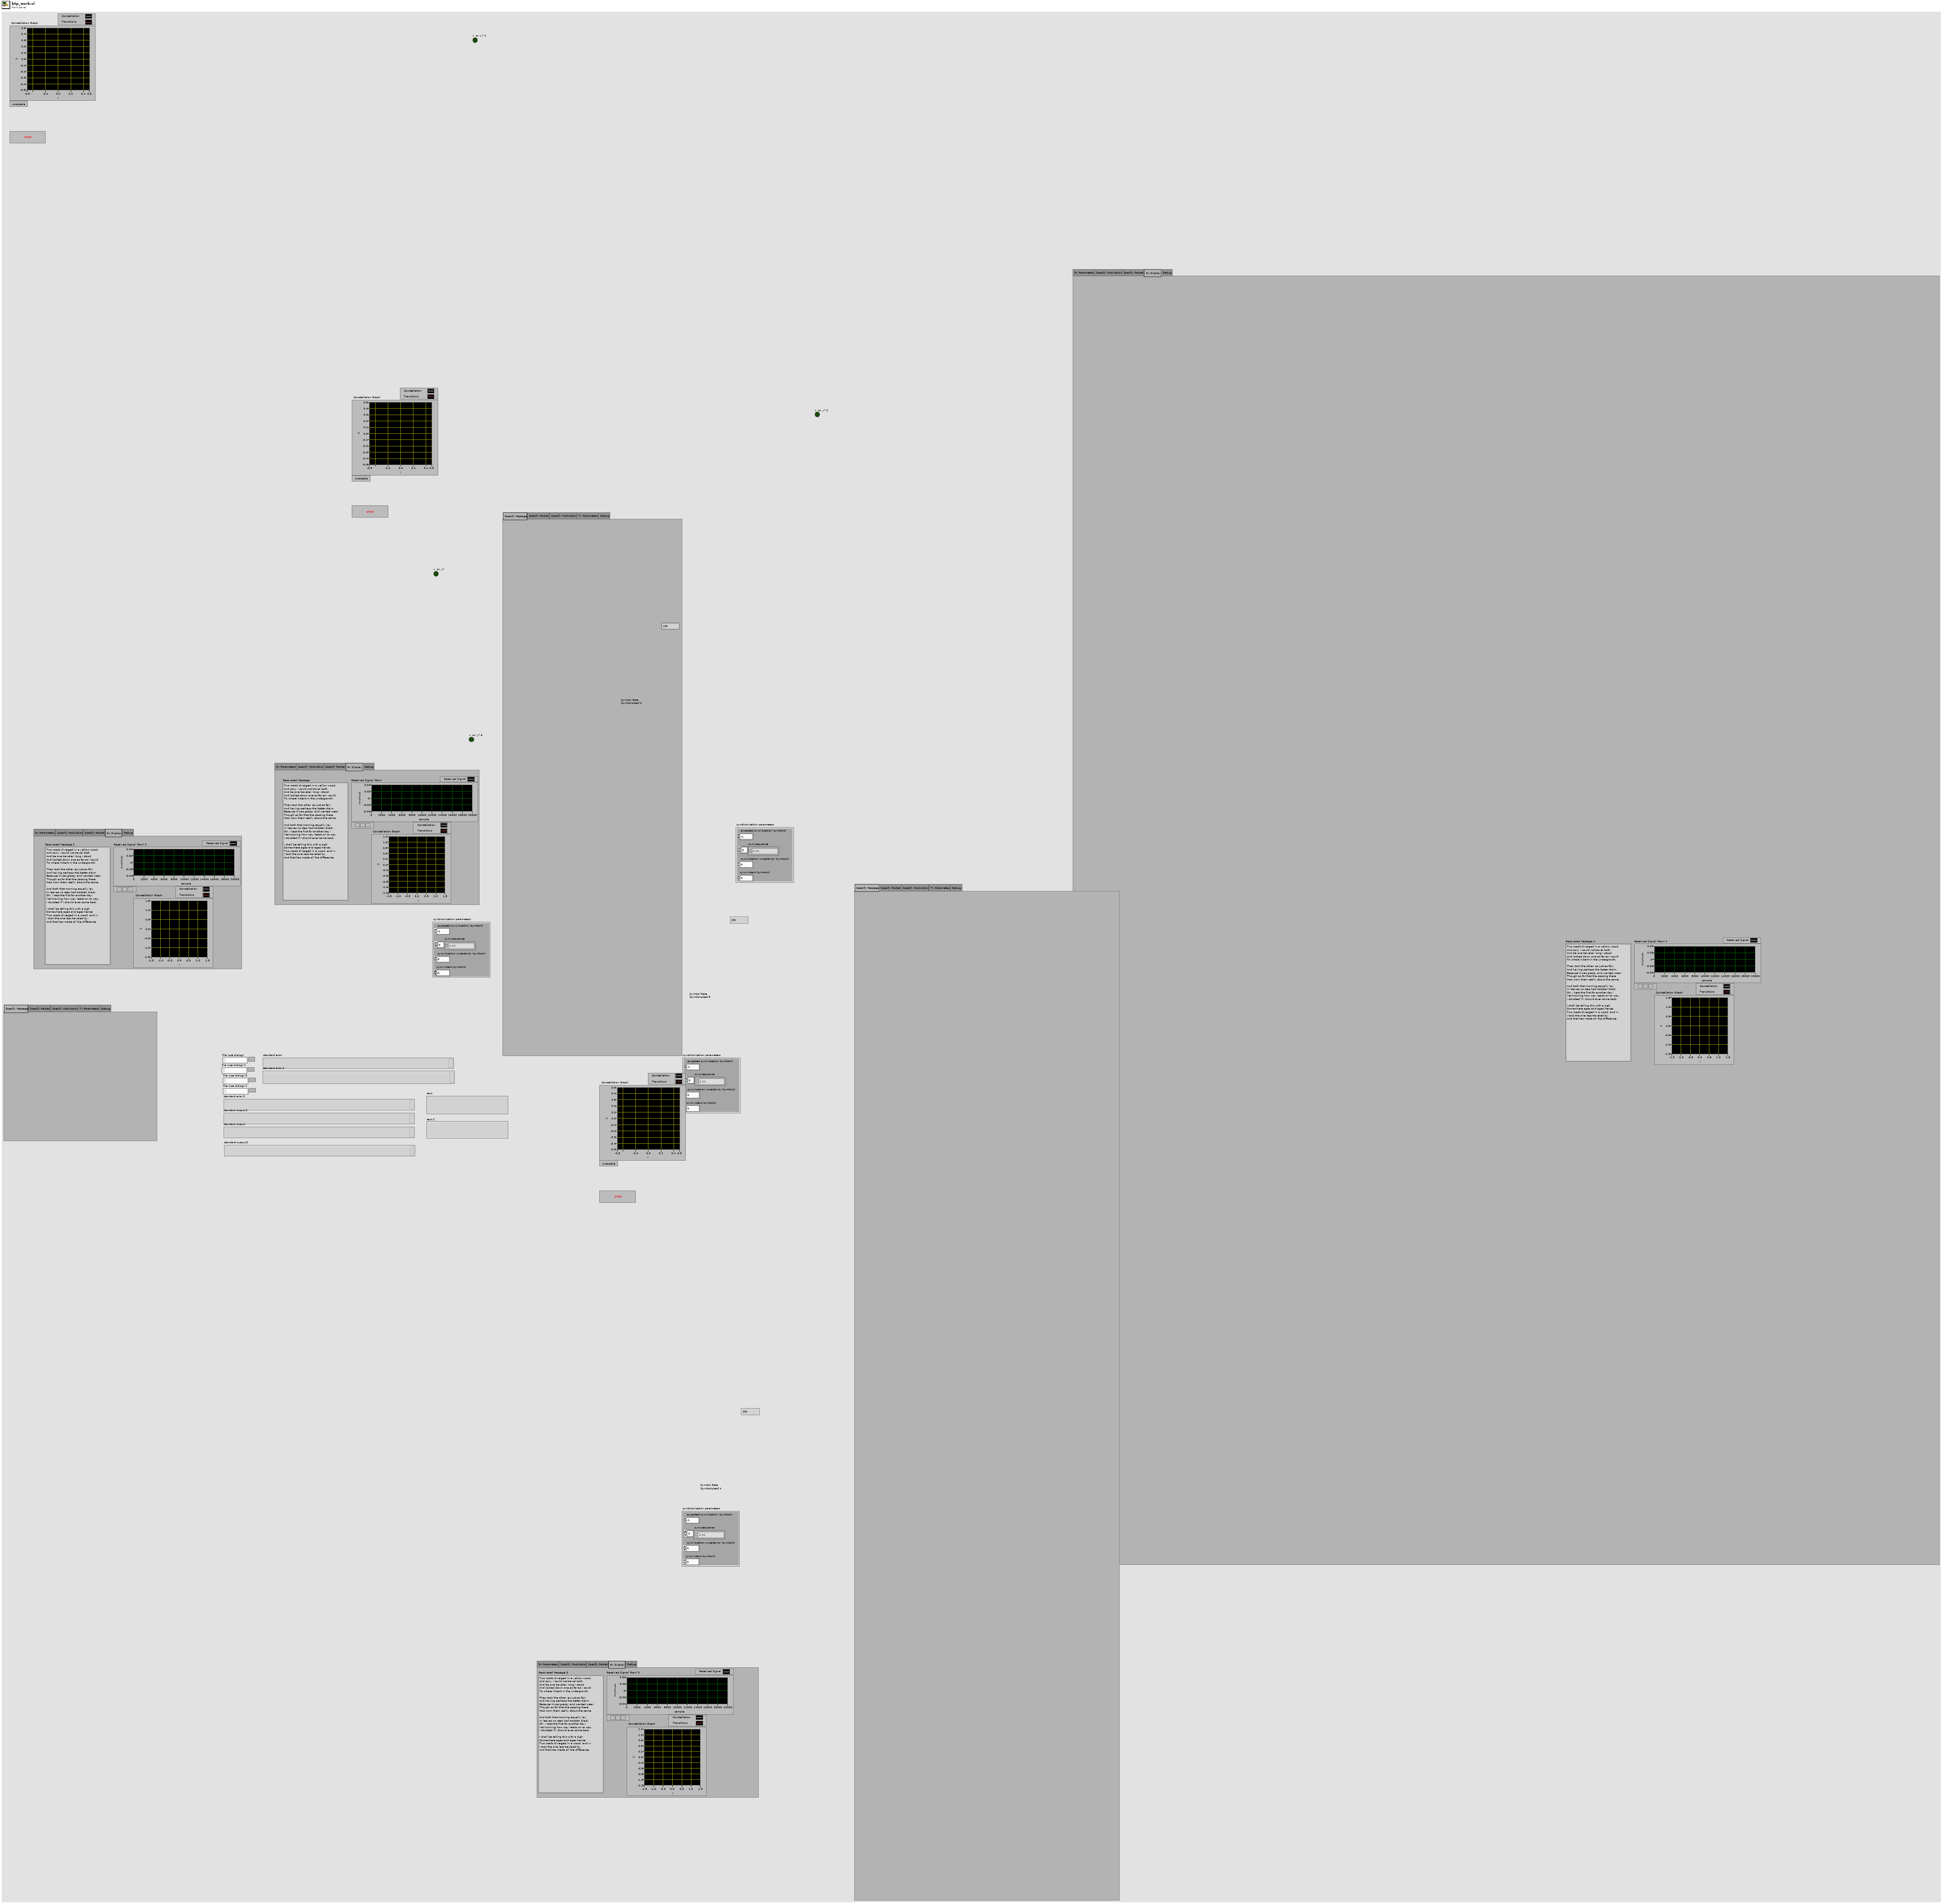
[diagram p1: front panel]
types:
  T1 = cluster{"expected sync location (symbols)":i32, "sync sequence":cdb[], "sync location uncertainty (symbols)":i32, "sync indent (symbols)":i32}
  T2 = enum32{"Rx Parameters", "Specify Modulation", "Specify Packet", "Rx Display", "Debug"}
  T3 = cluster{"Rx IQ Sampling\nRate [s/sec]":dbl, "Rx\nFrequency [Hz]":dbl, "Rx Gain [dB]":dbl, "Rx Antenna":string}
  T4 = enum32{"BPSK", "QPSK", "pi/4DQPSK", "OQPSK", "8-PSK", "16-PSK", "Custom"}
  T5 = cluster{"Samples per Symbol":i32, "symbol map":cdb[], "Differential PSK":enum16{"disable", "enable"}, "PSK type":u16}
  T6 = cluster{"Alpha":dbl, "Filter Length":i32, "TX Filter":enum16{"none", "Raised Cosine", "Root Raised Cos", "Gaussian"}}
  T7 = cluster{"Guard Bits ":i32, "Sync Bits":i32, "Message Bits":i32, "Number of Packets \nto Expect":i32}
  T8 = cluster{"Decimated Array":dbl[], "Decimated Array":dbl[]}[]
  T9 = enum32{"Specify Message", "Specify Packet", "Specify Modulation", "Tx Parameters", "Debug"}
  T10 = cluster{"Guard Bits ":i32, "Sync Bits":i32, "Message Bits":i32}
  T11 = cluster{"Tx IQ Sampling\nRate [s/sec]":dbl, "Tx Frequency [Hz]":dbl, "Tx Gain [dB]":dbl, "Tx Antenna":string}
  T12 = cluster{"Packet Array":i32[][], "IP Array of Pkt Nums Received  ":bool[]}
  T13 = cluster{"bit stream ":i8[][], "Sync Valid?":bool[], "Decoded Pkt Numbers":u32[], "Enable?":bool}
  T14 = cluster{"packet_arr":cdb[][], "Packets Valid?":bool}
  T15 = cluster{"PSK type":u16, "Samples per Symbol":i32, "Differential PSK":enum16{"disable", "enable"}, "M":i32}
  T16 = cluster{"samples per symbol (16)":i32, "symbol map":cdb[], "differential PSK":enum16{"disable", "enable"}, "PSK type":u16}
  T17 = cluster{"PSK system parameters":cluster{"samples per symbol (16)":i32, "symbol map":cdb[], "differential PSK":enum16{"disable", "enable"}, "PSK type":u16}, "pulse shaping filter coefficients":dbl[], "matched filter coefficients":dbl[], "synchronization parameters":cluster{"expected sync location (symbols)":i32, "sync sequence":cdb[], "sync location uncertainty (symbols)":i32, "sync indent (symbols)":i32}, "Sync Bits":i8[]}
  T18 = cluster{"s? t:f":cluster{"t0":dbl, "dt":dbl, "Y":cdb[]}, i32}
  T19 = typedef "niAMT.lvlib/Complex Data Waveform.ctl" = cluster{"t0":dbl, "dt":dbl, "Y":cdb[]}
  T20 = cluster{"constellation":dbl[], "oversampled data":dbl[]}[]
  T21 = cluster{"PSK type":u16, "Samples per Symbol":i32, "Differential PSK":enum16{"disable", "enable"}, "M 7":i32}
  T22 = cluster{"output complex waveform":cluster{"t0":dbl, "dt":dbl, "Y":cdb[]}, i32}
  T23 = cluster{"PSK type":u16, "Samples per Symbol":i32, "Differential PSK":enum16{"disable", "enable"}, "M 6":i32}
  T24 = cluster{"PSK type":u16, "Samples per Symbol":i32, "Differential PSK":enum16{"disable", "enable"}, "M 3":i32}
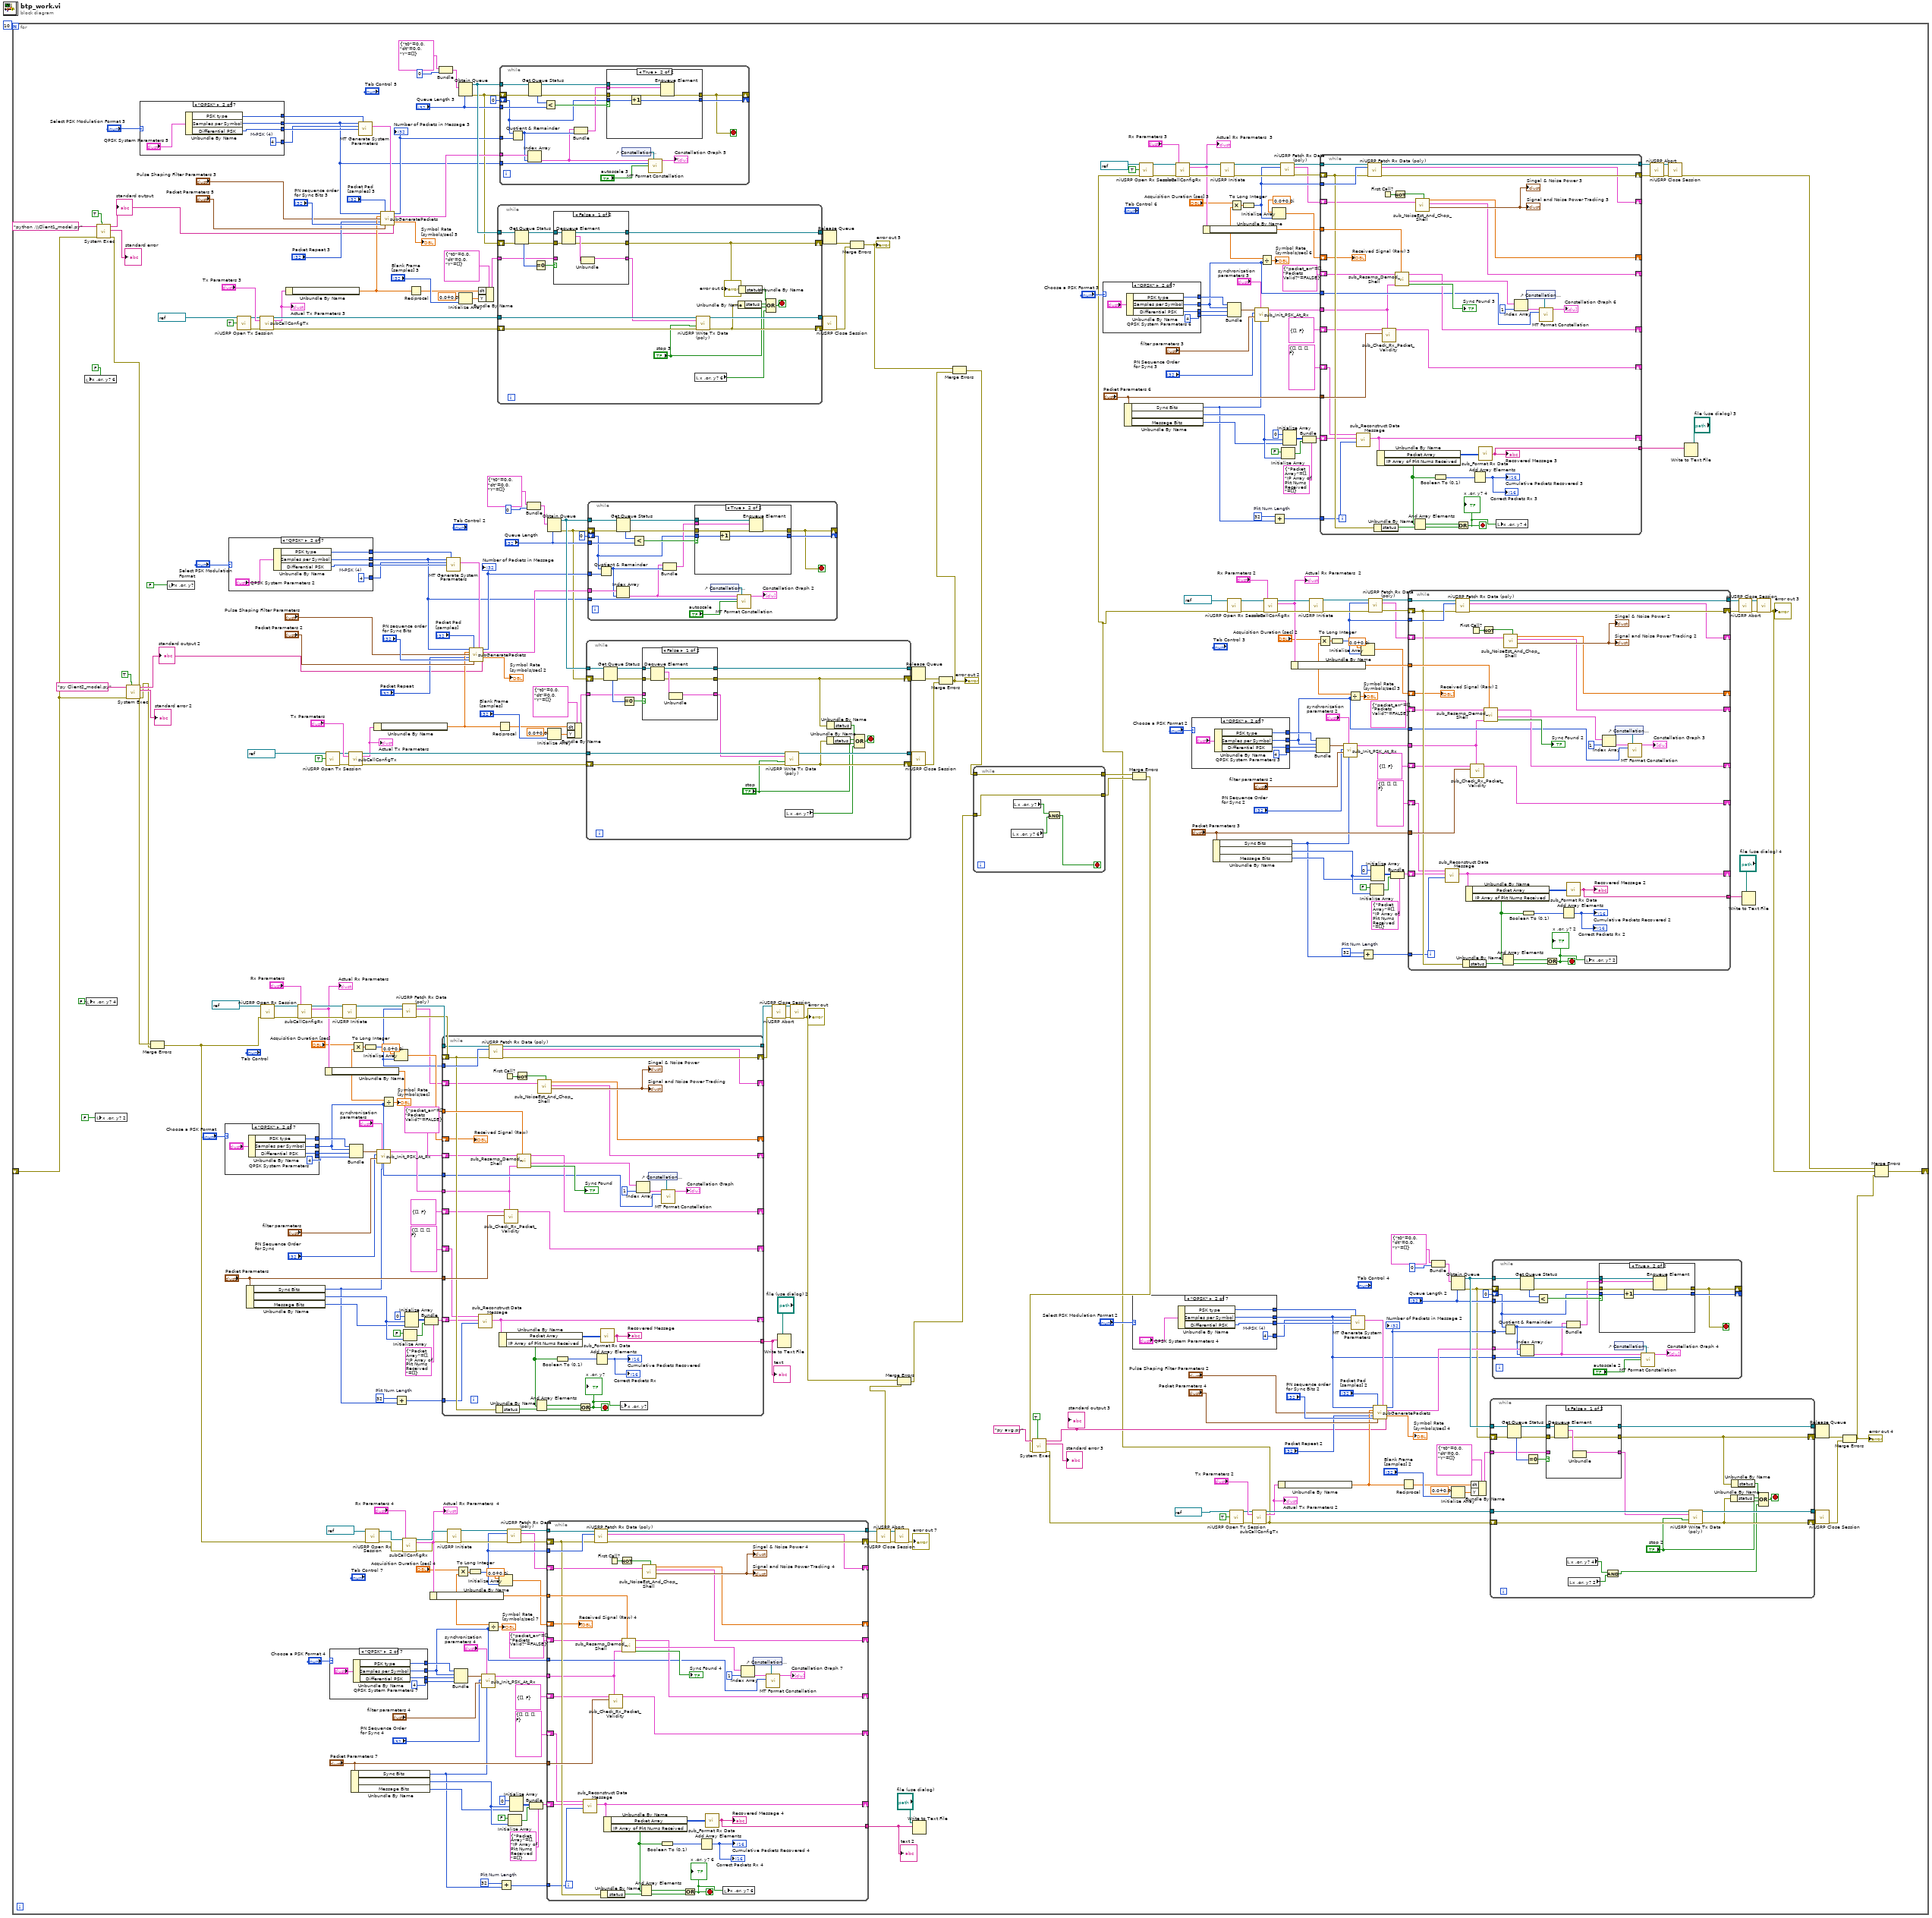
[diagram p0: block diagram]
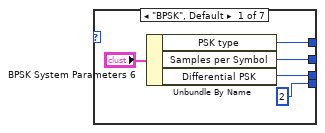
[diagram p2: hidden frame]
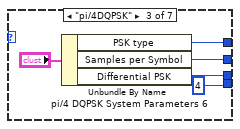
[diagram p3: hidden frame]
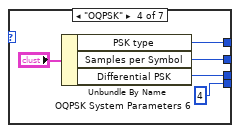
[diagram p4: hidden frame]
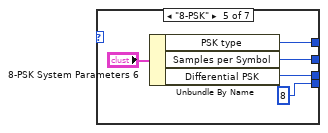
[diagram p5: hidden frame]
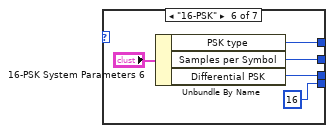
[diagram p6: hidden frame]
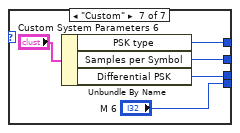
[diagram p7: hidden frame]
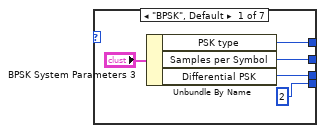
[diagram p8: hidden frame]
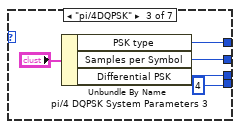
[diagram p9: hidden frame]
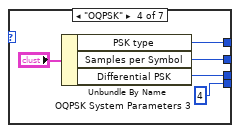
[diagram p10: hidden frame]
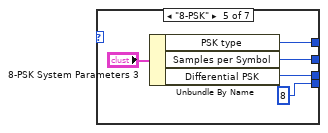
[diagram p11: hidden frame]
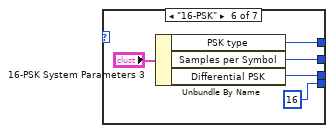
[diagram p12: hidden frame]
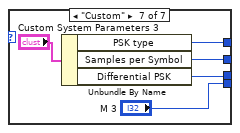
[diagram p13: hidden frame]
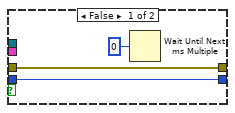
[diagram p14: hidden frame]
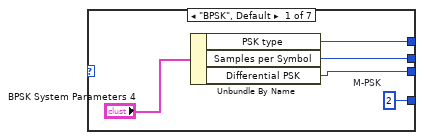
[diagram p15: hidden frame]
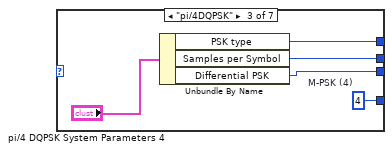
[diagram p16: hidden frame]
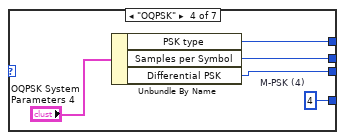
[diagram p17: hidden frame]
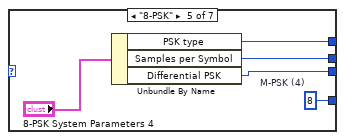
[diagram p18: hidden frame]
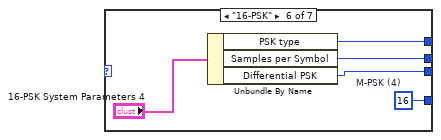
[diagram p19: hidden frame]
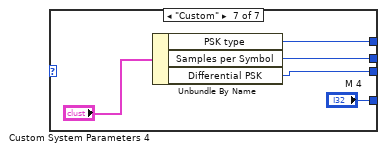
[diagram p20: hidden frame]
diagram:
  n1 = for {
    N: 10 -> [_]
    shift-right: [w29] -> _
    shift-left: _ -> [w24]
    w67 = 32  # Pkt Num Length
    w113 = 32  # Pkt Num Length
    w208 = 32  # Pkt Num Length
    w339 = 32  # Pkt Num Length
    n2 = local write "x .or. y? 6"(FALSE) -> ()
    n3 = local write "x .or. y? 4"(FALSE) -> ()
    n4 = local write "x .or. y? 2"(FALSE) -> ()
    n5 = call <vilib>:"System Exec.vi"("wait until completion? (T)"=TRUE, "error in (no error)"=w24, "command line"="python .\\Client1_model.py") -> ("error out"=w22:errorcluster, "standard error"=→"standard error":string, "standard output"=w33:string)  [unwired: 5 in, 1 out]
    "standard output" <- w33
    n6 = call <vilib>:"System Exec.vi"("wait until completion? (T)"=TRUE, "error in (no error)"=w24, "command line"="py Client2_model.py") -> ("error out"=w21:errorcluster, "standard error"=→"standard error 2":string, "standard output"=w25:string)  [unwired: 5 in, 1 out]
    "standard output 2" <- w25
    n7 = case shown="\"QPSK\"" "Select PSK Modulation Format 3" {
      tunnel: [w712 w716 w724 w729 w734 w740 w743] -> w234
      tunnel: [w713 w718 w723 w728 w733 w739 w744] -> w270
      tunnel: [w715 w720 w725 w730 w732 w738 "M 5"] -> w253
      tunnel: [w714 w719 w722 w727 w735 w737 w745] -> w241
      frame "BPSK", Default {
        w715 = 2  # M-PSK
        n8 = Unbundle By Name("BPSK System Parameters 5") -> ("PSK type"=w714:u16, "Samples per Symbol"=w712:i32, "Differential PSK"=w713:enum16{"disable", "enable"})
      }
      frame "QPSK" {
        w720 = 4  # M-PSK (4)
        n9 = Unbundle By Name("QPSK System Parameters 5") -> ("PSK type"=w719:u16, "Samples per Symbol"=w716:i32, "Differential PSK"=w718:enum16{"disable", "enable"})
      }
      frame "pi/4DQPSK" {
        w725 = 4  # M-PSK (4)
        n10 = Unbundle By Name("pi/4 DQPSK System Parameters 5") -> ("PSK type"=w722:u16, "Samples per Symbol"=w724:i32, "Differential PSK"=w723:enum16{"disable", "enable"})
      }
      frame "OQPSK" {
        w730 = 4  # M-PSK (4)
        n11 = Unbundle By Name("OQPSK System Parameters 5") -> ("PSK type"=w727:u16, "Samples per Symbol"=w729:i32, "Differential PSK"=w728:enum16{"disable", "enable"})
      }
      frame "8-PSK" {
        w732 = 8  # M-PSK (4)
        n12 = Unbundle By Name("8-PSK System Parameters 5") -> ("PSK type"=w735:u16, "Samples per Symbol"=w734:i32, "Differential PSK"=w733:enum16{"disable", "enable"})
      }
      frame "16-PSK" {
        w738 = 16  # M-PSK (4)
        n13 = Unbundle By Name("16-PSK System Parameters 5") -> ("PSK type"=w737:u16, "Samples per Symbol"=w740:i32, "Differential PSK"=w739:enum16{"disable", "enable"})
      }
      frame "Custom" {
        n14 = Unbundle By Name("Custom System Parameters 5") -> ("PSK type"=w745:u16, "Samples per Symbol"=w743:i32, "Differential PSK"=w744:enum16{"disable", "enable"})
      }
    }
    n15 = Merge Errors(w22, w21) -> (w20:errorcluster)
    n16 = local write "x .or. y?"(FALSE) -> ()
    n17 = case shown="\"QPSK\"" "Choose a PSK Format" {
      tunnel: [w908 w914 w919 w924 w929 w935 w938] -> w336
      tunnel: [w909 w912 w918 w923 w928 w934 w939] -> w346
      tunnel: [2 ("M-PSK (4)") 4 ("M-PSK (4)") 4 ("M-PSK (4)") 4 ("M-PSK (4)") 8 ("M-PSK (4)") 16 ("M-PSK (4)") "M"] -> w345
      tunnel: [w910 w913 w917 w922 w930 w933 w940] -> w347
      frame "BPSK", Default {
        n18 = Unbundle By Name("BPSK System Parameters") -> ("PSK type"=w910:u16, "Samples per Symbol"=w908:i32, "Differential PSK"=w909:enum16{"disable", "enable"})
      }
      frame "QPSK" {
        n19 = Unbundle By Name("QPSK System Parameters") -> ("PSK type"=w913:u16, "Samples per Symbol"=w914:i32, "Differential PSK"=w912:enum16{"disable", "enable"})
      }
      frame "pi/4DQPSK" {
        n20 = Unbundle By Name("pi/4 DQPSK System Parameters") -> ("PSK type"=w917:u16, "Samples per Symbol"=w919:i32, "Differential PSK"=w918:enum16{"disable", "enable"})
      }
      frame "OQPSK" {
        n21 = Unbundle By Name("OQPSK System Parameters") -> ("PSK type"=w922:u16, "Samples per Symbol"=w924:i32, "Differential PSK"=w923:enum16{"disable", "enable"})
      }
      frame "8-PSK" {
        n22 = Unbundle By Name("8-PSK System Parameters") -> ("PSK type"=w930:u16, "Samples per Symbol"=w929:i32, "Differential PSK"=w928:enum16{"disable", "enable"})
      }
      frame "16-PSK" {
        n23 = Unbundle By Name("16-PSK System Parameters") -> ("PSK type"=w933:u16, "Samples per Symbol"=w935:i32, "Differential PSK"=w934:enum16{"disable", "enable"})
      }
      frame "Custom" {
        n24 = Unbundle By Name("Custom System Parameters") -> ("PSK type"=w940:u16, "Samples per Symbol"=w938:i32, "Differential PSK"=w939:enum16{"disable", "enable"})
      }
    }
    n25 = case shown="\"QPSK\"" "Select PSK Modulation Format" {
      tunnel: [w804 w808 w816 w821 w826 w832 w835] -> w278
      tunnel: [w805 w810 w815 w820 w825 w831 w836] -> w314
      tunnel: [w807 w812 w817 w822 w824 w830 "M 2"] -> w297
      tunnel: [w806 w811 w814 w819 w827 w829 w837] -> w285
      frame "BPSK", Default {
        w807 = 2  # M-PSK
        n26 = Unbundle By Name("BPSK System Parameters 2") -> ("PSK type"=w806:u16, "Samples per Symbol"=w804:i32, "Differential PSK"=w805:enum16{"disable", "enable"})
      }
      frame "QPSK" {
        w812 = 4  # M-PSK (4)
        n27 = Unbundle By Name("QPSK System Parameters 2") -> ("PSK type"=w811:u16, "Samples per Symbol"=w808:i32, "Differential PSK"=w810:enum16{"disable", "enable"})
      }
      frame "pi/4DQPSK" {
        w817 = 4  # M-PSK (4)
        n28 = Unbundle By Name("pi/4 DQPSK System Parameters 2") -> ("PSK type"=w814:u16, "Samples per Symbol"=w816:i32, "Differential PSK"=w815:enum16{"disable", "enable"})
      }
      frame "OQPSK" {
        w822 = 4  # M-PSK (4)
        n29 = Unbundle By Name("OQPSK System Parameters 2") -> ("PSK type"=w819:u16, "Samples per Symbol"=w821:i32, "Differential PSK"=w820:enum16{"disable", "enable"})
      }
      frame "8-PSK" {
        w824 = 8  # M-PSK (4)
        n30 = Unbundle By Name("8-PSK System Parameters 2") -> ("PSK type"=w827:u16, "Samples per Symbol"=w826:i32, "Differential PSK"=w825:enum16{"disable", "enable"})
      }
      frame "16-PSK" {
        w830 = 16  # M-PSK (4)
        n31 = Unbundle By Name("16-PSK System Parameters 2") -> ("PSK type"=w829:u16, "Samples per Symbol"=w832:i32, "Differential PSK"=w831:enum16{"disable", "enable"})
      }
      frame "Custom" {
        n32 = Unbundle By Name("Custom System Parameters 2") -> ("PSK type"=w837:u16, "Samples per Symbol"=w835:i32, "Differential PSK"=w836:enum16{"disable", "enable"})
      }
    }
    n33 = call <instrlib>:"niUSRP Open Tx Session.vi"("device names"=refnum<k15> "USRP1", "reset"=TRUE) -> ("session handle out"=w244:refnum<k15>, "error out"=w243:errorcluster)  [unwired: 12 in]
    n34 = Unbundle By Name("Packet Parameters") -> ("Sync Bits"=w323:i32, "Number of Packets \nto Expect"=w338:i32, "Message Bits"=w337:i32)
    n35 = call "subCallConfigTx.vi"("session handle"=w244, "Tx Parameters"="Tx Parameters 3", "error in"=w243) -> ("session handle out"=w252:refnum<k15>, "Actual Tx Parameters"=w251:T11, "error out"=w231:errorcluster)  [unwired: 10 in]
    "Actual Tx Parameters 3" <- w251
    n36 = call <instrlib>:"niUSRP Open Rx Session.vi"("device names"=refnum<k15> "USRP3", "error in (no error)"=w20) -> ("session handle out"=w357:refnum<k15>, "error out"=w358:errorcluster)  [unwired: 12 in]
    n37 = Unbundle By Name(w251) -> ("Tx IQ Sampling\nRate [s/sec]"=w235:dbl)
    n38 = call "subCallConfigRx.vi"("session handle"=w357, "Rx Parameters"="Rx Parameters", "error in"=w358) -> ("session handle out"=w355:refnum<k15>, "Actual Rx Parameters"=w340:T3, "error out"=w354:errorcluster)  [unwired: 10 in]
    "Actual Rx Parameters" <- w340
    n39 = Unbundle By Name(w340) -> ("Rx IQ Sampling\nRate [s/sec]"=w333:dbl)
    n40 = call <instrlib>:"niUSRP Open Tx Session.vi"("device names"=refnum<k15> "USRP4", "reset"=TRUE) -> ("session handle out"=w288:refnum<k15>, "error out"=w287:errorcluster)  [unwired: 12 in]
    n41 = case shown="\"QPSK\"" "Choose a PSK Format 4" {
      tunnel: [w650 w656 w661 w666 w671 w677 w680] -> w205
      tunnel: [w651 w654 w660 w665 w670 w676 w681] -> w215
      tunnel: [2 ("M-PSK (4)") 4 ("M-PSK (4)") 4 ("M-PSK (4)") 4 ("M-PSK (4)") 8 ("M-PSK (4)") 16 ("M-PSK (4)") "M 7"] -> w214
      tunnel: [w652 w655 w659 w664 w672 w675 w682] -> w216
      frame "BPSK", Default {
        n42 = Unbundle By Name("BPSK System Parameters 7") -> ("PSK type"=w652:u16, "Samples per Symbol"=w650:i32, "Differential PSK"=w651:enum16{"disable", "enable"})
      }
      frame "QPSK" {
        n43 = Unbundle By Name("QPSK System Parameters 7") -> ("PSK type"=w655:u16, "Samples per Symbol"=w656:i32, "Differential PSK"=w654:enum16{"disable", "enable"})
      }
      frame "pi/4DQPSK" {
        n44 = Unbundle By Name("pi/4 DQPSK System Parameters 7") -> ("PSK type"=w659:u16, "Samples per Symbol"=w661:i32, "Differential PSK"=w660:enum16{"disable", "enable"})
      }
      frame "OQPSK" {
        n45 = Unbundle By Name("OQPSK System Parameters 7") -> ("PSK type"=w664:u16, "Samples per Symbol"=w666:i32, "Differential PSK"=w665:enum16{"disable", "enable"})
      }
      frame "8-PSK" {
        n46 = Unbundle By Name("8-PSK System Parameters 7") -> ("PSK type"=w672:u16, "Samples per Symbol"=w671:i32, "Differential PSK"=w670:enum16{"disable", "enable"})
      }
      frame "16-PSK" {
        n47 = Unbundle By Name("16-PSK System Parameters 7") -> ("PSK type"=w675:u16, "Samples per Symbol"=w677:i32, "Differential PSK"=w676:enum16{"disable", "enable"})
      }
      frame "Custom" {
        n48 = Unbundle By Name("Custom System Parameters 7") -> ("PSK type"=w682:u16, "Samples per Symbol"=w680:i32, "Differential PSK"=w681:enum16{"disable", "enable"})
      }
    }
    n49 = call <instrlib>:"niUSRP Initiate.vi"("session handle"=w355, "error in (no error)"=w354) -> ("session handle out"=w319:refnum<k15>, "error out"=w318:errorcluster)  [unwired: 12 in]
    n50 = call "subCallConfigTx.vi"("session handle"=w288, "Tx Parameters"="Tx Parameters", "error in"=w287) -> ("session handle out"=w296:refnum<k15>, "Actual Tx Parameters"=w295:T11, "error out"=w275:errorcluster)  [unwired: 10 in]
    "Actual Tx Parameters" <- w295
    n51 = Bundle("PSK type"=w347, "Samples per Symbol"=w336, "Differential PSK"=w346, "M"=w345) -> (w343:T15)  [unwired: 1 in]
    n52 = Unbundle By Name("Packet Parameters 7") -> ("Sync Bits"=w192:i32, "Number of Packets \nto Expect"=w207:i32, "Message Bits"=w206:i32)
    n53 = Multiply(x="Acquisition Duration [sec]", y=w333) -> (x*y=w360:dbl)
    n54 = call-poly <vilib>:"MT Generate System Parameters.vi"("samples per symbol (16)"=w234, "PSK type"=w241, "M-PSK (4)"=w253, "differential PSK"=w270) -> ("PSK system parameters"=w242:T16)  [unwired: 9 in, 2 out]
    n55 = To Long Integer(number=w360) -> (32bit integer=w317:i32)
    n56 = call <instrlib>:"niUSRP Open Rx Session.vi"("device names"=refnum<k15> "USRP2", "error in (no error)"=w20) -> ("session handle out"=w226:refnum<k15>, "error out"=w227:errorcluster)  [unwired: 12 in]
    n57 = Unbundle By Name(w295) -> ("Tx IQ Sampling\nRate [s/sec]"=w279:dbl)
    n58 = call "sub_Init_PSK_At_Rx.vi"("Sync Bits"=w323, "synchronization parameters"="synchronization parameters", "filter parameters"="filter parameters", "PN sequence order (9)"="PN Sequence Order\nfor Sync", "PSK Parameters"=w343) -> ("PSK Init Parameters"=w342:T17)  [unwired: 5 in, 1 out]
    n59 = call "subGeneratePackets.vi"("Samples per Symbol"=w234, "Packet Pad \n[samples]"="Packet Pad \n[samples] 3", "PSK system parameters"=w242, "Tx IQ Sampling\nRate [s/sec]"=w235, "Pulse Shaping Filter Parameters"="Pulse Shaping Filter Parameters 3", "Packet Repeat"="Packet Repeat 3", "PN sequence order\nfor Sync Bits"="PN sequence order\nfor Sync Bits 3", "Packet Parameters"="Packet Parameters 5", "Message Text"=w33) -> ("Number of Packets"=w250:i32, "Packets"=w258:cluster{"t0":dbl, "dt":dbl, "Y":cdb[]}[], "Symbol Rate"=→"Symbol Rate\n[symbols/sec] 5":dbl)  [unwired: 4 in]
    "Number of Packets in Message 3" <- w250
    n60 = Divide(x=w333, y=w336) -> (x/y=→"Symbol Rate\n[symbols/sec]":dbl)
    n61 = Initialize Array(cdb 0.0+0.0i ("element"), w317) -> (w324:cdb[])
    n62 = Add(x=w339, y=w323) -> (x+y=w348:i32)
    n63 = call-poly <instrlib>:"niUSRP Fetch Rx Data (poly).vi"("session handle"=w319, "number of samples"=w317, "error in (no error)"=w318) -> ("session handle out"=w321:refnum<k15>, "data"=w316:cluster{"t0":dbl, "dt":dbl, "Y":cdb[]}, "error out"=w320:errorcluster)  [unwired: 9 in, 1 out]
    n64 = call "subCallConfigRx.vi"("session handle"=w226, "Rx Parameters"="Rx Parameters 4", "error in"=w227) -> ("session handle out"=w224:refnum<k15>, "Actual Rx Parameters"=w209:T3, "error out"=w223:errorcluster)  [unwired: 10 in]
    "Actual Rx Parameters  4" <- w209
    n65 = Initialize Array(FALSE, w338) -> (w326:bool[])
    n66 = Initialize Array(0, w338, w337) -> (w327:i32[][])
    n67 = Reciprocal(x=w235) -> (1/x=w254:dbl)
    n68 = Bundle(cluster=T12 {"Packet Array"=[], "IP Array of Pkt Nums Received  "=[]} ("Packet Info"), "Packet Array"=w327, "IP Array of Pkt Nums Received"=w326) -> (w325:T12)
    n69 = Unbundle By Name(w209) -> ("Rx IQ Sampling\nRate [s/sec]"=w202:dbl)
    n70 = Bundle("s? t:f"=cluster{"t0":dbl, "dt":dbl, "Y":cdb[]} {"t0"=0.0, "dt"=0.0, "Y"=[]}, 0) -> (w261:T18)  [unwired: 1 in]
    n71 = while {
      tunnel: w333 -> [w905]
      tunnel: w321 -> [w892]
      tunnel: [w890] -> w351
      tunnel: w317 -> [w889]
      tunnel: "Packet Parameters" -> [w904]
      tunnel: w348 -> [w877]
      tunnel: w342 -> [w870]
      shift-right: [w891] -> w272
      shift-left: w320 -> [w887]
      tunnel: w336 -> [w871]
      shift-right: [w875] -> _
      shift-left: w325 -> [w878]
      shift-right: [w884] -> _
      shift-left: T14 {"packet_arr"=[], "Packets Valid?"=FALSE} -> [w885]
      shift-right: [w880] -> _
      shift-left: cluster{"bit stream":i8[][], "Enable?":bool} {"bit stream"=[], "Enable?"=FALSE} ("Output Bitstream") -> [w883]
      shift-right: [w869] -> _
      shift-left: T13 {"bit stream "=[], "Sync Valid?"=[], "Decoded Pkt Numbers"=[], "Enable?"=FALSE} ("Output Bit Stream") -> [w879]
      shift-right: [w881] -> _
      shift-left: w316 -> [w882]
      shift-right: [w872] -> _
      shift-left: w324 -> [w873]
      tunnel: [w867] -> w6
      stop <- w868 stop-if-true
      n72 = call "sub_Reconstruct Data Message.vi"("Start Loc of Data"=w877, "Packet Info"=w878, "Input Stream"=w879) -> ("Packet Info out"=w875:T12)  [unwired: 8 in]
      n73 = call-poly <instrlib>:"niUSRP Fetch Rx Data (poly).vi"("session handle"=w892, "number of samples"=w889, "error in (no error)"=w887) -> ("session handle out"=w890:refnum<k15>, "data"=w881:cluster{"t0":dbl, "dt":dbl, "Y":cdb[]}, "error out"=w891:errorcluster)  [unwired: 9 in, 1 out]
      n74 = Unbundle By Name(w887) -> ("status"=w886:bool)
      n75 = Unbundle By Name(w875) -> ("Packet Array"=w876:i32[][], "IP Array of Pkt Nums Received"=w874:bool[])
      n76 = First Call?() -> (First Call?: T/F=w895:bool)
      n77 = call "sub_Check_Rx_Packet_Validity.vi"("PSK Init Parameters"=w870, "Packet Parameters"=w904, "Input Bit Stream"=w883) -> ("Output Bit Stream"=w869:T13)  [unwired: 7 in]
      n78 = Not(x=w895) -> (.not. x?=w894:bool)
      n79 = call "sub_Resamp_Demod_Shell.vi"("Rx IQ Sampling\nRate [s/sec]"=w905, "PSK Init Parameters"=w870, "Input Packets"=w885) -> ("Synch Found?"=→"Sync Found":bool, "recovered complex waveform"=w898:T19[], "Output Bitstream"=w880:cluster{"bit stream":i8[][], "Enable?":bool})  [unwired: 3 in]
      n80 = And Array Elements(Boolean array=w874) -> (logical AND=w888:bool)
      n81 = call "sub_NoiseEst_And_Chop_Shell.vi"("data"=w882, "Enable"=w894) -> ("Singal & Noise Power"=→"Signal and Noise Power Tracking" →"Singal & Noise Power":cluster{"signal_power":dbl, "noise_power":dbl}, "Output Packets"=w884:cluster{"Packets":cdb[][], "Enable?":bool}, "Delay signal (for plotting use only)"=w872:cdb[])  [unwired: 3 in]
      n82 = Boolean To (0,1)(Boolean=w874) -> (0, 1=w903:i16[])
      n83 = Or(x=w888, y=w886) -> (x .or. y?=w868:bool)
      "x .or. y?" <- w868
      n84 = Add Array Elements(numeric array=w903) -> (sum=→"Correct Packets Rx" →"Cumulative Packets Recovered":i16)
      n85 = call "sub_Format Rx Data.vi"("Output Packet Array"=w876) -> ("Received Message"=w867:string)
      "Recovered Message" <- w867
      n86 = local write "x .or. y?"(w868) -> ()
      n87 = Index Array(array=w898, index=1) -> (element=w897:T19)
      n88 = control-ref of="Constellation Graph"() -> (w900:refnum<vi>)
      n89 = call <vilib>:"MT Format Constellation.vi"("waveform"=w897, "constellation reference"=w900, "samples per symbol"=w871) -> ("constellation graph"=→"Constellation Graph":T20)  [unwired: 2 in, 10 out]
      "Received Signal (Raw)" <- w873
    }
    "text" <- w6
    n90 = call-poly <vilib>:"MT Generate System Parameters.vi"("samples per symbol (16)"=w278, "PSK type"=w285, "M-PSK (4)"=w297, "differential PSK"=w314) -> ("PSK system parameters"=w286:T16)  [unwired: 9 in, 2 out]
    n91 = call <instrlib>:"niUSRP Initiate.vi"("session handle"=w224, "error in (no error)"=w223) -> ("session handle out"=w188:refnum<k15>, "error out"=w187:errorcluster)  [unwired: 12 in]
    n92 = Bundle("PSK type"=w216, "Samples per Symbol"=w205, "Differential PSK"=w215, "M 7"=w214) -> (w212:T21)  [unwired: 1 in]
    n93 = Multiply(x="Acquisition Duration [sec] 4", y=w202) -> (x*y=w229:dbl)
    n94 = Obtain Queue(max queue size (-1, unlimited)="Queue Length 3", element data type=w261) -> (queue out=w267:refnum<queue>, error out=w246:errorcluster)  [unwired: 3 in, 1 out]
    n95 = Initialize Array(cdb 0.0+0.0i ("element"), "Blank Frame \n[samples] 3") -> (w266:cdb[])
    n96 = To Long Integer(number=w229) -> (32bit integer=w186:i32)
    n97 = call "subGeneratePackets.vi"("Samples per Symbol"=w278, "Packet Pad \n[samples]"="Packet Pad \n[samples]", "PSK system parameters"=w286, "Tx IQ Sampling\nRate [s/sec]"=w279, "Pulse Shaping Filter Parameters"="Pulse Shaping Filter Parameters", "Packet Repeat"="Packet Repeat", "PN sequence order\nfor Sync Bits"="PN sequence order\nfor Sync Bits", "Packet Parameters"="Packet Parameters 2", "Message Text"=w25) -> ("Number of Packets"=w294:i32, "Packets"=w302:cluster{"t0":dbl, "dt":dbl, "Y":cdb[]}[], "Symbol Rate"=→"Symbol Rate\n[symbols/sec] 2":dbl)  [unwired: 4 in]
    "Number of Packets in Message" <- w294
    n98 = Bundle By Name(cluster=cluster{"t0":dbl, "dt":dbl, "Y":cdb[]} {"t0"=0.0, "dt"=0.0, "Y"=[]} ("s? t:f"), "dt"=w254, "Y"=w266) -> (w265:cluster{"t0":dbl, "dt":dbl, "Y":cdb[]})
    n99 = call "sub_Init_PSK_At_Rx.vi"("Sync Bits"=w192, "synchronization parameters"="synchronization parameters 4", "filter parameters"="filter parameters 4", "PN sequence order (9)"="PN Sequence Order\nfor Sync 4", "PSK Parameters"=w212) -> ("PSK Init Parameters"=w211:T17)  [unwired: 5 in, 1 out]
    n100 = Divide(x=w202, y=w205) -> (x/y=→"Symbol Rate\n[symbols/sec] 7":dbl)
    n101 = while {
      tunnel: w252 -> [w755]
      shift-right: [w752] -> w256
      shift-left: w231 -> [w756]
      tunnel: w267 -> [w764]
      tunnel: w265 -> [w761]
      tunnel: [w760] -> w264
      tunnel: [w754] -> w255
      shift-right: [w750] -> w263
      shift-left: w246 -> [w757]
      stop <- w751 stop-if-true
      n102 = Get Queue Status(queue=w764, error in (no error)=w757) -> (queue out=w759:refnum<queue>, error out=w758:errorcluster, # elements in queue=w763:i32)  [unwired: 1 in, 5 out]
      n103 = Equal To 0?(x=w763) -> (x = 0?=w762:bool)
      n104 = case shown="False" w762 {
        tunnel: w761 -> [_ w774]
        tunnel: [w766 w774] -> w748
        tunnel: [w770 w772] -> w760
        tunnel: [w765 w773] -> w750
        tunnel: w759 -> [w769 w772]
        tunnel: w758 -> [w768 w773]
        frame False {
          n105 = Dequeue Element(queue=w769, error in (no error)=w768) -> (queue out=w770:refnum<queue>, element=w767:T18, error out=w765:errorcluster)  [unwired: 1 in, 1 out]
          n106 = Unbundle(w767) -> ("s? t:f"=w766:cluster{"t0":dbl, "dt":dbl, "Y":cdb[]})  [unwired: 1 out]
        }
        frame True {
          # "Message\nnot Ready\nTx Blank Frame"
          n107 = Wait Until Next ms Multiple(millisecond multiple=u32 0) -> ()  [unwired: 1 out]
        }
      }
      n108 = local read "x .or. y? 6"() -> (w746:bool)
      n109 = call-poly <instrlib>:"niUSRP Write Tx Data (poly).vi"("session handle"=w755, "data"=w748, "end of data?"="stop 3", "error in (no error)"=w756) -> ("session handle out"=w754:refnum<k15>, "error out"=w752:errorcluster)  [unwired: 10 in]
      n110 = Unbundle By Name(w752) -> ("status"=w753:bool)
      n111 = Unbundle By Name(w750) -> ("status"=w749:bool)
      n112 = Compound Arithmetic op=OR(w749, w753, "stop 3", w746) -> (w751:bool)
    }
    n113 = Reciprocal(x=w279) -> (1/x=w298:dbl)
    n114 = Initialize Array(cdb 0.0+0.0i ("element"), w186) -> (w193:cdb[])
    n115 = while {
      tunnel: w267 -> [w701]
      shift-right: [w694] -> _
      shift-left: 0 -> [w690]
      tunnel: w258 -> [w691]
      tunnel: "Queue Length 3" -> [w693]
      tunnel: w250 -> [w692]
      shift-right: [w688] -> _
      shift-left: w246 -> [w696]
      tunnel: w234 -> [w685]
      stop <- w688 stop-if-true
      n116 = Quotient & Remainder(x=w690, y=w692) -> (x-y*floor(x/y)=w689:i32)  [unwired: 1 out]
      n117 = Index Array(array=w691, index=w689) -> (element=w683:cluster{"t0":dbl, "dt":dbl, "Y":cdb[]})
      n118 = Get Queue Status(queue=w701, error in (no error)=w696) -> (queue out=w700:refnum<queue>, error out=w697:errorcluster, # elements in queue=w699:i32)  [unwired: 1 in, 5 out]
      n119 = Less?(x=w699, y=w693) -> (x < y?=w698:bool)
      n120 = Bundle("output complex waveform"=w683, w689) -> (w695:T22)  [unwired: 1 in]
      n121 = case shown="True" w698 {
        tunnel: w697 -> [w702 w710]
        tunnel: w700 -> [_ w709]
        tunnel: [w702 w708] -> w688
        tunnel: w695 -> [_ w707]
        tunnel: w690 -> [w704 w706]
        tunnel: [w704 w705] -> w694
        frame False {
          n122 = Wait Until Next ms Multiple(millisecond multiple=u32 0) -> ()  [unwired: 1 out]
        }
        frame True {
          n123 = Increment(x=w706) -> (x+1=w705:i32)
          n124 = Enqueue Element(queue=w709, element=w707, error in (no error)=w710) -> (error out=w708:errorcluster)  [unwired: 1 in, 2 out]
        }
      }
      n125 = control-ref of="Constellation Graph 5"() -> (w686:refnum<vi>)
      n126 = call <vilib>:"MT Format Constellation.vi"("waveform"=w683, "constellation reference"=w686, "samples per symbol"=w685, "autoscale"="autoscale 3") -> ("constellation graph"=→"Constellation Graph 5":T20)  [unwired: 1 in, 10 out]
    }
    n127 = Add(x=w208, y=w192) -> (x+y=w217:i32)
    n128 = call-poly <instrlib>:"niUSRP Fetch Rx Data (poly).vi"("session handle"=w188, "number of samples"=w186, "error in (no error)"=w187) -> ("session handle out"=w190:refnum<k15>, "data"=w185:cluster{"t0":dbl, "dt":dbl, "Y":cdb[]}, "error out"=w189:errorcluster)  [unwired: 9 in, 1 out]
    n129 = Initialize Array(FALSE, w207) -> (w195:bool[])
    n130 = Initialize Array(0, w207, w206) -> (w196:i32[][])
    n131 = Bundle("s? t:f"=cluster{"t0":dbl, "dt":dbl, "Y":cdb[]} {"t0"=0.0, "dt"=0.0, "Y"=[]}, 0) -> (w305:T18)  [unwired: 1 in]
    n132 = Bundle(cluster=T12 {"Packet Array"=[], "IP Array of Pkt Nums Received  "=[]} ("Packet Info"), "Packet Array"=w196, "IP Array of Pkt Nums Received"=w195) -> (w194:T12)
    n133 = while {
      tunnel: w202 -> [w647]
      tunnel: w190 -> [w634]
      tunnel: [w632] -> w220
      tunnel: w186 -> [w631]
      tunnel: "Packet Parameters 7" -> [w646]
      tunnel: w217 -> [w619]
      tunnel: w211 -> [w612]
      shift-right: [w633] -> w184
      shift-left: w189 -> [w629]
      tunnel: w205 -> [w613]
      shift-right: [w617] -> _
      shift-left: w194 -> [w620]
      shift-right: [w626] -> _
      shift-left: T14 {"packet_arr"=[], "Packets Valid?"=FALSE} -> [w627]
      shift-right: [w622] -> _
      shift-left: cluster{"bit stream":i8[][], "Enable?":bool} {"bit stream"=[], "Enable?"=FALSE} ("Output Bitstream") -> [w625]
      shift-right: [w611] -> _
      shift-left: T13 {"bit stream "=[], "Sync Valid?"=[], "Decoded Pkt Numbers"=[], "Enable?"=FALSE} ("Output Bit Stream") -> [w621]
      shift-right: [w623] -> _
      shift-left: w185 -> [w624]
      shift-right: [w614] -> _
      shift-left: w193 -> [w615]
      tunnel: [w609] -> w5
      stop <- w610 stop-if-true
      n134 = call "sub_Reconstruct Data Message.vi"("Start Loc of Data"=w619, "Packet Info"=w620, "Input Stream"=w621) -> ("Packet Info out"=w617:T12)  [unwired: 8 in]
      n135 = call-poly <instrlib>:"niUSRP Fetch Rx Data (poly).vi"("session handle"=w634, "number of samples"=w631, "error in (no error)"=w629) -> ("session handle out"=w632:refnum<k15>, "data"=w623:cluster{"t0":dbl, "dt":dbl, "Y":cdb[]}, "error out"=w633:errorcluster)  [unwired: 9 in, 1 out]
      n136 = Unbundle By Name(w629) -> ("status"=w628:bool)
      n137 = Unbundle By Name(w617) -> ("Packet Array"=w618:i32[][], "IP Array of Pkt Nums Received"=w616:bool[])
      n138 = First Call?() -> (First Call?: T/F=w637:bool)
      n139 = call "sub_Check_Rx_Packet_Validity.vi"("PSK Init Parameters"=w612, "Packet Parameters"=w646, "Input Bit Stream"=w625) -> ("Output Bit Stream"=w611:T13)  [unwired: 7 in]
      n140 = Not(x=w637) -> (.not. x?=w636:bool)
      n141 = call "sub_Resamp_Demod_Shell.vi"("Rx IQ Sampling\nRate [s/sec]"=w647, "PSK Init Parameters"=w612, "Input Packets"=w627) -> ("Synch Found?"=→"Sync Found 4":bool, "recovered complex waveform"=w640:T19[], "Output Bitstream"=w622:cluster{"bit stream":i8[][], "Enable?":bool})  [unwired: 3 in]
      n142 = And Array Elements(Boolean array=w616) -> (logical AND=w630:bool)
      n143 = call "sub_NoiseEst_And_Chop_Shell.vi"("data"=w624, "Enable"=w636) -> ("Singal & Noise Power"=→"Signal and Noise Power Tracking 4" →"Singal & Noise Power 4":cluster{"signal_power":dbl, "noise_power":dbl}, "Output Packets"=w626:cluster{"Packets":cdb[][], "Enable?":bool}, "Delay signal (for plotting use only)"=w614:cdb[])  [unwired: 3 in]
      n144 = Boolean To (0,1)(Boolean=w616) -> (0, 1=w645:i16[])
      n145 = Or(x=w630, y=w628) -> (x .or. y?=w610:bool)
      "x .or. y? 6" <- w610
      n146 = Add Array Elements(numeric array=w645) -> (sum=→"Correct Packets Rx 4" →"Cumulative Packets Recovered 4":i16)
      n147 = call "sub_Format Rx Data.vi"("Output Packet Array"=w618) -> ("Received Message"=w609:string)
      "Recovered Message 4" <- w609
      n148 = local write "x .or. y? 6"(w610) -> ()
      n149 = Index Array(array=w640, index=1) -> (element=w639:T19)
      n150 = control-ref of="Constellation Graph 7"() -> (w642:refnum<vi>)
      n151 = call <vilib>:"MT Format Constellation.vi"("waveform"=w639, "constellation reference"=w642, "samples per symbol"=w613) -> ("constellation graph"=→"Constellation Graph 7":T20)  [unwired: 2 in, 10 out]
      "Received Signal (Raw) 4" <- w615
    }
    "text 2" <- w5
    n152 = Obtain Queue(max queue size (-1, unlimited)="Queue Length", element data type=w305) -> (queue out=w311:refnum<queue>, error out=w290:errorcluster)  [unwired: 3 in, 1 out]
    n153 = Initialize Array(cdb 0.0+0.0i ("element"), "Blank Frame \n[samples]") -> (w310:cdb[])
    n154 = Bundle By Name(cluster=cluster{"t0":dbl, "dt":dbl, "Y":cdb[]} {"t0"=0.0, "dt"=0.0, "Y"=[]} ("s? t:f"), "dt"=w298, "Y"=w310) -> (w309:cluster{"t0":dbl, "dt":dbl, "Y":cdb[]})
    n155 = while {
      tunnel: w296 -> [w847]
      shift-right: [w844] -> w300
      shift-left: w275 -> [w848]
      tunnel: w311 -> [w856]
      tunnel: w309 -> [w853]
      tunnel: [w852] -> w308
      tunnel: [w846] -> w299
      shift-right: [w842] -> w307
      shift-left: w290 -> [w849]
      stop <- w843 stop-if-true
      n156 = Get Queue Status(queue=w856, error in (no error)=w849) -> (queue out=w851:refnum<queue>, error out=w850:errorcluster, # elements in queue=w855:i32)  [unwired: 1 in, 5 out]
      n157 = Equal To 0?(x=w855) -> (x = 0?=w854:bool)
      n158 = case shown="False" w854 {
        tunnel: w853 -> [_ w866]
        tunnel: [w858 w866] -> w840
        tunnel: [w862 w864] -> w852
        tunnel: [w857 w865] -> w842
        tunnel: w851 -> [w861 w864]
        tunnel: w850 -> [w860 w865]
        frame False {
          n159 = Dequeue Element(queue=w861, error in (no error)=w860) -> (queue out=w862:refnum<queue>, element=w859:T18, error out=w857:errorcluster)  [unwired: 1 in, 1 out]
          n160 = Unbundle(w859) -> ("s? t:f"=w858:cluster{"t0":dbl, "dt":dbl, "Y":cdb[]})  [unwired: 1 out]
        }
        frame True {
          # "Message\nnot Ready\nTx Blank Frame"
          n161 = Wait Until Next ms Multiple(millisecond multiple=u32 0) -> ()  [unwired: 1 out]
        }
      }
      n162 = call-poly <instrlib>:"niUSRP Write Tx Data (poly).vi"("session handle"=w847, "data"=w840, "end of data?"="stop", "error in (no error)"=w848) -> ("session handle out"=w846:refnum<k15>, "error out"=w844:errorcluster)  [unwired: 10 in]
      n163 = local read "x .or. y?"() -> (w838:bool)
      n164 = Unbundle By Name(w844) -> ("status"=w845:bool)
      n165 = Unbundle By Name(w842) -> ("status"=w841:bool)
      n166 = Compound Arithmetic op=OR(w841, w845, "stop", w838) -> (w843:bool)
    }
    n167 = while {
      tunnel: w311 -> [w793]
      shift-right: [w786] -> _
      shift-left: 0 -> [w782]
      tunnel: w302 -> [w783]
      tunnel: "Queue Length" -> [w785]
      tunnel: w294 -> [w784]
      shift-right: [w780] -> _
      shift-left: w290 -> [w788]
      tunnel: w278 -> [w777]
      stop <- w780 stop-if-true
      n168 = Quotient & Remainder(x=w782, y=w784) -> (x-y*floor(x/y)=w781:i32)  [unwired: 1 out]
      n169 = Index Array(array=w783, index=w781) -> (element=w775:cluster{"t0":dbl, "dt":dbl, "Y":cdb[]})
      n170 = Get Queue Status(queue=w793, error in (no error)=w788) -> (queue out=w792:refnum<queue>, error out=w789:errorcluster, # elements in queue=w791:i32)  [unwired: 1 in, 5 out]
      n171 = Less?(x=w791, y=w785) -> (x < y?=w790:bool)
      n172 = Bundle("output complex waveform"=w775, w781) -> (w787:T22)  [unwired: 1 in]
      n173 = case shown="True" w790 {
        tunnel: w789 -> [w794 w802]
        tunnel: w792 -> [_ w801]
        tunnel: [w794 w800] -> w780
        tunnel: w787 -> [_ w799]
        tunnel: w782 -> [w796 w798]
        tunnel: [w796 w797] -> w786
        frame False {
          n174 = Wait Until Next ms Multiple(millisecond multiple=u32 0) -> ()  [unwired: 1 out]
        }
        frame True {
          n175 = Increment(x=w798) -> (x+1=w797:i32)
          n176 = Enqueue Element(queue=w801, element=w799, error in (no error)=w802) -> (error out=w800:errorcluster)  [unwired: 1 in, 2 out]
        }
      }
      n177 = control-ref of="Constellation Graph 2"() -> (w778:refnum<vi>)
      n178 = call <vilib>:"MT Format Constellation.vi"("waveform"=w775, "constellation reference"=w778, "samples per symbol"=w777, "autoscale"="autoscale") -> ("constellation graph"=→"Constellation Graph 2":T20)  [unwired: 1 in, 10 out]
    }
    n179 = call <instrlib>:"niUSRP Abort.vi"("session handle"=w351, "error in (no error)"=w272) -> ("session handle out"=w352:refnum<k15>, "error out"=w353:errorcluster)  [unwired: 12 in]
    n180 = Write to Text File(file (use dialog)="file (use dialog) 2", text=w6) -> ()  [unwired: 2 in, 3 out]
    n181 = call <instrlib>:"niUSRP Close Session.vi"("session handle"=w352, "error in (no error)"=w353) -> ("error out"=w182:errorcluster)  [unwired: 13 in]
    "error out" <- w182
    n182 = Release Queue(queue=w264, error in (no error)=w263) -> (error out=w240:errorcluster)  [unwired: 3 out]
    n183 = call <instrlib>:"niUSRP Close Session.vi"("session handle"=w255, "error in (no error)"=w256) -> ("error out"=w239:errorcluster)  [unwired: 13 in]
    n184 = Merge Errors(w240, w239) -> (w179:errorcluster)
    "error out 5" <- w179
    n185 = call <instrlib>:"niUSRP Abort.vi"("session handle"=w220, "error in (no error)"=w184) -> ("session handle out"=w221:refnum<k15>, "error out"=w222:errorcluster)  [unwired: 12 in]
    n186 = call <instrlib>:"niUSRP Close Session.vi"("session handle"=w221, "error in (no error)"=w222) -> ("error out"=w183:errorcluster)  [unwired: 13 in]
    "error out 7" <- w183
    n187 = Merge Errors "Merge Errors"(w182, w183) -> (w136:errorcluster)
    n188 = Release Queue(queue=w308, error in (no error)=w307) -> (error out=w284:errorcluster)  [unwired: 3 out]
    n189 = call <instrlib>:"niUSRP Close Session.vi"("session handle"=w299, "error in (no error)"=w300) -> ("error out"=w283:errorcluster)  [unwired: 13 in]
    n190 = Write to Text File(file (use dialog)="file (use dialog)", text=w5) -> ()  [unwired: 2 in, 3 out]
    n191 = Merge Errors(w284, w283) -> (w178:errorcluster)
    "error out 2" <- w178
    n192 = Merge Errors(w179, w178) -> (w42:errorcluster)
    n193 = while {
      tunnel: w136 -> [w605]
      tunnel: [w605] -> w12
      tunnel: w42 -> [w604]
      tunnel: [w604] -> w13
      stop <- w606 stop-if-true
      n194 = local read "x .or. y? 6"() -> (w607:bool)
      n195 = local read "x .or. y?"() -> (w608:bool)
      n196 = And(x=w608, y=w607) -> (x .and. y?=w606:bool)
    }
    n197 = case shown="\"QPSK\"" "Choose a PSK Format 3" {
      tunnel: [w403 w409 w414 w419 w424 w430 w433] -> w64
      tunnel: [w404 w407 w413 w418 w423 w429 w434] -> w74
      tunnel: [2 ("M-PSK (4)") 4 ("M-PSK (4)") 4 ("M-PSK (4)") 4 ("M-PSK (4)") 8 ("M-PSK (4)") 16 ("M-PSK (4)") "M 6"] -> w73
      tunnel: [w405 w408 w412 w417 w425 w428 w435] -> w75
      frame "BPSK", Default {
        n198 = Unbundle By Name("BPSK System Parameters 6") -> ("PSK type"=w405:u16, "Samples per Symbol"=w403:i32, "Differential PSK"=w404:enum16{"disable", "enable"})
      }
      frame "QPSK" {
        n199 = Unbundle By Name("QPSK System Parameters 6") -> ("PSK type"=w408:u16, "Samples per Symbol"=w409:i32, "Differential PSK"=w407:enum16{"disable", "enable"})
      }
      frame "pi/4DQPSK" {
        n200 = Unbundle By Name("pi/4 DQPSK System Parameters 6") -> ("PSK type"=w412:u16, "Samples per Symbol"=w414:i32, "Differential PSK"=w413:enum16{"disable", "enable"})
      }
      frame "OQPSK" {
        n201 = Unbundle By Name("OQPSK System Parameters 6") -> ("PSK type"=w417:u16, "Samples per Symbol"=w419:i32, "Differential PSK"=w418:enum16{"disable", "enable"})
      }
      frame "8-PSK" {
        n202 = Unbundle By Name("8-PSK System Parameters 6") -> ("PSK type"=w425:u16, "Samples per Symbol"=w424:i32, "Differential PSK"=w423:enum16{"disable", "enable"})
      }
      frame "16-PSK" {
        n203 = Unbundle By Name("16-PSK System Parameters 6") -> ("PSK type"=w428:u16, "Samples per Symbol"=w430:i32, "Differential PSK"=w429:enum16{"disable", "enable"})
      }
      frame "Custom" {
        n204 = Unbundle By Name("Custom System Parameters 6") -> ("PSK type"=w435:u16, "Samples per Symbol"=w433:i32, "Differential PSK"=w434:enum16{"disable", "enable"})
      }
    }
    n205 = Unbundle By Name("Packet Parameters 6") -> ("Sync Bits"=w51:i32, "Number of Packets \nto Expect"=w66:i32, "Message Bits"=w65:i32)
    n206 = case shown="\"QPSK\"" "Select PSK Modulation Format 2" {
      tunnel: [w539 w543 w551 w556 w561 w567 w570] -> w139
      tunnel: [w540 w545 w550 w555 w560 w566 w571] -> w176
      tunnel: [w542 w547 w552 w557 w559 w565 "M 4"] -> w159
      tunnel: [w541 w546 w549 w554 w562 w564 w572] -> w146
      frame "BPSK", Default {
        w542 = 2  # M-PSK
        n207 = Unbundle By Name("BPSK System Parameters 4") -> ("PSK type"=w541:u16, "Samples per Symbol"=w539:i32, "Differential PSK"=w540:enum16{"disable", "enable"})
      }
      frame "QPSK" {
        w547 = 4  # M-PSK (4)
        n208 = Unbundle By Name("QPSK System Parameters 4") -> ("PSK type"=w546:u16, "Samples per Symbol"=w543:i32, "Differential PSK"=w545:enum16{"disable", "enable"})
      }
      frame "pi/4DQPSK" {
        w552 = 4  # M-PSK (4)
        n209 = Unbundle By Name("pi/4 DQPSK System Parameters 4") -> ("PSK type"=w549:u16, "Samples per Symbol"=w551:i32, "Differential PSK"=w550:enum16{"disable", "enable"})
      }
      frame "OQPSK" {
        w557 = 4  # M-PSK (4)
        n210 = Unbundle By Name("OQPSK System Parameters 4") -> ("PSK type"=w554:u16, "Samples per Symbol"=w556:i32, "Differential PSK"=w555:enum16{"disable", "enable"})
      }
      frame "8-PSK" {
        w559 = 8  # M-PSK (4)
        n211 = Unbundle By Name("8-PSK System Parameters 4") -> ("PSK type"=w562:u16, "Samples per Symbol"=w561:i32, "Differential PSK"=w560:enum16{"disable", "enable"})
      }
      frame "16-PSK" {
        w565 = 16  # M-PSK (4)
        n212 = Unbundle By Name("16-PSK System Parameters 4") -> ("PSK type"=w564:u16, "Samples per Symbol"=w567:i32, "Differential PSK"=w566:enum16{"disable", "enable"})
      }
      frame "Custom" {
        n213 = Unbundle By Name("Custom System Parameters 4") -> ("PSK type"=w572:u16, "Samples per Symbol"=w570:i32, "Differential PSK"=w571:enum16{"disable", "enable"})
      }
    }
    n214 = Merge Errors(w13, w12) -> (w11:errorcluster)
    n215 = call <vilib>:"System Exec.vi"("wait until completion? (T)"=TRUE, "error in (no error)"=w11, "command line"="py avg.py") -> ("error out"=w4:errorcluster, "standard error"=→"standard error 3":string, "standard output"=w14:string)  [unwired: 5 in, 1 out]
    "standard output 3" <- w14
    n216 = case shown="\"QPSK\"" "Choose a PSK Format 2" {
      tunnel: [w477 w483 w488 w493 w498 w504 w507] -> w110
      tunnel: [w478 w481 w487 w492 w497 w503 w508] -> w120
      tunnel: [2 ("M-PSK (4)") 4 ("M-PSK (4)") 4 ("M-PSK (4)") 4 ("M-PSK (4)") 8 ("M-PSK (4)") 16 ("M-PSK (4)") "M 3"] -> w119
      tunnel: [w479 w482 w486 w491 w499 w502 w509] -> w121
      frame "BPSK", Default {
        n217 = Unbundle By Name("BPSK System Parameters 3") -> ("PSK type"=w479:u16, "Samples per Symbol"=w477:i32, "Differential PSK"=w478:enum16{"disable", "enable"})
      }
      frame "QPSK" {
        n218 = Unbundle By Name("QPSK System Parameters 3") -> ("PSK type"=w482:u16, "Samples per Symbol"=w483:i32, "Differential PSK"=w481:enum16{"disable", "enable"})
      }
      frame "pi/4DQPSK" {
        n219 = Unbundle By Name("pi/4 DQPSK System Parameters 3") -> ("PSK type"=w486:u16, "Samples per Symbol"=w488:i32, "Differential PSK"=w487:enum16{"disable", "enable"})
      }
      frame "OQPSK" {
        n220 = Unbundle By Name("OQPSK System Parameters 3") -> ("PSK type"=w491:u16, "Samples per Symbol"=w493:i32, "Differential PSK"=w492:enum16{"disable", "enable"})
      }
      frame "8-PSK" {
        n221 = Unbundle By Name("8-PSK System Parameters 3") -> ("PSK type"=w499:u16, "Samples per Symbol"=w498:i32, "Differential PSK"=w497:enum16{"disable", "enable"})
      }
      frame "16-PSK" {
        n222 = Unbundle By Name("16-PSK System Parameters 3") -> ("PSK type"=w502:u16, "Samples per Symbol"=w504:i32, "Differential PSK"=w503:enum16{"disable", "enable"})
      }
      frame "Custom" {
        n223 = Unbundle By Name("Custom System Parameters 3") -> ("PSK type"=w509:u16, "Samples per Symbol"=w507:i32, "Differential PSK"=w508:enum16{"disable", "enable"})
      }
    }
    n224 = Unbundle By Name("Packet Parameters 3") -> ("Sync Bits"=w97:i32, "Number of Packets \nto Expect"=w112:i32, "Message Bits"=w111:i32)
    n225 = Bundle("PSK type"=w75, "Samples per Symbol"=w64, "Differential PSK"=w74, "M 6"=w73) -> (w71:T23)  [unwired: 1 in]
    n226 = call <instrlib>:"niUSRP Open Tx Session.vi"("device names"=refnum<k15> "USRP2", "reset"=TRUE, "error in (no error)"=w4) -> ("session handle out"=w150:refnum<k15>, "error out"=w149:errorcluster)  [unwired: 11 in]
    n227 = call "subCallConfigTx.vi"("session handle"=w150, "Tx Parameters"="Tx Parameters 2", "error in"=w149) -> ("session handle out"=w158:refnum<k15>, "Actual Tx Parameters"=w157:T11, "error out"=w3:errorcluster)  [unwired: 10 in]
    "Actual Tx Parameters 2" <- w157
    n228 = call <instrlib>:"niUSRP Open Rx Session.vi"("device names"=refnum<k15> "USRP3", "reset"=TRUE, "error in (no error)"=w3) -> ("session handle out"=w84:refnum<k15>, "error out"=w85:errorcluster)  [unwired: 11 in]
    n229 = call "subCallConfigRx.vi"("session handle"=w84, "Rx Parameters"="Rx Parameters 3", "error in"=w85) -> ("session handle out"=w82:refnum<k15>, "Actual Rx Parameters"=w68:T3, "error out"=w81:errorcluster)  [unwired: 10 in]
    "Actual Rx Parameters  3" <- w68
    n230 = Unbundle By Name(w68) -> ("Rx IQ Sampling\nRate [s/sec]"=w61:dbl)
    n231 = call <instrlib>:"niUSRP Initiate.vi"("session handle"=w82, "error in (no error)"=w81) -> ("session handle out"=w47:refnum<k15>, "error out"=w46:errorcluster)  [unwired: 12 in]
    n232 = call <instrlib>:"niUSRP Open Rx Session.vi"("device names"=refnum<k15> "USRP4", "error in (no error)"=w3) -> ("session handle out"=w131:refnum<k15>, "error out"=w132:errorcluster)  [unwired: 12 in]
    n233 = Multiply(x="Acquisition Duration [sec] 3", y=w61) -> (x*y=w87:dbl)
    n234 = To Long Integer(number=w87) -> (32bit integer=w45:i32)
    n235 = call "sub_Init_PSK_At_Rx.vi"("Sync Bits"=w51, "synchronization parameters"="synchronization parameters 3", "filter parameters"="filter parameters 3", "PN sequence order (9)"="PN Sequence Order\nfor Sync 3", "PSK Parameters"=w71) -> ("PSK Init Parameters"=w70:T17)  [unwired: 5 in, 1 out]
    n236 = Divide(x=w61, y=w64) -> (x/y=→"Symbol Rate\n[symbols/sec] 6":dbl)
    n237 = call "subCallConfigRx.vi"("session handle"=w131, "Rx Parameters"="Rx Parameters 2", "error in"=w132) -> ("session handle out"=w129:refnum<k15>, "Actual Rx Parameters"=w114:T3, "error out"=w128:errorcluster)  [unwired: 10 in]
    "Actual Rx Parameters  2" <- w114
    n238 = Initialize Array(cdb 0.0+0.0i ("element"), w45) -> (w52:cdb[])
    n239 = Add(x=w67, y=w51) -> (x+y=w76:i32)
    n240 = Unbundle By Name(w157) -> ("Tx IQ Sampling\nRate [s/sec]"=w140:dbl)
    n241 = call-poly <instrlib>:"niUSRP Fetch Rx Data (poly).vi"("session handle"=w47, "number of samples"=w45, "error in (no error)"=w46) -> ("session handle out"=w49:refnum<k15>, "data"=w44:cluster{"t0":dbl, "dt":dbl, "Y":cdb[]}, "error out"=w48:errorcluster)  [unwired: 9 in, 1 out]
    n242 = Initialize Array(FALSE, w66) -> (w54:bool[])
    n243 = Initialize Array(0, w66, w65) -> (w55:i32[][])
    n244 = Unbundle By Name(w114) -> ("Rx IQ Sampling\nRate [s/sec]"=w107:dbl)
    n245 = Bundle(cluster=T12 {"Packet Array"=[], "IP Array of Pkt Nums Received  "=[]} ("Packet Info"), "Packet Array"=w55, "IP Array of Pkt Nums Received"=w54) -> (w53:T12)
    n246 = call <instrlib>:"niUSRP Initiate.vi"("session handle"=w129, "error in (no error)"=w128) -> ("session handle out"=w93:refnum<k15>, "error out"=w92:errorcluster)  [unwired: 12 in]
    n247 = Bundle("PSK type"=w121, "Samples per Symbol"=w110, "Differential PSK"=w120, "M 3"=w119) -> (w117:T24)  [unwired: 1 in]
    n248 = Multiply(x="Acquisition Duration [sec] 2", y=w107) -> (x*y=w134:dbl)
    n249 = while {
      tunnel: w61 -> [w400]
      tunnel: w49 -> [w387]
      tunnel: [w385] -> w79
      tunnel: w45 -> [w384]
      tunnel: "Packet Parameters 6" -> [w399]
      tunnel: w76 -> [w372]
      tunnel: w70 -> [w365]
      shift-right: [w386] -> w43
      shift-left: w48 -> [w382]
      tunnel: w64 -> [w366]
      shift-right: [w370] -> _
      shift-left: w53 -> [w373]
      shift-right: [w379] -> _
      shift-left: T14 {"packet_arr"=[], "Packets Valid?"=FALSE} -> [w380]
      shift-right: [w375] -> _
      shift-left: cluster{"bit stream":i8[][], "Enable?":bool} {"bit stream"=[], "Enable?"=FALSE} ("Output Bitstream") -> [w378]
      shift-right: [w364] -> _
      shift-left: T13 {"bit stream "=[], "Sync Valid?"=[], "Decoded Pkt Numbers"=[], "Enable?"=FALSE} ("Output Bit Stream") -> [w374]
      shift-right: [w376] -> _
      shift-left: w44 -> [w377]
      shift-right: [w367] -> _
      shift-left: w52 -> [w368]
      tunnel: [w362] -> w10
      stop <- w363 stop-if-true
      n250 = call "sub_Reconstruct Data Message.vi"("Start Loc of Data"=w372, "Packet Info"=w373, "Input Stream"=w374) -> ("Packet Info out"=w370:T12)  [unwired: 8 in]
      n251 = call-poly <instrlib>:"niUSRP Fetch Rx Data (poly).vi"("session handle"=w387, "number of samples"=w384, "error in (no error)"=w382) -> ("session handle out"=w385:refnum<k15>, "data"=w376:cluster{"t0":dbl, "dt":dbl, "Y":cdb[]}, "error out"=w386:errorcluster)  [unwired: 9 in, 1 out]
      n252 = Unbundle By Name(w382) -> ("status"=w381:bool)
      n253 = Unbundle By Name(w370) -> ("Packet Array"=w371:i32[][], "IP Array of Pkt Nums Received"=w369:bool[])
      n254 = First Call?() -> (First Call?: T/F=w390:bool)
      n255 = call "sub_Check_Rx_Packet_Validity.vi"("PSK Init Parameters"=w365, "Packet Parameters"=w399, "Input Bit Stream"=w378) -> ("Output Bit Stream"=w364:T13)  [unwired: 7 in]
      n256 = Not(x=w390) -> (.not. x?=w389:bool)
      n257 = call "sub_Resamp_Demod_Shell.vi"("Rx IQ Sampling\nRate [s/sec]"=w400, "PSK Init Parameters"=w365, "Input Packets"=w380) -> ("Synch Found?"=→"Sync Found 3":bool, "recovered complex waveform"=w393:T19[], "Output Bitstream"=w375:cluster{"bit stream":i8[][], "Enable?":bool})  [unwired: 3 in]
      n258 = And Array Elements(Boolean array=w369) -> (logical AND=w383:bool)
      n259 = call "sub_NoiseEst_And_Chop_Shell.vi"("data"=w377, "Enable"=w389) -> ("Singal & Noise Power"=→"Signal and Noise Power Tracking 3" →"Singal & Noise Power 3":cluster{"signal_power":dbl, "noise_power":dbl}, "Output Packets"=w379:cluster{"Packets":cdb[][], "Enable?":bool}, "Delay signal (for plotting use only)"=w367:cdb[])  [unwired: 3 in]
      n260 = Boolean To (0,1)(Boolean=w369) -> (0, 1=w398:i16[])
      n261 = Or(x=w383, y=w381) -> (x .or. y?=w363:bool)
      "x .or. y? 4" <- w363
      n262 = Add Array Elements(numeric array=w398) -> (sum=→"Correct Packets Rx 3" →"Cumulative Packets Recovered 3":i16)
      n263 = call "sub_Format Rx Data.vi"("Output Packet Array"=w371) -> ("Received Message"=w362:string)
      "Recovered Message 3" <- w362
      n264 = local write "x .or. y? 4"(w363) -> ()
      n265 = Index Array(array=w393, index=1) -> (element=w392:T19)
      n266 = control-ref of="Constellation Graph 6"() -> (w395:refnum<vi>)
      n267 = call <vilib>:"MT Format Constellation.vi"("waveform"=w392, "constellation reference"=w395, "samples per symbol"=w366) -> ("constellation graph"=→"Constellation Graph 6":T20)  [unwired: 2 in, 10 out]
      "Received Signal (Raw) 3" <- w368
    }
    n268 = To Long Integer(number=w134) -> (32bit integer=w91:i32)
    n269 = call "sub_Init_PSK_At_Rx.vi"("Sync Bits"=w97, "synchronization parameters"="synchronization parameters 2", "filter parameters"="filter parameters 2", "PN sequence order (9)"="PN Sequence Order\nfor Sync 2", "PSK Parameters"=w117) -> ("PSK Init Parameters"=w116:T17)  [unwired: 5 in, 1 out]
    n270 = Divide(x=w107, y=w110) -> (x/y=→"Symbol Rate\n[symbols/sec] 3":dbl)
    n271 = call-poly <vilib>:"MT Generate System Parameters.vi"("samples per symbol (16)"=w139, "PSK type"=w146, "M-PSK (4)"=w159, "differential PSK"=w176) -> ("PSK system parameters"=w147:T16)  [unwired: 9 in, 2 out]
    n272 = Initialize Array(cdb 0.0+0.0i ("element"), w91) -> (w98:cdb[])
    n273 = Add(x=w113, y=w97) -> (x+y=w122:i32)
    n274 = call-poly <instrlib>:"niUSRP Fetch Rx Data (poly).vi"("session handle"=w93, "number of samples"=w91, "error in (no error)"=w92) -> ("session handle out"=w95:refnum<k15>, "data"=w90:cluster{"t0":dbl, "dt":dbl, "Y":cdb[]}, "error out"=w94:errorcluster)  [unwired: 9 in, 1 out]
    n275 = Initialize Array(FALSE, w112) -> (w100:bool[])
    n276 = Initialize Array(0, w112, w111) -> (w101:i32[][])
    n277 = call "subGeneratePackets.vi"("Samples per Symbol"=w139, "Packet Pad \n[samples]"="Packet Pad \n[samples] 2", "PSK system parameters"=w147, "Tx IQ Sampling\nRate [s/sec]"=w140, "Pulse Shaping Filter Parameters"="Pulse Shaping Filter Parameters 2", "Packet Repeat"="Packet Repeat 2", "PN sequence order\nfor Sync Bits"="PN sequence order\nfor Sync Bits 2", "Packet Parameters"="Packet Parameters 4", "Message Text"=w14) -> ("Number of Packets"=w156:i32, "Packets"=w164:cluster{"t0":dbl, "dt":dbl, "Y":cdb[]}[], "Symbol Rate"=→"Symbol Rate\n[symbols/sec] 4":dbl)  [unwired: 4 in]
    "Number of Packets in Message 2" <- w156
    n278 = Bundle(cluster=T12 {"Packet Array"=[], "IP Array of Pkt Nums Received  "=[]} ("Packet Info"), "Packet Array"=w101, "IP Array of Pkt Nums Received"=w100) -> (w99:T12)
    n279 = Reciprocal(x=w140) -> (1/x=w160:dbl)
    n280 = while {
      tunnel: w107 -> [w474]
      tunnel: w95 -> [w461]
      tunnel: [w459] -> w125
      tunnel: w91 -> [w458]
      tunnel: "Packet Parameters 3" -> [w473]
      tunnel: w122 -> [w446]
      tunnel: w116 -> [w439]
      shift-right: [w460] -> w89
      shift-left: w94 -> [w456]
      tunnel: w110 -> [w440]
      shift-right: [w444] -> _
      shift-left: w99 -> [w447]
      shift-right: [w453] -> _
      shift-left: T14 {"packet_arr"=[], "Packets Valid?"=FALSE} -> [w454]
      shift-right: [w449] -> _
      shift-left: cluster{"bit stream":i8[][], "Enable?":bool} {"bit stream"=[], "Enable?"=FALSE} ("Output Bitstream") -> [w452]
      shift-right: [w438] -> _
      shift-left: T13 {"bit stream "=[], "Sync Valid?"=[], "Decoded Pkt Numbers"=[], "Enable?"=FALSE} ("Output Bit Stream") -> [w448]
      shift-right: [w450] -> _
      shift-left: w90 -> [w451]
      shift-right: [w441] -> _
      shift-left: w98 -> [w442]
      tunnel: [w436] -> w8
      stop <- w437 stop-if-true
      n281 = call "sub_Reconstruct Data Message.vi"("Start Loc of Data"=w446, "Packet Info"=w447, "Input Stream"=w448) -> ("Packet Info out"=w444:T12)  [unwired: 8 in]
      n282 = call-poly <instrlib>:"niUSRP Fetch Rx Data (poly).vi"("session handle"=w461, "number of samples"=w458, "error in (no error)"=w456) -> ("session handle out"=w459:refnum<k15>, "data"=w450:cluster{"t0":dbl, "dt":dbl, "Y":cdb[]}, "error out"=w460:errorcluster)  [unwired: 9 in, 1 out]
      n283 = Unbundle By Name(w456) -> ("status"=w455:bool)
      n284 = Unbundle By Name(w444) -> ("Packet Array"=w445:i32[][], "IP Array of Pkt Nums Received"=w443:bool[])
      n285 = First Call?() -> (First Call?: T/F=w464:bool)
      n286 = call "sub_Check_Rx_Packet_Validity.vi"("PSK Init Parameters"=w439, "Packet Parameters"=w473, "Input Bit Stream"=w452) -> ("Output Bit Stream"=w438:T13)  [unwired: 7 in]
      n287 = Not(x=w464) -> (.not. x?=w463:bool)
      n288 = call "sub_Resamp_Demod_Shell.vi"("Rx IQ Sampling\nRate [s/sec]"=w474, "PSK Init Parameters"=w439, "Input Packets"=w454) -> ("Synch Found?"=→"Sync Found 2":bool, "recovered complex waveform"=w467:T19[], "Output Bitstream"=w449:cluster{"bit stream":i8[][], "Enable?":bool})  [unwired: 3 in]
      n289 = And Array Elements(Boolean array=w443) -> (logical AND=w457:bool)
      n290 = call "sub_NoiseEst_And_Chop_Shell.vi"("data"=w451, "Enable"=w463) -> ("Singal & Noise Power"=→"Signal and Noise Power Tracking 2" →"Singal & Noise Power 2":cluster{"signal_power":dbl, "noise_power":dbl}, "Output Packets"=w453:cluster{"Packets":cdb[][], "Enable?":bool}, "Delay signal (for plotting use only)"=w441:cdb[])  [unwired: 3 in]
      n291 = Boolean To (0,1)(Boolean=w443) -> (0, 1=w472:i16[])
      n292 = Or(x=w457, y=w455) -> (x .or. y?=w437:bool)
      "x .or. y? 2" <- w437
      n293 = Add Array Elements(numeric array=w472) -> (sum=→"Correct Packets Rx 2" →"Cumulative Packets Recovered 2":i16)
      n294 = call "sub_Format Rx Data.vi"("Output Packet Array"=w445) -> ("Received Message"=w436:string)
      "Recovered Message 2" <- w436
      n295 = local write "x .or. y? 2"(w437) -> ()
      n296 = Index Array(array=w467, index=1) -> (element=w466:T19)
      n297 = control-ref of="Constellation Graph 3"() -> (w469:refnum<vi>)
      n298 = call <vilib>:"MT Format Constellation.vi"("waveform"=w466, "constellation reference"=w469, "samples per symbol"=w440) -> ("constellation graph"=→"Constellation Graph 3":T20)  [unwired: 2 in, 10 out]
      "Received Signal (Raw) 2" <- w442
    }
    n299 = Bundle("s? t:f"=cluster{"t0":dbl, "dt":dbl, "Y":cdb[]} {"t0"=0.0, "dt"=0.0, "Y"=[]}, 0) -> (w167:T18)  [unwired: 1 in]
    n300 = Obtain Queue(max queue size (-1, unlimited)="Queue Length 2", element data type=w167) -> (queue out=w173:refnum<queue>, error out=w152:errorcluster)  [unwired: 3 in, 1 out]
    n301 = Initialize Array(cdb 0.0+0.0i ("element"), "Blank Frame \n[samples] 2") -> (w172:cdb[])
    n302 = Bundle By Name(cluster=cluster{"t0":dbl, "dt":dbl, "Y":cdb[]} {"t0"=0.0, "dt"=0.0, "Y"=[]} ("s? t:f"), "dt"=w160, "Y"=w172) -> (w171:cluster{"t0":dbl, "dt":dbl, "Y":cdb[]})
    n303 = while {
      tunnel: w158 -> [w584]
      shift-right: [w581] -> w162
      shift-left: w3 -> [w585]
      tunnel: w173 -> [w593]
      tunnel: w171 -> [w590]
      tunnel: [w589] -> w170
      tunnel: [w583] -> w161
      shift-right: [w579] -> w169
      shift-left: w152 -> [w586]
      stop <- w580 stop-if-true
      n304 = Get Queue Status(queue=w593, error in (no error)=w586) -> (queue out=w588:refnum<queue>, error out=w587:errorcluster, # elements in queue=w592:i32)  [unwired: 1 in, 5 out]
      n305 = Equal To 0?(x=w592) -> (x = 0?=w591:bool)
      n306 = case shown="False" w591 {
        tunnel: w590 -> [_ w603]
        tunnel: [w595 w603] -> w577
        tunnel: [w599 w601] -> w589
        tunnel: [w594 w602] -> w579
        tunnel: w588 -> [w598 w601]
        tunnel: w587 -> [w597 w602]
        frame False {
          n307 = Dequeue Element(queue=w598, error in (no error)=w597) -> (queue out=w599:refnum<queue>, element=w596:T18, error out=w594:errorcluster)  [unwired: 1 in, 1 out]
          n308 = Unbundle(w596) -> ("s? t:f"=w595:cluster{"t0":dbl, "dt":dbl, "Y":cdb[]})  [unwired: 1 out]
        }
        frame True {
          # "Message\nnot Ready\nTx Blank Frame"
          n309 = Wait Until Next ms Multiple(millisecond multiple=u32 0) -> ()  [unwired: 1 out]
        }
      }
      n310 = local read "x .or. y? 4"() -> (w575:bool)
      n311 = local read "x .or. y? 2"() -> (w574:bool)
      n312 = And(x=w575, y=w574) -> (x .and. y?=w573:bool)
      n313 = call-poly <instrlib>:"niUSRP Write Tx Data (poly).vi"("session handle"=w584, "data"=w577, "end of data?"="stop 2", "error in (no error)"=w585) -> ("session handle out"=w583:refnum<k15>, "error out"=w581:errorcluster)  [unwired: 10 in]
      n314 = Unbundle By Name(w581) -> ("status"=w582:bool)
      n315 = Unbundle By Name(w579) -> ("status"=w578:bool)
      n316 = Compound Arithmetic op=OR(w578, w582, "stop 2", w573) -> (w580:bool)
    }
    n317 = while {
      tunnel: w173 -> [w528]
      shift-right: [w521] -> _
      shift-left: 0 -> [w517]
      tunnel: w164 -> [w518]
      tunnel: "Queue Length 2" -> [w520]
      tunnel: w156 -> [w519]
      shift-right: [w515] -> _
      shift-left: w152 -> [w523]
      tunnel: w139 -> [w512]
      stop <- w515 stop-if-true
      n318 = Quotient & Remainder(x=w517, y=w519) -> (x-y*floor(x/y)=w516:i32)  [unwired: 1 out]
      n319 = Index Array(array=w518, index=w516) -> (element=w510:cluster{"t0":dbl, "dt":dbl, "Y":cdb[]})
      n320 = Get Queue Status(queue=w528, error in (no error)=w523) -> (queue out=w527:refnum<queue>, error out=w524:errorcluster, # elements in queue=w526:i32)  [unwired: 1 in, 5 out]
      n321 = Less?(x=w526, y=w520) -> (x < y?=w525:bool)
      n322 = Bundle("output complex waveform"=w510, w516) -> (w522:T22)  [unwired: 1 in]
      n323 = case shown="True" w525 {
        tunnel: w524 -> [w529 w537]
        tunnel: w527 -> [_ w536]
        tunnel: [w529 w535] -> w515
        tunnel: w522 -> [_ w534]
        tunnel: w517 -> [w531 w533]
        tunnel: [w531 w532] -> w521
        frame False {
          n324 = Wait Until Next ms Multiple(millisecond multiple=u32 0) -> ()  [unwired: 1 out]
        }
        frame True {
          n325 = Increment(x=w533) -> (x+1=w532:i32)
          n326 = Enqueue Element(queue=w536, element=w534, error in (no error)=w537) -> (error out=w535:errorcluster)  [unwired: 1 in, 2 out]
        }
      }
      n327 = control-ref of="Constellation Graph 4"() -> (w513:refnum<vi>)
      n328 = call <vilib>:"MT Format Constellation.vi"("waveform"=w510, "constellation reference"=w513, "samples per symbol"=w512, "autoscale"="autoscale 2") -> ("constellation graph"=→"Constellation Graph 4":T20)  [unwired: 1 in, 10 out]
    }
    n329 = call <instrlib>:"niUSRP Abort.vi"("session handle"=w79, "error in (no error)"=w43) -> ("session handle out"=w80:refnum<k15>, "error out"=w32:errorcluster)  [unwired: 12 in]
    n330 = call <instrlib>:"niUSRP Close Session.vi"("session handle"=w80, "error in (no error)"=w32) -> ()  [unwired: 13 in, 1 out]
    n331 = Write to Text File(file (use dialog)="file (use dialog) 3", text=w10) -> ()  [unwired: 2 in, 3 out]
    n332 = call <instrlib>:"niUSRP Abort.vi"("session handle"=w125, "error in (no error)"=w89) -> ("session handle out"=w126:refnum<k15>, "error out"=w127:errorcluster)  [unwired: 12 in]
    n333 = Write to Text File(file (use dialog)="file (use dialog) 4", text=w8) -> ()  [unwired: 2 in, 3 out]
    n334 = call <instrlib>:"niUSRP Close Session.vi"("session handle"=w126, "error in (no error)"=w127) -> ("error out"=w31:errorcluster)  [unwired: 13 in]
    "error out 3" <- w31
    n335 = Release Queue(queue=w170, error in (no error)=w169) -> (error out=w145:errorcluster)  [unwired: 3 out]
    n336 = call <instrlib>:"niUSRP Close Session.vi"("session handle"=w161, "error in (no error)"=w162) -> ("error out"=w144:errorcluster)  [unwired: 13 in]
    n337 = Merge Errors(w145, w144) -> (w30:errorcluster)
    "error out 4" <- w30
    n338 = Merge Errors(w32, w31, w30) -> (w29:errorcluster)
  }
